vi "ACT Panel.vi"() -> ()   [LabVIEW 2013]
uses:
  Type Defs/Final Output for Dispaly 2.ctl
  Type Defs/Alt Control.ctl
  Type Defs/Alt Digit 100 New.ctl
  Type Defs/All Timers.ctl
  Type Defs/Timer Control.ctl
  Altitude/Altitude.xctl
  Type Defs/Action Time.ctl
  Mode Control/Mode.xctl
  Type Defs/Alt Display Large.ctl
  MSR/VertMode/VertMode.xctl
  Type Defs/Named Final Output name list with 02.ctl
  Type Defs/Named Final Output name list ordered.ctl
  MSR/MultiVal Buffer Xctl/Multivalue Buffer.xctl
  Type Defs/CO2 Settings.ctl
  Type Defs/Output Values.ctl
  Type Defs/Output Switches.ctl
  Type Defs/AD Settings.ctl
  <vilib>/Platform/TimedLoop/XDataNode/timing_clust.ctl
  <vilib>/Platform/TimedLoop/XDataNode/nitl_modes.ctl
  <vilib>/Platform/TimedLoop/XDataNode/wakeup.ctl
  <vilib>/Utility/miscctls.llb/LVPointTypeDef.ctl
  Type Defs/Data Reading.ctl
  File/File.lvclass
  Output Timer/Output Timer.lvclass
  <vilib>/Utility/config.llb/Read Key (I32).vi
  <vilib>/Utility/config.llb/Read Key (Double).vi
  <vilib>/Utility/config.llb/Read Key (Boolean).vi
  Output Timer/Set Delay.vi
  <vilib>/Utility/config.llb/Write Key (I32).vi
  <vilib>/Utility/config.llb/Write Key (Double).vi
  <vilib>/Utility/config.llb/Write Key (Boolean).vi
  <vilib>/Platform/TimedLoop/XDataNode/XDataNode.xnode
  <vilib>/Platform/TimedLoop/XDataNode/XDNodeRunTimeDep.lvlib
  <vilib>/ptbypt/NI_PtbyPt.lvlib
  <vilib>/Utility/config.llb/NI_LVConfig.lvlib
panel:
  out "sysStat":bool caption="System Status"
  in  "Main Tabs":T1(tab)=enum."Hypoxic CO2 Settings"
  in  "Close":bool
  in  "Other Outputs":cluster{"Alarm":bool, "Heater":bool}
  out "CO2 ppm":u32(slide)=493 scale=0.0..10000.0
  out "Alt Dif":dbl(slide)=1604.2180978990014 scale=-1000.0..1000.0 scale format="%.1f"
  out "Final Output":T2
  in  "hypCO2":T3={"Run C1"={"A-1,  1"=inf, "A-3,  2"=inf, "A-4, 3"=9600.0, "A-5, 4"=8800.0, "ABCD-7, 5"=9800.0, "A-8, 6"=9800.0, "B-1,  7"=3400.0, "B-3, 8"=3400.0, "B-4,  9"=9600.0, "B-5, 10"=8800.0, "B-8, 11"=9800.0, "C-1, 12"=1800.0, "C-3, 13"=1800.0, "C-4, 14"=9600.0, "C-5,  15"=8800.0, "C-8, 16"=9800.0, "D-1, 17"=inf, "D-3, 18"=inf, "D-4,  19"=3400.0, "D-5,  20"=1800.0, "D-8,  21"=9800.0}, "Run C2"={"A-1,  1"=inf, "A-3,  2"=inf, "A-4, 3"=9500.0, "A-5, 4"=8600.0, "ABCD-7, 5"=9700.0, "A-8, 6"=9700.0, "B-1,  7"=3000.0, "B-3, 8"=3000.0, "B-4,  9"=9500.0, "B-5, 10"=8600.0, "B-8, 11"=9700.0, "C-1, 12"=1400.0, "C-3, 13"=1400.0, "C-4, 14"=9500.0, "C-5,  15"=8600.0, "C-8, 16"=9700.0, "D-1, 17"=inf, "D-3, 18"=inf, "D-4,  19"=3000.0, "D-5,  20"=1400.0, "D-8,  21"=9700.0}, "Hold C3"={"A-1,  1"=1800.0, "A-3,  2"=1800.0, "A-4, 3"=9000.0, "A-5, 4"=8800.0, "ABCD-7, 5"=9800.0, "A-8, 6"=9800.0, "B-1,  7"=3400.0, "B-3, 8"=3400.0, "B-4,  9"=9000.0, "B-5, 10"=8800.0, "B-8, 11"=9800.0, "C-1, 12"=1800.0, "C-3, 13"=1800.0, "C-4, 14"=9000.0, "C-5,  15"=8800.0, "C-8, 16"=9800.0, "D-1, 17"=inf, "D-3, 18"=1800.0, "D-4,  19"=3400.0, "D-5,  20"=1800.0, "D-8,  21"=9800.0}, "Hold C4"={"A-1,  1"=1400.0, "A-3,  2"=1400.0, "A-4, 3"=8800.0, "A-5, 4"=8600.0, "ABCD-7, 5"=9700.0, "A-8, 6"=9700.0, "B-1,  7"=3000.0, "B-3, 8"=3000.0, "B-4,  9"=8800.0, "B-5, 10"=8600.0, "B-8, 11"=9700.0, "C-1, 12"=1400.0, "C-3, 13"=1400.0, "C-4, 14"=8800.0, "C-5,  15"=8600.0, "C-8, 16"=9700.0, "D-1, 17"=inf, "D-3, 18"=1400.0, "D-4,  19"=3000.0, "D-5,  20"=1400.0, "D-8,  21"=9700.0}, "High CO2 Forces"={"A-1, 1"=TRUE, "A-3, 2"=TRUE, "A-4, 3"=FALSE, "A-5, 4"=TRUE, "ABCD-7, 5"=FALSE, "A-8, 6"=TRUE, "B-1,  7"=TRUE, "B-3, 8"=TRUE, "B-4, 9"=FALSE, "B-5, 10"=TRUE, "B-8,  11"=TRUE, "C-1, 12"=TRUE, "C-3, 13"=TRUE, "C-4,  14"=FALSE, "C-5,  15"=TRUE, "C-8, 16"=TRUE, "D-1, 17"=TRUE, "D-3, 18"=TRUE, "D-4, 19"=TRUE, "D-5,  20"=TRUE, "D-8,  21"=TRUE}}
  in  "hypAD":T6={"Set Point Force"={"A-1,  1"=inf, "A-3,  2"=inf, "A-4, 3"=inf, "A-5, 4"=5790.0, "ABCD-7, 5"=inf, "A-8, 6"=inf, "B-1,  7"=5790.0, "B-3, 8"=5790.0, "B-4,  9"=inf, "B-5, 10"=5790.0, "B-8, 11"=inf, "C-1, 12"=inf, "C-3, 13"=inf, "C-4, 14"=inf, "C-5,  15"=5790.0, "C-8, 16"=inf, "D-1, 17"=inf, "D-3, 18"=inf, "D-4,  19"=5790.0, "D-5,  20"=5790.0, "D-8,  21"=inf}, "Run A1"={"A-1,  1"=inf, "A-3,  2"=inf, "A-4, 3"=3.0, "A-5, 4"=inf, "ABCD-7, 5"=67.0, "A-8, 6"=630.0, "B-1,  7"=-30.0, "B-3, 8"=-30.0, "B-4,  9"=3.0, "B-5, 10"=inf, "B-8, 11"=630.0, "C-1, 12"=-60.0, "C-3, 13"=-60.0, "C-4, 14"=3.0, "C-5,  15"=inf, "C-8, 16"=630.0, "D-1, 17"=inf, "D-3, 18"=inf, "D-4,  19"=-30.0, "D-5,  20"=-60.0, "D-8,  21"=630.0}, "Run A2"={"A-1,  1"=inf, "A-3,  2"=inf, "A-4, 3"=-3.0, "A-5, 4"=inf, "ABCD-7, 5"=60.0, "A-8, 6"=610.0, "B-1,  7"=-100.0, "B-3, 8"=-100.0, "B-4,  9"=-3.0, "B-5, 10"=inf, "B-8, 11"=610.0, "C-1, 12"=-120.0, "C-3, 13"=-120.0, "C-4, 14"=-3.0, "C-5,  15"=inf, "C-8, 16"=610.0, "D-1, 17"=inf, "D-3, 18"=inf, "D-4,  19"=-100.0, "D-5,  20"=-120.0, "D-8,  21"=610.0}, "Hold A3"={"A-1,  1"=0.0, "A-3,  2"=0.0, "A-4, 3"=3.0, "A-5, 4"=inf, "ABCD-7, 5"=67.0, "A-8, 6"=630.0, "B-1,  7"=-150.0, "B-3, 8"=-150.0, "B-4,  9"=3.0, "B-5, 10"=inf, "B-8, 11"=630.0, "C-1, 12"=-300.0, "C-3, 13"=-300.0, "C-4, 14"=3.0, "C-5,  15"=inf, "C-8, 16"=630.0, "D-1, 17"=inf, "D-3, 18"=0.0, "D-4,  19"=-150.0, "D-5,  20"=-300.0, "D-8,  21"=630.0}, "Hold A4"={"A-1,  1"=-150.0, "A-3,  2"=-150.0, "A-4, 3"=-3.0, "A-5, 4"=inf, "ABCD-7, 5"=60.0, "A-8, 6"=610.0, "B-1,  7"=-250.0, "B-3, 8"=-250.0, "B-4,  9"=-3.0, "B-5, 10"=inf, "B-8, 11"=610.0, "C-1, 12"=-500.0, "C-3, 13"=-500.0, "C-4, 14"=-3.0, "C-5,  15"=inf, "C-8, 16"=610.0, "D-1, 17"=inf, "D-3, 18"=-150.0, "D-4,  19"=-250.0, "D-5,  20"=-500.0, "D-8,  21"=610.0}, "High AD Diff "={"A-1, 1"=FALSE, "A-3, 2"=FALSE, "A-4, 3"=FALSE, "A-5, 4"=TRUE, "ABCD-7, 5"=FALSE, "A-8, 6"=TRUE, "B-1,  7"=FALSE, "B-3, 8"=FALSE, "B-4, 9"=FALSE, "B-5, 10"=TRUE, "B-8,  11"=TRUE, "C-1, 12"=FALSE, "C-3, 13"=FALSE, "C-4,  14"=FALSE, "C-5,  15"=TRUE, "C-8, 16"=TRUE, "D-1, 17"=FALSE, "D-3, 18"=FALSE, "D-4, 19"=FALSE, "D-5,  20"=FALSE, "D-8,  21"=TRUE}, "Delay S"={"A-1,  1"=30.0, "A-3,  2"=30.0, "A-4, 3"=1.0, "A-5, 4"=1.0, "ABCD-7, 5"=1.0, "A-8, 6"=1.0, "B-1,  7"=30.0, "B-3, 8"=30.0, "B-4,  9"=1.0, "B-5, 10"=1.0, "B-8, 11"=1.0, "C-1, 12"=30.0, "C-3, 13"=30.0, "C-4, 14"=1.0, "C-5,  15"=1.0, "C-8, 16"=1.0, "D-1, 17"=1.0, "D-3, 18"=30.0, "D-4,  19"=30.0, "D-5,  20"=30.0, "D-8,  21"=1.0}}
  in  "hyperCO2":T3={"Run C1"={"A-1,  1"=inf, "A-3,  2"=inf, "A-4, 3"=9600.0, "A-5, 4"=8800.0, "ABCD-7, 5"=9800.0, "A-8, 6"=9800.0, "B-1,  7"=3400.0, "B-3, 8"=3400.0, "B-4,  9"=9600.0, "B-5, 10"=8800.0, "B-8, 11"=9800.0, "C-1, 12"=1800.0, "C-3, 13"=1800.0, "C-4, 14"=9600.0, "C-5,  15"=8800.0, "C-8, 16"=9800.0, "D-1, 17"=inf, "D-3, 18"=inf, "D-4,  19"=3400.0, "D-5,  20"=1800.0, "D-8,  21"=9800.0}, "Run C2"={"A-1,  1"=inf, "A-3,  2"=inf, "A-4, 3"=9500.0, "A-5, 4"=8600.0, "ABCD-7, 5"=9700.0, "A-8, 6"=9700.0, "B-1,  7"=3000.0, "B-3, 8"=3000.0, "B-4,  9"=9500.0, "B-5, 10"=8600.0, "B-8, 11"=9700.0, "C-1, 12"=1400.0, "C-3, 13"=1400.0, "C-4, 14"=9500.0, "C-5,  15"=8600.0, "C-8, 16"=9700.0, "D-1, 17"=inf, "D-3, 18"=inf, "D-4,  19"=3000.0, "D-5,  20"=1400.0, "D-8,  21"=9700.0}, "Hold C3"={"A-1,  1"=1800.0, "A-3,  2"=1800.0, "A-4, 3"=9000.0, "A-5, 4"=8800.0, "ABCD-7, 5"=9800.0, "A-8, 6"=9800.0, "B-1,  7"=3400.0, "B-3, 8"=3400.0, "B-4,  9"=9000.0, "B-5, 10"=8800.0, "B-8, 11"=9800.0, "C-1, 12"=1800.0, "C-3, 13"=1800.0, "C-4, 14"=9000.0, "C-5,  15"=8800.0, "C-8, 16"=9800.0, "D-1, 17"=inf, "D-3, 18"=1800.0, "D-4,  19"=3400.0, "D-5,  20"=1800.0, "D-8,  21"=9800.0}, "Hold C4"={"A-1,  1"=1400.0, "A-3,  2"=1400.0, "A-4, 3"=8800.0, "A-5, 4"=8600.0, "ABCD-7, 5"=9700.0, "A-8, 6"=9700.0, "B-1,  7"=3000.0, "B-3, 8"=3000.0, "B-4,  9"=8800.0, "B-5, 10"=8600.0, "B-8, 11"=9700.0, "C-1, 12"=1400.0, "C-3, 13"=1400.0, "C-4, 14"=8800.0, "C-5,  15"=8600.0, "C-8, 16"=9700.0, "D-1, 17"=inf, "D-3, 18"=1400.0, "D-4,  19"=3000.0, "D-5,  20"=1400.0, "D-8,  21"=9700.0}, "High CO2 Forces"={"A-1, 1"=TRUE, "A-3, 2"=TRUE, "A-4, 3"=FALSE, "A-5, 4"=TRUE, "ABCD-7, 5"=FALSE, "A-8, 6"=TRUE, "B-1,  7"=TRUE, "B-3, 8"=TRUE, "B-4, 9"=FALSE, "B-5, 10"=TRUE, "B-8,  11"=TRUE, "C-1, 12"=TRUE, "C-3, 13"=TRUE, "C-4,  14"=FALSE, "C-5,  15"=TRUE, "C-8, 16"=TRUE, "D-1, 17"=TRUE, "D-3, 18"=TRUE, "D-4, 19"=TRUE, "D-5,  20"=TRUE, "D-8,  21"=TRUE}}
  in  "hyperAD":T6={"Set Point Force"={"A-1,  1"=inf, "A-3,  2"=inf, "A-4, 3"=inf, "A-5, 4"=5790.0, "ABCD-7, 5"=inf, "A-8, 6"=inf, "B-1,  7"=5790.0, "B-3, 8"=5790.0, "B-4,  9"=inf, "B-5, 10"=5790.0, "B-8, 11"=inf, "C-1, 12"=inf, "C-3, 13"=inf, "C-4, 14"=inf, "C-5,  15"=5790.0, "C-8, 16"=inf, "D-1, 17"=inf, "D-3, 18"=inf, "D-4,  19"=5790.0, "D-5,  20"=5790.0, "D-8,  21"=inf}, "Run A1"={"A-1,  1"=inf, "A-3,  2"=inf, "A-4, 3"=3.0, "A-5, 4"=inf, "ABCD-7, 5"=67.0, "A-8, 6"=630.0, "B-1,  7"=-30.0, "B-3, 8"=-30.0, "B-4,  9"=3.0, "B-5, 10"=inf, "B-8, 11"=630.0, "C-1, 12"=-60.0, "C-3, 13"=-60.0, "C-4, 14"=3.0, "C-5,  15"=inf, "C-8, 16"=630.0, "D-1, 17"=inf, "D-3, 18"=inf, "D-4,  19"=-30.0, "D-5,  20"=-60.0, "D-8,  21"=630.0}, "Run A2"={"A-1,  1"=inf, "A-3,  2"=inf, "A-4, 3"=-3.0, "A-5, 4"=inf, "ABCD-7, 5"=60.0, "A-8, 6"=610.0, "B-1,  7"=-100.0, "B-3, 8"=-100.0, "B-4,  9"=-3.0, "B-5, 10"=inf, "B-8, 11"=610.0, "C-1, 12"=-120.0, "C-3, 13"=-120.0, "C-4, 14"=-3.0, "C-5,  15"=inf, "C-8, 16"=610.0, "D-1, 17"=inf, "D-3, 18"=inf, "D-4,  19"=-100.0, "D-5,  20"=-120.0, "D-8,  21"=610.0}, "Hold A3"={"A-1,  1"=0.0, "A-3,  2"=0.0, "A-4, 3"=3.0, "A-5, 4"=inf, "ABCD-7, 5"=67.0, "A-8, 6"=630.0, "B-1,  7"=-150.0, "B-3, 8"=-150.0, "B-4,  9"=3.0, "B-5, 10"=inf, "B-8, 11"=630.0, "C-1, 12"=-300.0, "C-3, 13"=-300.0, "C-4, 14"=3.0, "C-5,  15"=inf, "C-8, 16"=630.0, "D-1, 17"=inf, "D-3, 18"=0.0, "D-4,  19"=-150.0, "D-5,  20"=-300.0, "D-8,  21"=630.0}, "Hold A4"={"A-1,  1"=-150.0, "A-3,  2"=-150.0, "A-4, 3"=-3.0, "A-5, 4"=inf, "ABCD-7, 5"=60.0, "A-8, 6"=610.0, "B-1,  7"=-250.0, "B-3, 8"=-250.0, "B-4,  9"=-3.0, "B-5, 10"=inf, "B-8, 11"=610.0, "C-1, 12"=-500.0, "C-3, 13"=-500.0, "C-4, 14"=-3.0, "C-5,  15"=inf, "C-8, 16"=610.0, "D-1, 17"=inf, "D-3, 18"=-150.0, "D-4,  19"=-250.0, "D-5,  20"=-500.0, "D-8,  21"=610.0}, "High AD Diff "={"A-1, 1"=FALSE, "A-3, 2"=FALSE, "A-4, 3"=FALSE, "A-5, 4"=TRUE, "ABCD-7, 5"=FALSE, "A-8, 6"=TRUE, "B-1,  7"=FALSE, "B-3, 8"=FALSE, "B-4, 9"=FALSE, "B-5, 10"=TRUE, "B-8,  11"=TRUE, "C-1, 12"=FALSE, "C-3, 13"=FALSE, "C-4,  14"=FALSE, "C-5,  15"=TRUE, "C-8, 16"=TRUE, "D-1, 17"=FALSE, "D-3, 18"=FALSE, "D-4, 19"=FALSE, "D-5,  20"=FALSE, "D-8,  21"=TRUE}, "Delay S"={"A-1,  1"=30.0, "A-3,  2"=30.0, "A-4, 3"=1.0, "A-5, 4"=1.0, "ABCD-7, 5"=1.0, "A-8, 6"=1.0, "B-1,  7"=30.0, "B-3, 8"=30.0, "B-4,  9"=1.0, "B-5, 10"=1.0, "B-8, 11"=1.0, "C-1, 12"=30.0, "C-3, 13"=30.0, "C-4, 14"=1.0, "C-5,  15"=1.0, "C-8, 16"=1.0, "D-1, 17"=1.0, "D-3, 18"=30.0, "D-4,  19"=30.0, "D-5,  20"=30.0, "D-8,  21"=1.0}}
  in  "Main States":T7(tab)
  out "altDisp1":dbl format="%#.0f"
  out "altDisp1 2":dbl format="%#.0f"
  out "Heading 3":string="Current Effective Altitude in  Feet"
  in  "Mode 1":enum8{"Off", "Stby", "Hold", "Run"}(xcontrol)=enum."Stby"
  in  "Confirm Now 2":bool
  out "CO2_1":sgl caption="Carbon Dioxide  %" format="%.3f"
  in  "ALT SET 2":T8 {"Alt Digit 100" min=0 max=9 step=1; "Alt Digit 100" min=0 max=9 step=1; "Alt Digit 100" min=0 max=9 step=1; "Alt Digit 100" min=0 max=9 step=1; "Alt Digit 100" min=0 max=9 step=1}
  out "altDisp2":T10 caption="ALT DISPLAY 2" format="%#.0f"
  out "Heading 2":string="Current Effective Altitude in  Feet"
  in  "dimmer":i8(slide) scale=0.0..100.0
  out "CO2Buffer":cluster{"Time":timestamp, "Val":dbl[]}(xcontrol)
  out "pAltitude":cluster{"Time":timestamp, "Val":dbl[]}(xcontrol)
  out "Temp C":sgl=26.28
  out "Press mB":sgl=833.25
  out "CO2_0":sgl=0.0493 caption="CO2%\n %" format="%.3g"
  in  "Confirm Now":bool
  in  "ALT SET":T8 {"Alt Digit 100" min=0 max=9 step=1; "Alt Digit 100" min=0 max=9 step=1; "Alt Digit 100" min=0 max=9 step=1; "Alt Digit 100" min=0 max=9 step=1; "Alt Digit 100" min=0 max=9 step=1}
  out "Altitude":sgl format="%#.0f"
  out "O2%":sgl=20.9793 format="%.1f"
  out "Units":string="F\ne\ne\nt"
  in  "Mode":enum8{"Off", "Stby", "Hold", "Run"}(xcontrol)=enum."Stby"
  out "Final  Output Names":T11={"A-1,  1"="Main", "A-3,  2"="Main", "A-4, 3"="Recircirculation", "A-5, 4"="Scrubber", "A-7, 5"="Oxygen", "A-8, 6"="Vent", "B-1,  7"="Boost A", "B-3, 8"="Boost A", "B-4,  9"="Recircirculation", "B-5, 10"="Scrubber", "B-8, 11"="Vent", "C-1, 12"="Boost B", "C-3, 13"="Boost B", "C-4, 14"="Recircirculation", "C-5,  15"="Scrubber", "C-8, 16"="Vent", "D-1, 17"="Main", "D-3, 18"="Boost A", "D-4,  19"="Boost B", "D-5,  20"="Vent", "D-8,  21"="Vent 2", "B-7"="Oxygen", "C-7"="Oxygen", "D-7"="Oxygen", "A-1"=FALSE, "A-3"=FALSE, "A-4"=FALSE, "A-5"=FALSE, "A-7"=FALSE, "A-8"=FALSE, "B-1"=FALSE, "B-3"=FALSE, "B-4"=FALSE, "B-5"=FALSE, "B-7"=FALSE, "B-8"=FALSE, "C-1"=FALSE, "C-3"=FALSE, "C-4"=FALSE, "C-5"=FALSE, "C-7"=FALSE, "C-8"=FALSE, "D-1"=FALSE, "D-3"=FALSE, "D-4"=FALSE, "D-5"=FALSE, "D-7"=FALSE, "D-8"=FALSE}
  out "Time":timestamp caption="Controller\nTime" format="%<%H:%M:%S\n%m/%d/%y>T"
  in  "Timers":T12 {"Timer 4"."Action Time" format="%<%H:%M>t"; "Timer 3"."Action Time" format="%<%H:%M>t"; "Timer 2"."Action Time" format="%<%H:%M>t"; "Timer"."Action Time" format="%<%H:%M>t"}
  in  "Shutdown":bool
  out "maxO2":dbl caption="Max O2" format="%.1f"
  out "minAlt":dbl caption="Minimum Altitude"
  out "onBatt":bool caption="Plugged in?"
  out "estBattLeft":u8(slide) caption="Estimated Battery Life" scale=0.0..100.0
  in  "eCode":bool
  in  "silence":bool
  out "senseConn":bool caption="Sensor Connection"
  out "High O2 Level":bool
  out "Altitude":bool
  out "Low O2 Level":bool
  out "CO2 Level":bool
  in  "writetofile":bool
  out "Sensor Error":bool
  out "Calibrate":bool
  out "meanDiff":dbl caption="Mean O2 Difference"
  out "Calibrating":bool
  in  "Enter or Exit Setup":bool
  in  "reset":bool
  in  "Set Point Alt":i32 min=0 max=10000 step=1
  in  "Level 0":T15 {"Time Offset (h)" min=-12.0 max=12.0 step=1.0}
  in  "Level 1":T16
  in  "Level 2":T17
  in  "Level 3":T19={"Final  Output Names "={"A-1, 1"="Main", "A-3, 2"="Main", "A-4, 3"="Recircirculation", "A-5, 4"="Scrubber", "A-7, 5"="Oxygen", "A-8, 6"="Vent", "B-1,  7"="Boost A", "B-3, 8"="Boost A", "B-4, 9"="Recircirculation", "B-5, 10"="Scrubber", "B-8, 11"="Vent", "C-1, 12"="Boost B", "C-3, 13"="Boost B", "C-4, 14"="Recircirculation", "C-5,  15"="Scrubber", "C-8, 16"="Vent", "D-1, 17"="Main", "D-3, 18"="Boost A", "D-4,  19"="Boost B", "D-5,  20"="Vent", "D-8,  21"="Vent 2"}, " Setup Tables Visible"=FALSE, "Load Names"=FALSE, "Save Names"=FALSE, "maxAltSP"=0.0, "Alarm Points"={"CalLimit"=500.0, "SenseLimit"=1000.0, "CO2Lim"=1.0, "AltLim"=100000.0, "O2 Low"=100.0, "O2 High"=100.0}, "Stop"=FALSE, "O2-1 (%)"=0.0, "O2-2 (%)"=0.0, "Buffer"=0.0} {"Buffer" min=0.0 max=1.0 format="%7.4f"; "O2-2 (%)" format="%7.4f"; "O2-1 (%)" format="%7.4f"}
  out "SN#":string
  out "Version":string
  out "locElev":dbl=1449.1019287109375 caption="Pressure Compensated \nLocal Elevation"
  out "altSp":dbl
  out "codelapse":bool
  # "Channel A"
  # "Channel B"
  # "Channel C"
  # "Channel D"
  # "Channel A"
  # "Channel B"
  # "Channel C"
  # "Channel D"
  # "1"
  # "1"
  # "1"
  # "1"
  # "CAT v153"
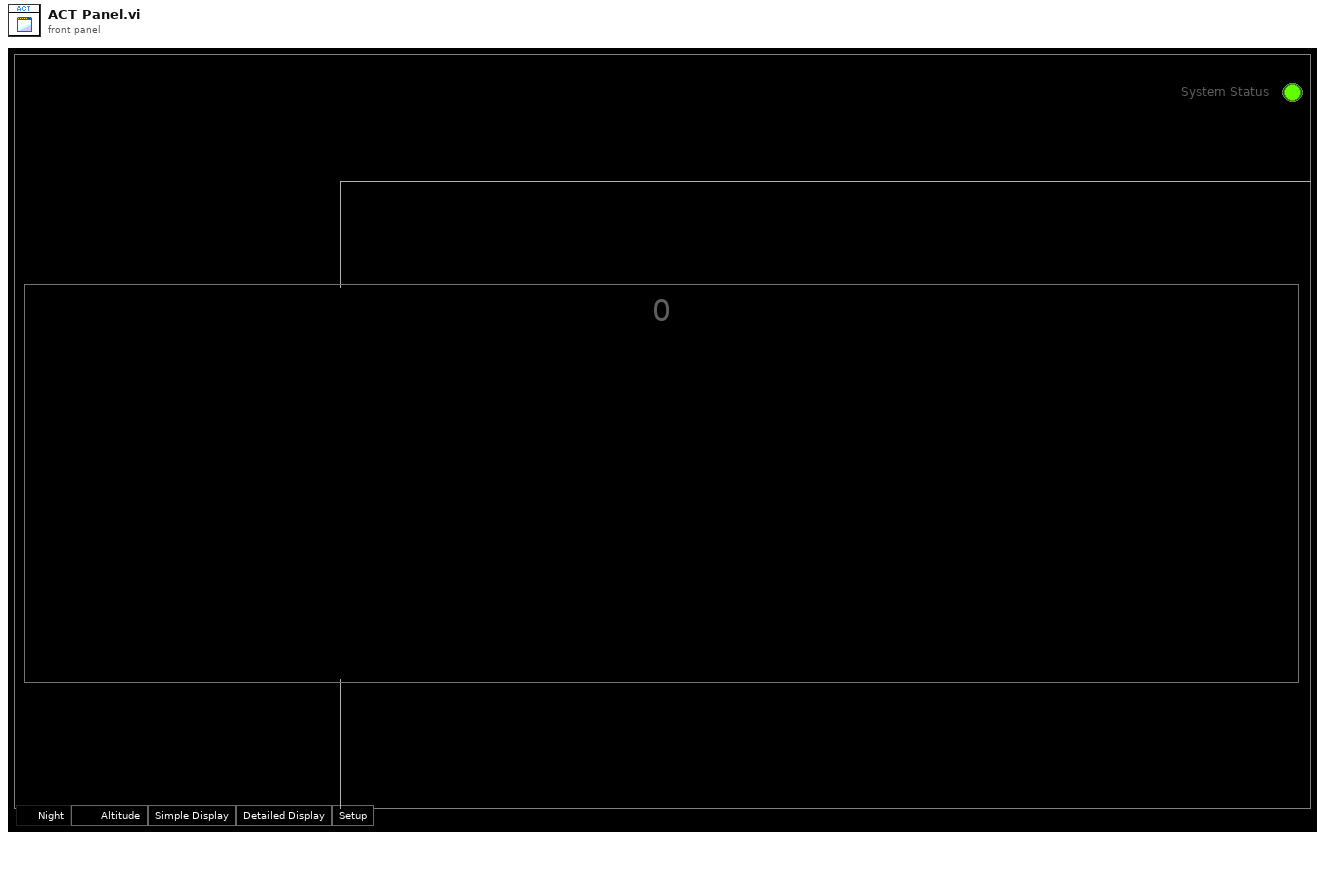
[diagram p1: front panel]
types:
  T1 = enum32{"Inputs and Controls", "CO2 and AD Outputs", "Hypoxic CO2 Settings", "Hypoxic AD Settings", "Hyperoxic CO2 Settings", "Hyperoxic AD Settings"}
  T2 = typedef "Final Output for Dispaly 2.ctl" = cluster{"A-1,  1":bool, "A-3,  2":bool, "A-4, 3":bool, "A-5, 4":bool, "ABCD-7, 5":bool, "A-8, 6":bool, "B-1,  7":bool, "B-3, 8":bool, "B-4,  9":bool, "B-5, 10":bool, "B-8, 11":bool, "C-1, 12":bool, "C-3, 13":bool, "C-4, 14":bool, "C-5,  15":bool, "C-8, 16":bool, "D-1, 17":bool, "D-3, 18":bool, "D-4,  19":bool, "D-5,  20":bool, "D-8,  21":bool}
  T3 = typedef "CO2 Settings.ctl" = cluster{"Run C1":T4, "Run C2":T4, "Hold C3":T4, "Hold C4":T4, "High CO2 Forces":T5}
  T4 = typedef "Output Values.ctl" = cluster{"A-1,  1":dbl, "A-3,  2":dbl, "A-4, 3":dbl, "A-5, 4":dbl, "ABCD-7, 5":dbl, "A-8, 6":dbl, "B-1,  7":dbl, "B-3, 8":dbl, "B-4,  9":dbl, "B-5, 10":dbl, "B-8, 11":dbl, "C-1, 12":dbl, "C-3, 13":dbl, "C-4, 14":dbl, "C-5,  15":dbl, "C-8, 16":dbl, "D-1, 17":dbl, "D-3, 18":dbl, "D-4,  19":dbl, "D-5,  20":dbl, "D-8,  21":dbl}
  T5 = typedef "Output Switches.ctl" = cluster{"A-1, 1":bool, "A-3, 2":bool, "A-4, 3":bool, "A-5, 4":bool, "ABCD-7, 5":bool, "A-8, 6":bool, "B-1,  7":bool, "B-3, 8":bool, "B-4, 9":bool, "B-5, 10":bool, "B-8,  11":bool, "C-1, 12":bool, "C-3, 13":bool, "C-4,  14":bool, "C-5,  15":bool, "C-8, 16":bool, "D-1, 17":bool, "D-3, 18":bool, "D-4, 19":bool, "D-5,  20":bool, "D-8,  21":bool}
  T6 = typedef "AD Settings.ctl" = cluster{"Set Point Force":T4, "Run A1":T4, "Run A2":T4, "Hold A3":T4, "Hold A4":T4, "High AD Diff ":T5, "Delay S":T4}
  T7 = enum32{"     Night", "       Altitude ", "Simple Display", "Detailed Display", "Timers", "Setup"}
  T8 = typedef "Alt Control.ctl" = cluster{"Alt Digit 100":T9, "Alt Digit 100":T9, "Alt Digit 100":T9, "Alt Digit 100":T9, "Alt Digit 100":T9}
  T9 = typedef "Alt Digit 100 New.ctl" = i8
  T10 = typedef "Alt Display Large.ctl" = sgl
  T11 = typedef "Named Final Output name list with 02.ctl" = cluster{"A-1,  1":string, "A-3,  2":string, "A-4, 3":string, "A-5, 4":string, "A-7, 5":string, "A-8, 6":string, "B-1,  7":string, "B-3, 8":string, "B-4,  9":string, "B-5, 10":string, "B-8, 11":string, "C-1, 12":string, "C-3, 13":string, "C-4, 14":string, "C-5,  15":string, "C-8, 16":string, "D-1, 17":string, "D-3, 18":string, "D-4,  19":string, "D-5,  20":string, "D-8,  21":string, "B-7":string, "C-7":string, "D-7":string, "A-1":bool, "A-3":bool, "A-4":bool, "A-5":bool, "A-7":bool, "A-8":bool, "B-1":bool, "B-3":bool, "B-4":bool, "B-5":bool, "B-7":bool, "B-8":bool, "C-1":bool, "C-3":bool, "C-4":bool, "C-5":bool, "C-7":bool, "C-8":bool, "D-1":bool, "D-3":bool, "D-4":bool, "D-5":bool, "D-7":bool, "D-8":bool}
  T12 = typedef "All Timers.ctl" = cluster{"Timer":T13, "Timer 2":T13, "Timer 3":T13, "Timer 4":T13}
  T13 = typedef "Timer Control.ctl" = cluster{"Sun":bool, "Timer":bool, "Altitude":sgl, "Action Time":T14, "Mon":bool, "Tues":bool, "Wed":bool, "Thur":bool, "Fri":bool, "Sat":bool, "Mode":enum8{"Off", "Stby", "Hold", "Run"}}
  T14 = typedef "Action Time.ctl" = dbl
  T15 = cluster{"Time Offset (h)":dbl, "Demo Mode?":bool}
  T16 = cluster{"ALT Window ON/OFF":bool, "Feet OFF/ Meters ON":bool}
  T17 = cluster{"West ON/Std OFF":bool, "Enter Calibration":bool, "Max Altitude":dbl, "Alt Points":u32, "CO2 Points":u32}
  T18 = typedef "Named Final Output name list ordered.ctl" = cluster{"A-1, 1":string, "A-3, 2":string, "A-4, 3":string, "A-5, 4":string, "A-7, 5":string, "A-8, 6":string, "B-1,  7":string, "B-3, 8":string, "B-4, 9":string, "B-5, 10":string, "B-8, 11":string, "C-1, 12":string, "C-3, 13":string, "C-4, 14":string, "C-5,  15":string, "C-8, 16":string, "D-1, 17":string, "D-3, 18":string, "D-4,  19":string, "D-5,  20":string, "D-8,  21":string}
  T19 = cluster{"Final  Output Names ":T18, " Setup Tables Visible":bool, "Load Names":bool, "Save Names":bool, "maxAltSP":sgl, "Alarm Points":cluster{"CalLimit":sgl, "SenseLimit":sgl, "CO2Lim":sgl, "AltLim":sgl, "O2 Low":sgl, "O2 High":sgl}, "Stop":bool, "O2-1 (%)":dbl, "O2-2 (%)":dbl, "Buffer":dbl}
  T20 = typedef "LVPointTypeDef.ctl" = cluster{"Horizontal":i16, "Vertical":i16}
  T21 = cluster{"Heading":string, "Altitude":dbl, "Visible?":bool}
  T22 = typedef "XDNodeRunTimeDep.lvlib/timing_clust.ctl" = cluster{"Expected End [f-1]":u64, "Actual End [f-1]":u64, "Finished Late? [f-1]":bool, "Expected End [i-1]":u64, "Actual End [i-1]":u64, "Finished Late? [i-1]":bool, "Expected Start [i]":u64, "Actual Start [i]":u64, "Expected Start [f]":u64, "Actual Start [f]":u64, "Source Name":string, "Structure Name":string, "Period":i64, "Deadline":i64, "Offset":i64, "Start":i64, "Priority":i32, "Timeout":i32, "Mode":T23, "Wakeup Reason":T24, "Error":errorcluster, "Source Type":string, "Secondary Source Type":string, "Global End Time":u64, "Global Start Time":u64, "Frame Duration":u64, "Iteration Duration":u64, "Assigned CPU":i32, "I/O Scan Engine Mode":u32}
  T23 = typedef "XDNodeRunTimeDep.lvlib/nitl_modes.ctl" = enum32{"No Change", "Process missed periods, maintain original phase", "Discard missed periods, maintain original phase", "Process missed periods, ignore original phase", "Discard missed periods, ignore original phase"}
  T24 = typedef "XDNodeRunTimeDep.lvlib/wakeup.ctl" = enum32{"Normal", "Aborted", "Asynchronous wakeup", "Timing source error", "Timed loop error", "Timeout"}
  T25 = enum32{"Invalid", "Standard", "Closed", "Hidden", "Minimized", "Maximized"}
  T26 = typedef "Data Reading.ctl" = cluster{"Date":string, "Time":string, "CO2- ppm":u32, "Last Ctrl Word":u32, "O2-1 ppm":u32, "O2-2 ppm":u32, "Temp MB":sgl, "Temp Sensor Module":sgl, "Press mB":sgl}
  T27 = typedef "NI_LVConfig.lvlib/Config Data RefNum.ctl" = refnum<k1>
  T28 = enum8{"Enabled", "Disabled", "Disabled and Grayed Out"}
  T29 = cluster{"[0]":i8, "[1]":i8, "[2]":i8, "[3]":i8, "[4]":i8}
  T30 = cluster{"Level 1 Password":string, "Level 2 Password":string, "Level 3 Password":string}
  T31 = cluster{"CalLimit":dbl, "SenseLimit":dbl, "CO2Lim":dbl, "AltLim":dbl, "O2 Low":dbl, "O2 High":dbl}
  T32 = cluster{"Pointers":i32[], "Dates":dbl[], "Keys":string[], "Key Valid?":bool[], "Date Exceeded":bool[]}
  T33 = typedef "LVRectTypeDef.ctl" = cluster{"Left":i16, "Top":i16, "Right":i16, "Bottom":i16}
  T34 = cluster{"Mode":refnum<vi>, "ALT SET":refnum<vi>, "Confirm Now":refnum<vi>}
  T35 = cluster{"Main 1":bool, "Main 2":bool, "Recirc  3":bool, "Boost A 7":bool, "Recirc  9":bool, "Scrub 4":bool, "Scrub 10":bool, "O2 5":bool, "Vent 6":bool, "Boost A 8":bool, "Vent 11":bool, "Boost B 12":bool, "Boost B 13":bool, "Recirc 14":bool, "Scrub 15":bool, "Vent 16":bool, "Main 17":bool, "Boost A 18":bool, "Boost B 19":bool, "Boost F 20":bool, "Vent 2 21":bool}
  T36 = cluster{"A-1,  1":bool, "A-3,  2":bool, "A-4, 3":bool, "A-5, 4":bool, "ABCD-7, 5":bool, "A-8, 6":bool, "B-1,  7":bool, "B-3, 8":bool, "B-4,  9":bool, "B-5, 10":bool, "B-8, 11":bool, "C-1, 12":bool, "C-3, 13":bool, "C-4, 14":bool, "C-5,  15":bool, "C-8, 16":bool, "D-1, 17":bool, "D-3, 18":bool, "D-4,  19":bool, "D-5,  20":bool, "D-8,  21":bool}
  T37 = cluster{bool, bool, bool, bool, bool, bool, bool, bool, bool, bool, bool, bool, bool, bool, bool, bool, bool, bool, bool, bool, bool}
  T38 = cluster{"[0]":bool, "[1]":bool, "[2]":bool, "[3]":bool, "[4]":bool, "[5]":bool, "[6]":bool, "[7]":bool, "[8]":bool, "[9]":bool, "[10]":bool, "[11]":bool, "[12]":bool, "[13]":bool, "[14]":bool, "[15]":bool, "[16]":bool, "[17]":bool, "[18]":bool, "[19]":bool, "[20]":bool}
  T39 = cluster{"Date":string, "Time":string, "CO2- ppm":u32, "Last Ctrl Word":u32, "O2-1 ppm":u32, "O2-2 ppm":u32, "Temp MB":sgl, "Temp Sensor Module":sgl, "Press mB":sgl}
  T40 = cluster{"Set Point Force":T4, "Run A1":T4, "Run A2":T4, "Hold A3":T4, "Hold A4":T4}
  T41 = cluster{"Set Point Force":T4, "Run A1":T4, "Run A2":T4, "Hold A3":T4, "Hold A4":T4, "AltLim":sgl, "Set Point Alt":i32, "Value":sgl, "Value":dbl}
  T42 = cluster{"Set Point Force":T4, "Run A1":T4, "Run A2":T4, "Hold A3":T4, "Hold A4":T4, "AltLim":dbl, "Set Point Alt":dbl, "Value":dbl, "Value":dbl}
  T43 = cluster{"CalLimit":sgl, "SenseLimit":sgl, "CO2Lim":sgl, "AltLim":sgl, "O2 Low":sgl, "O2 High":sgl}
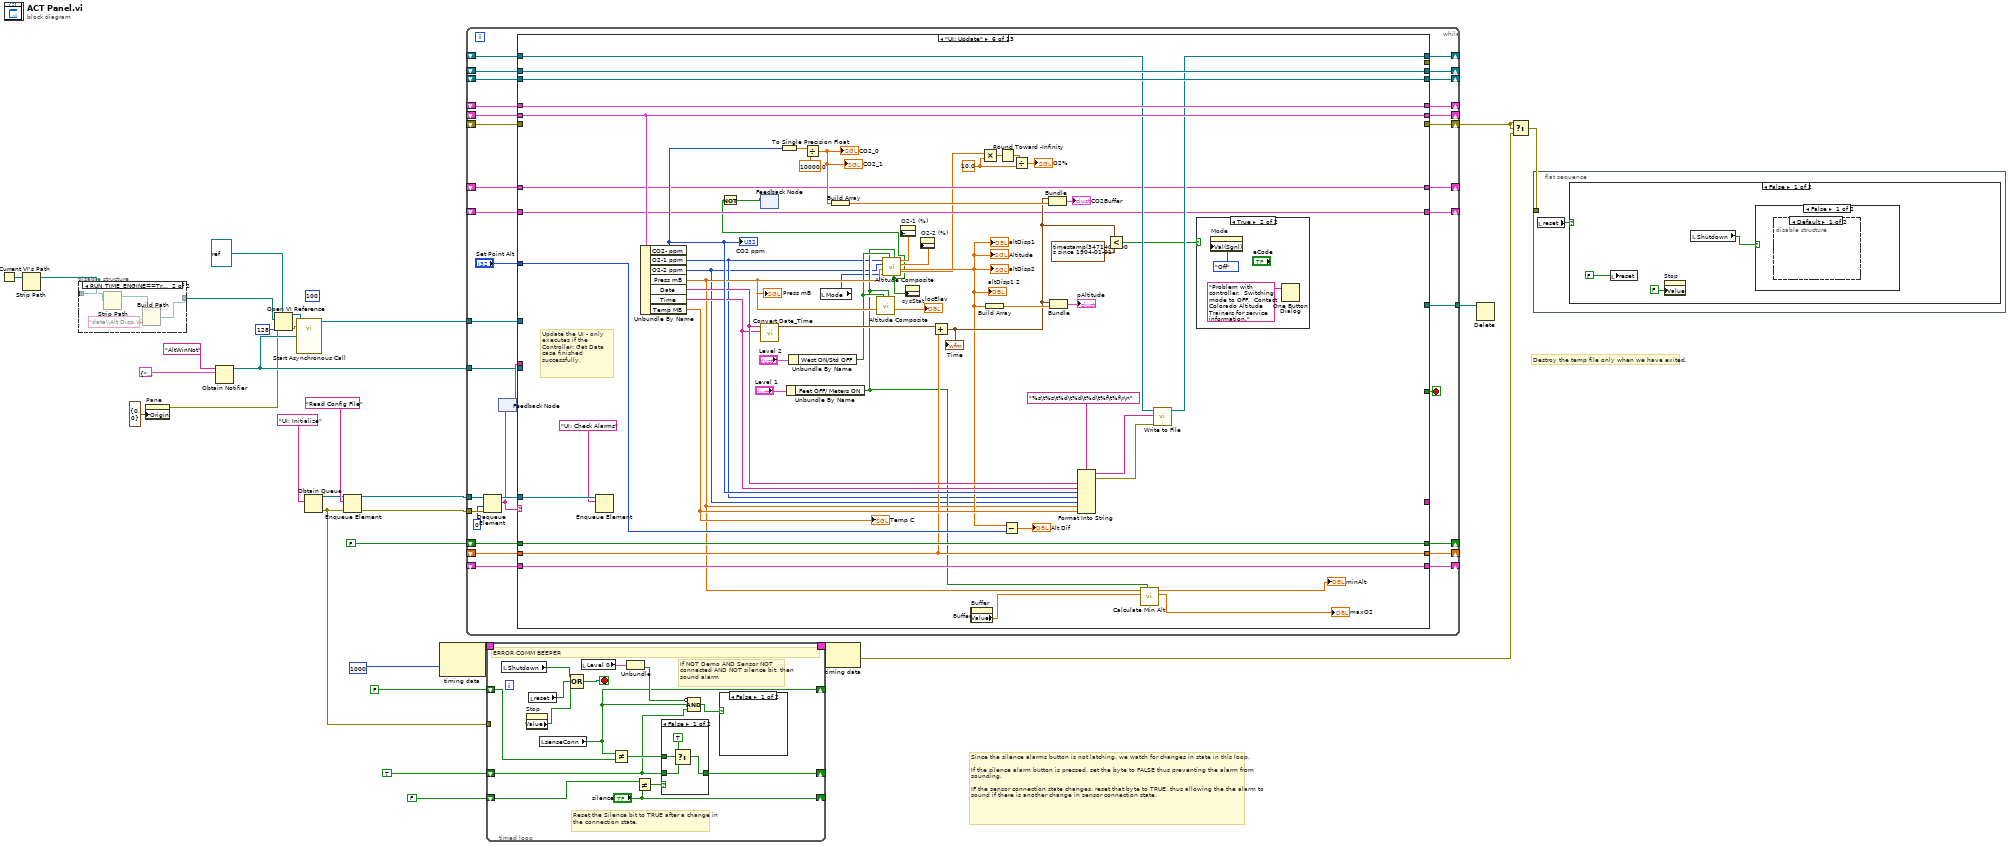
[diagram p0: block diagram]
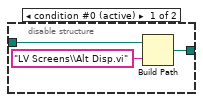
[diagram p2: hidden frame]
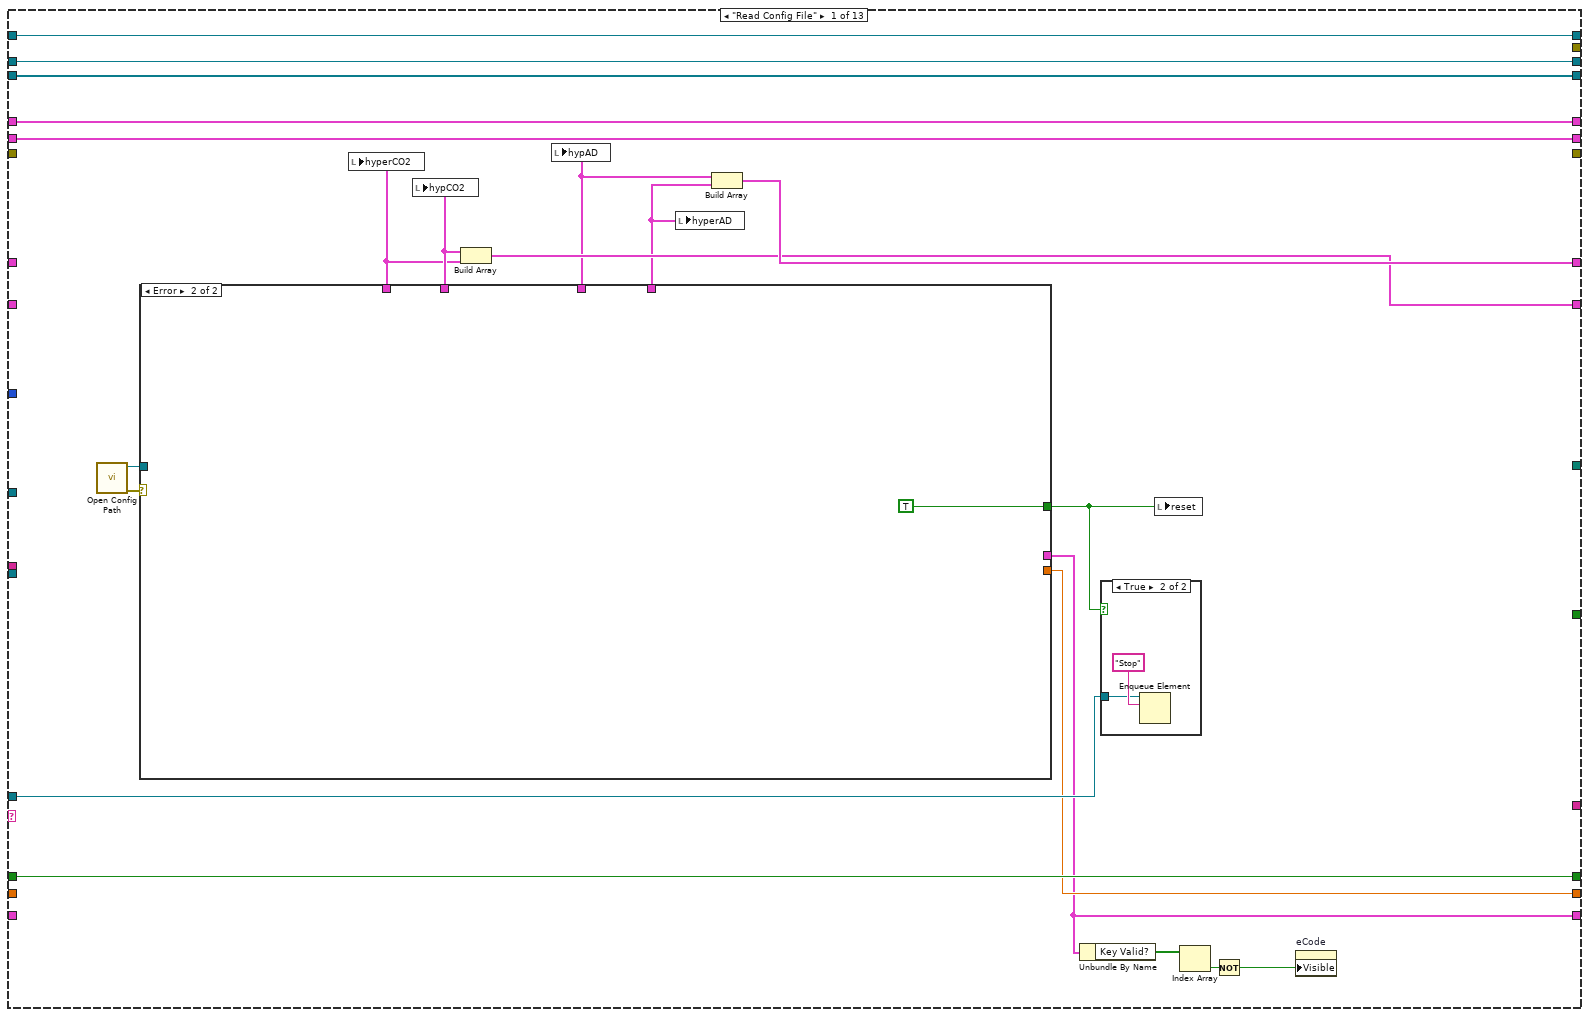
[diagram p3: hidden frame]
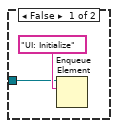
[diagram p4: hidden frame]
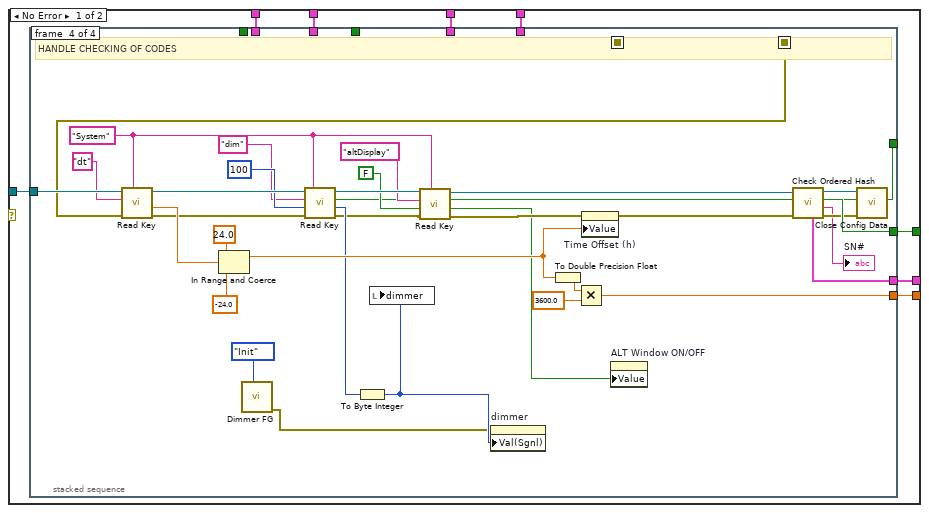
[diagram p5: hidden frame]
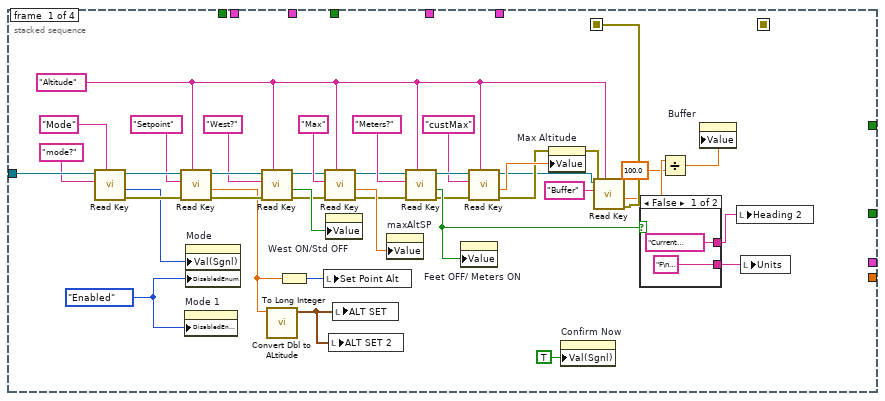
[diagram p6: hidden frame]
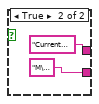
[diagram p7: hidden frame]
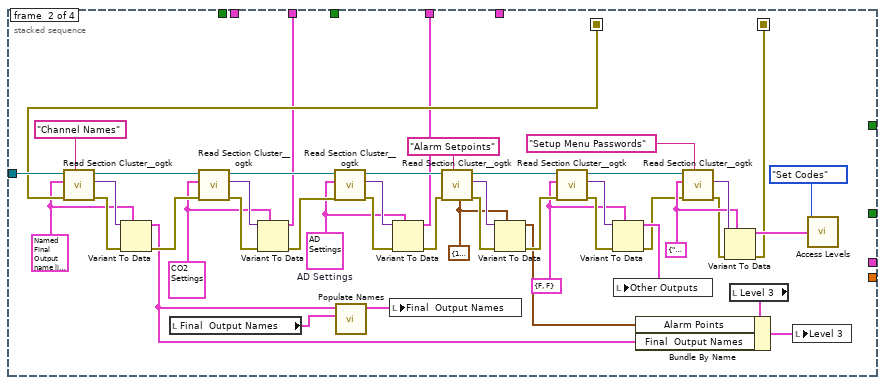
[diagram p8: hidden frame]
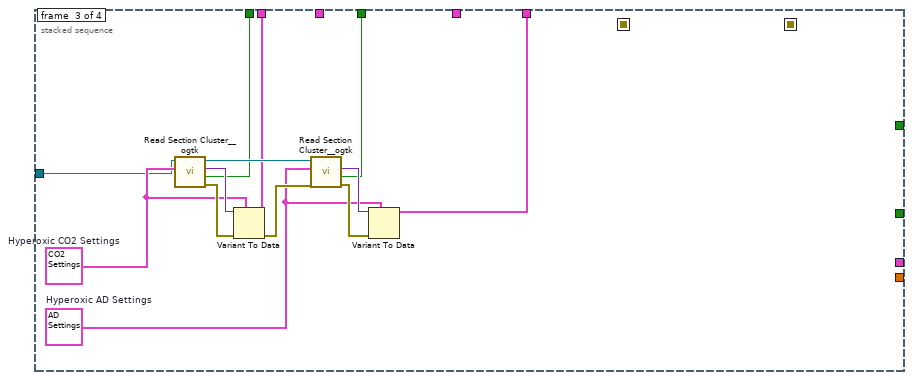
[diagram p9: hidden frame]
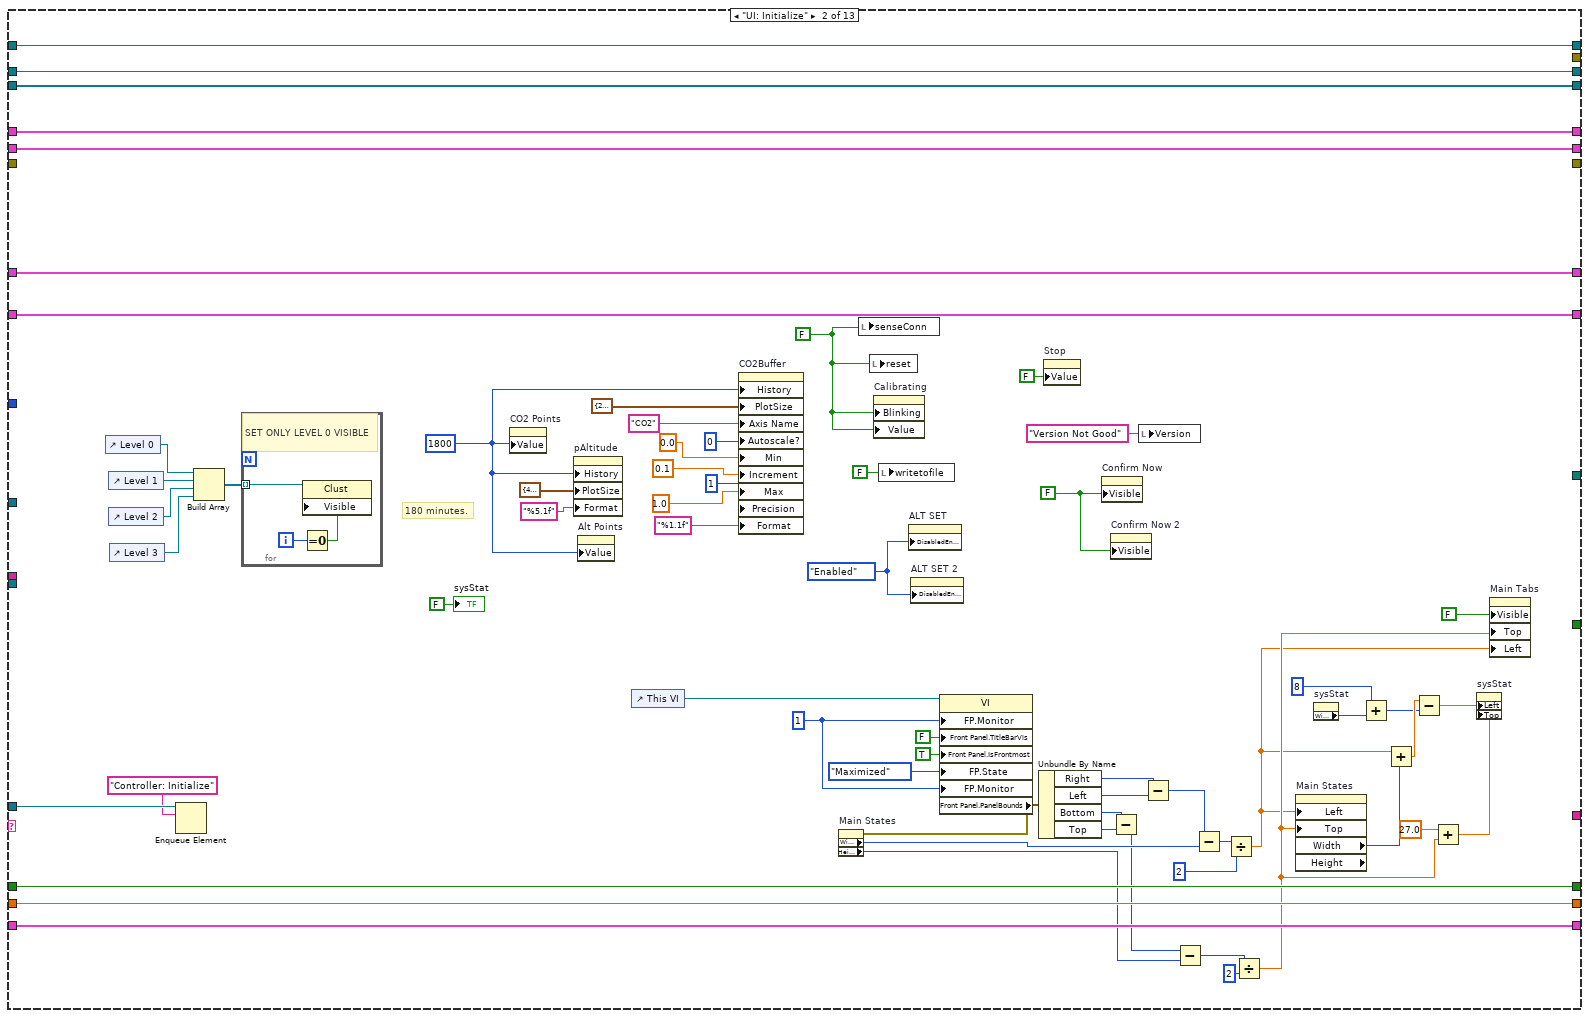
[diagram p10: hidden frame]
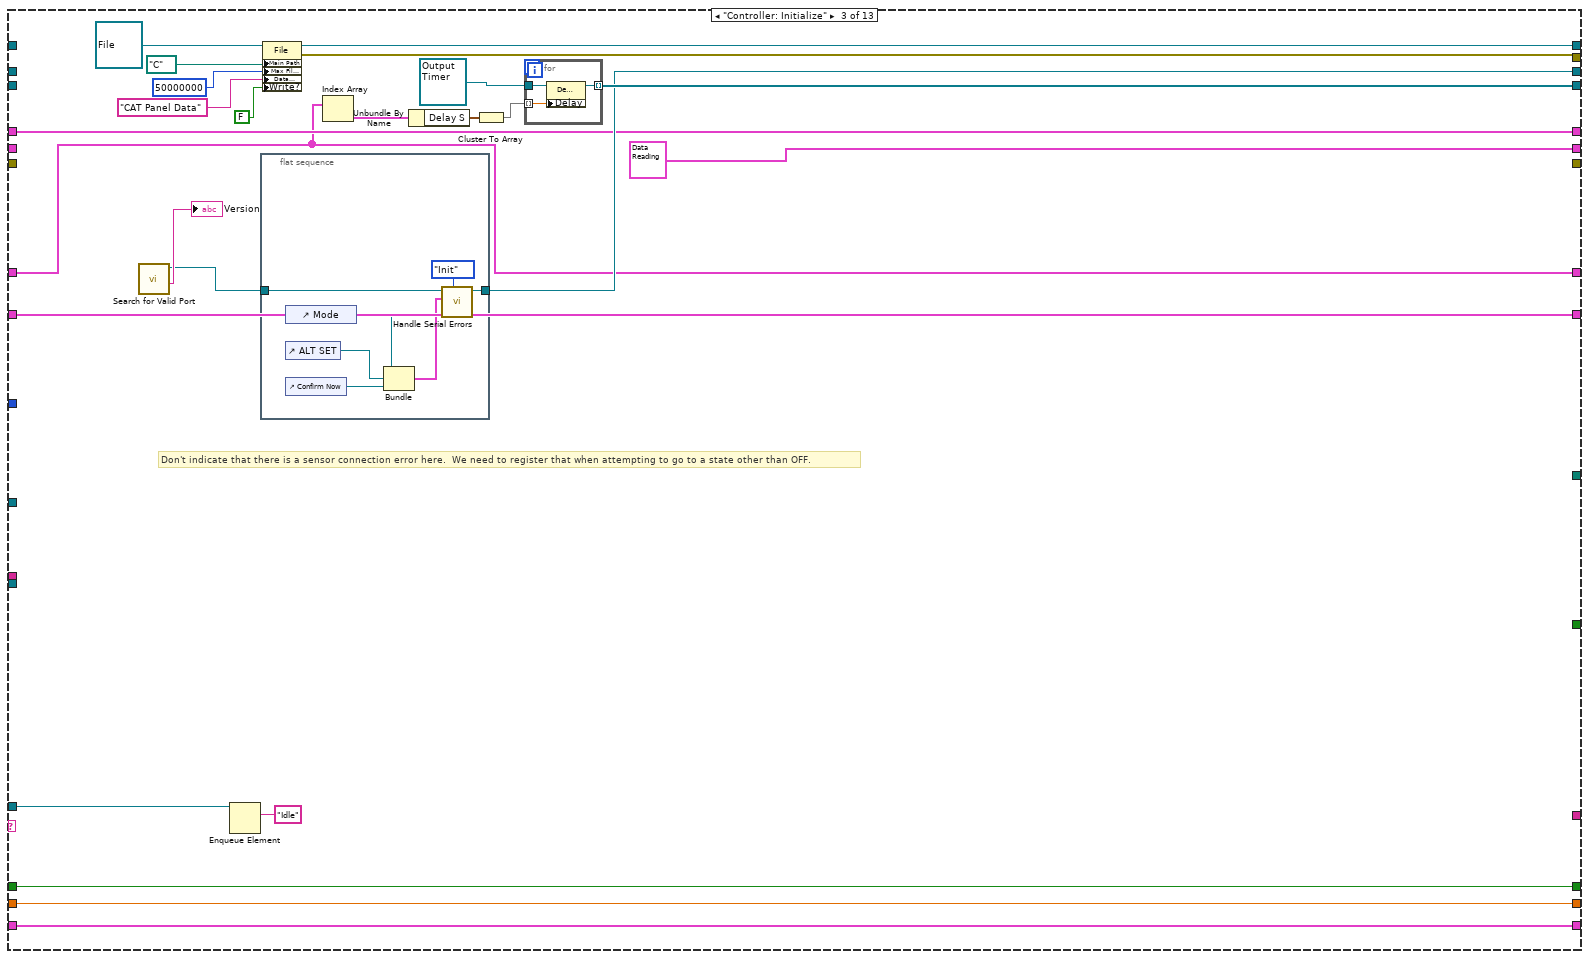
[diagram p11: hidden frame]
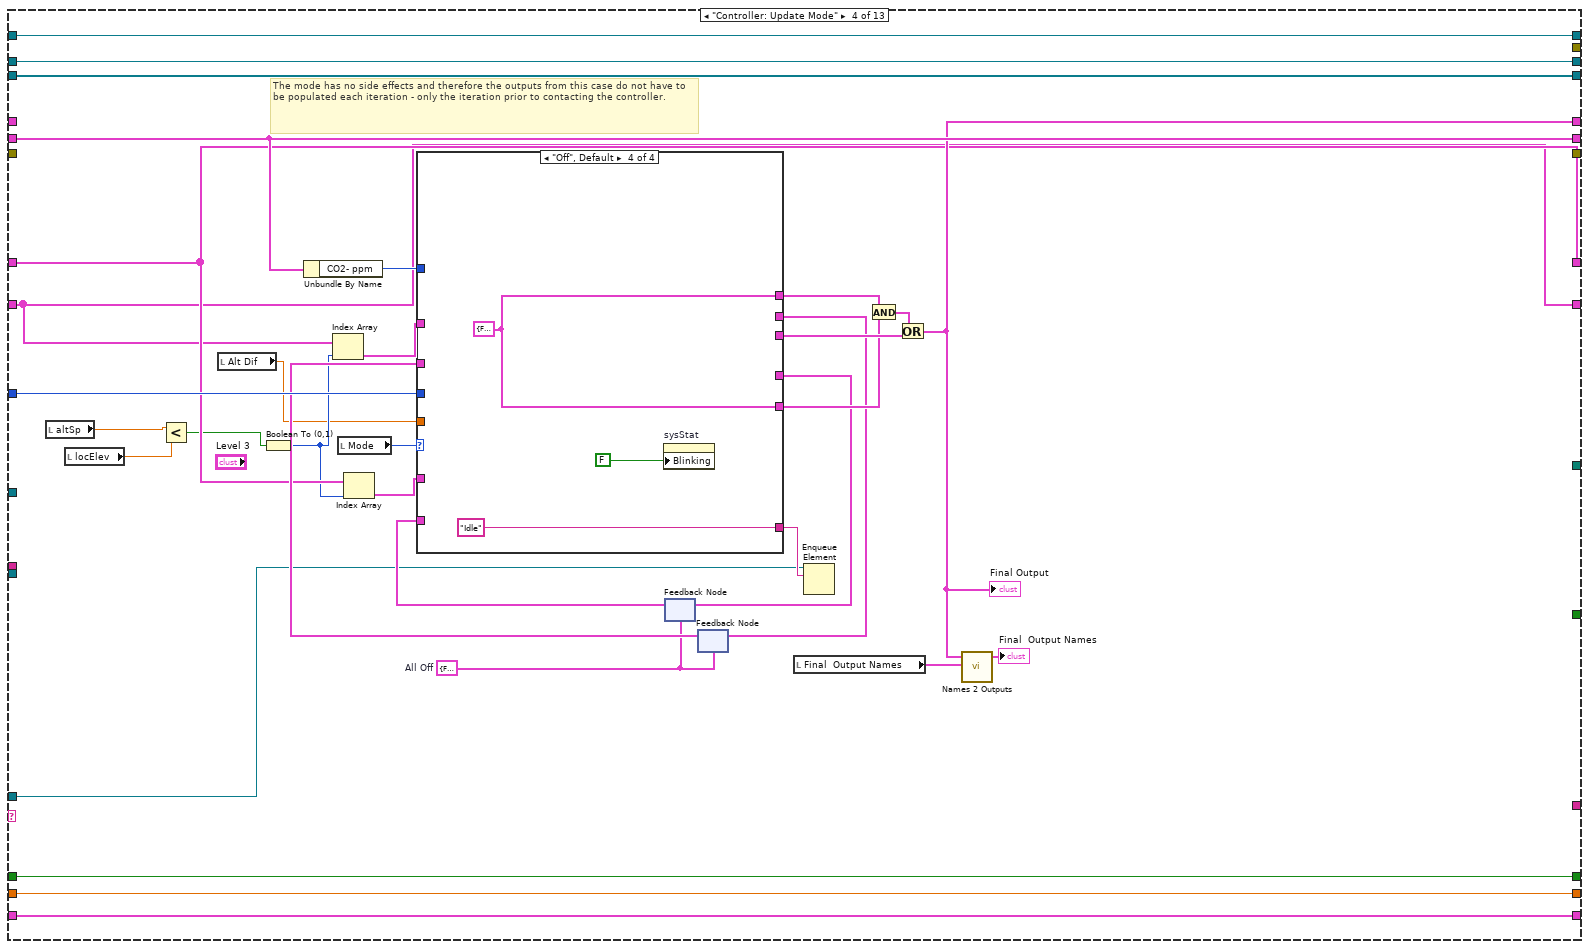
[diagram p12: hidden frame]
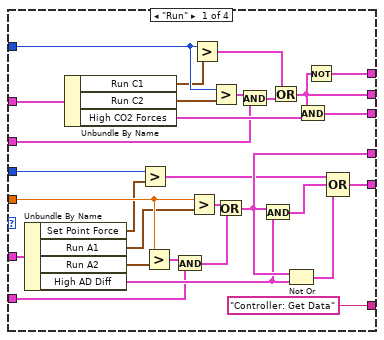
[diagram p13: hidden frame]
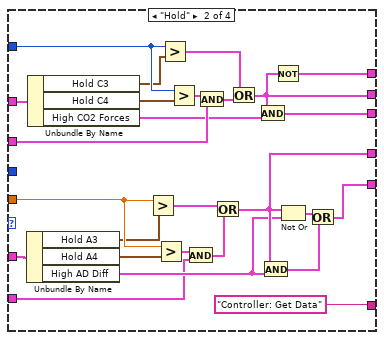
[diagram p14: hidden frame]
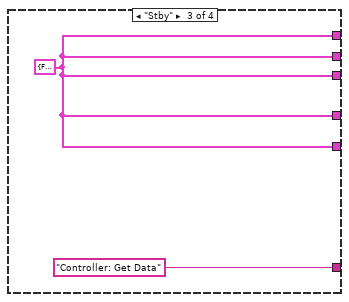
[diagram p15: hidden frame]
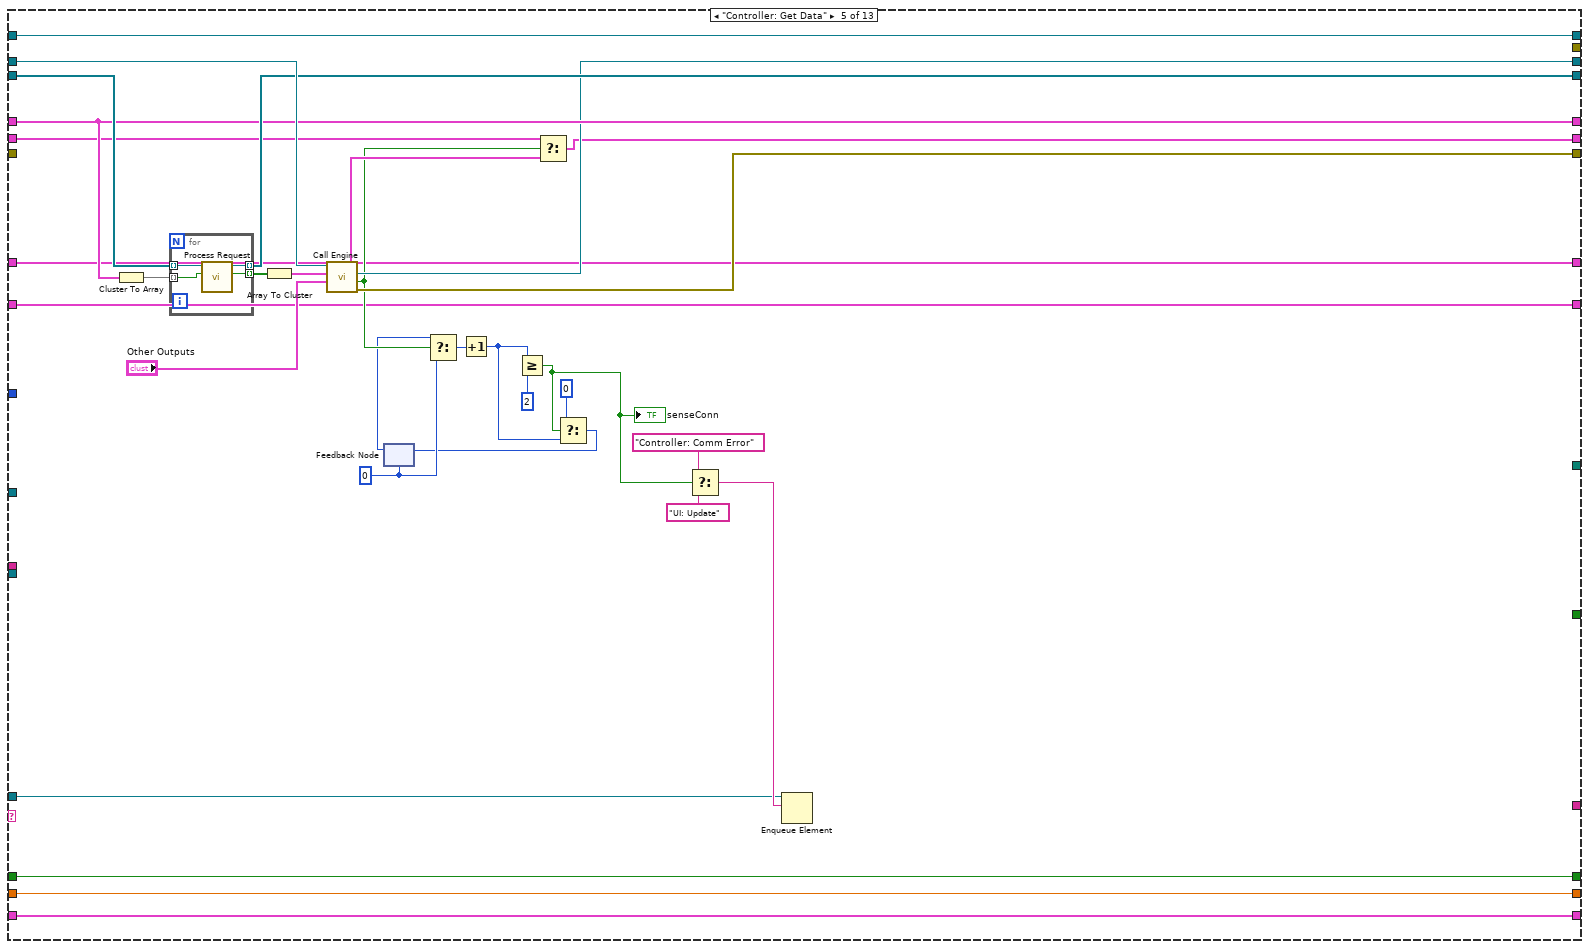
[diagram p16: hidden frame]
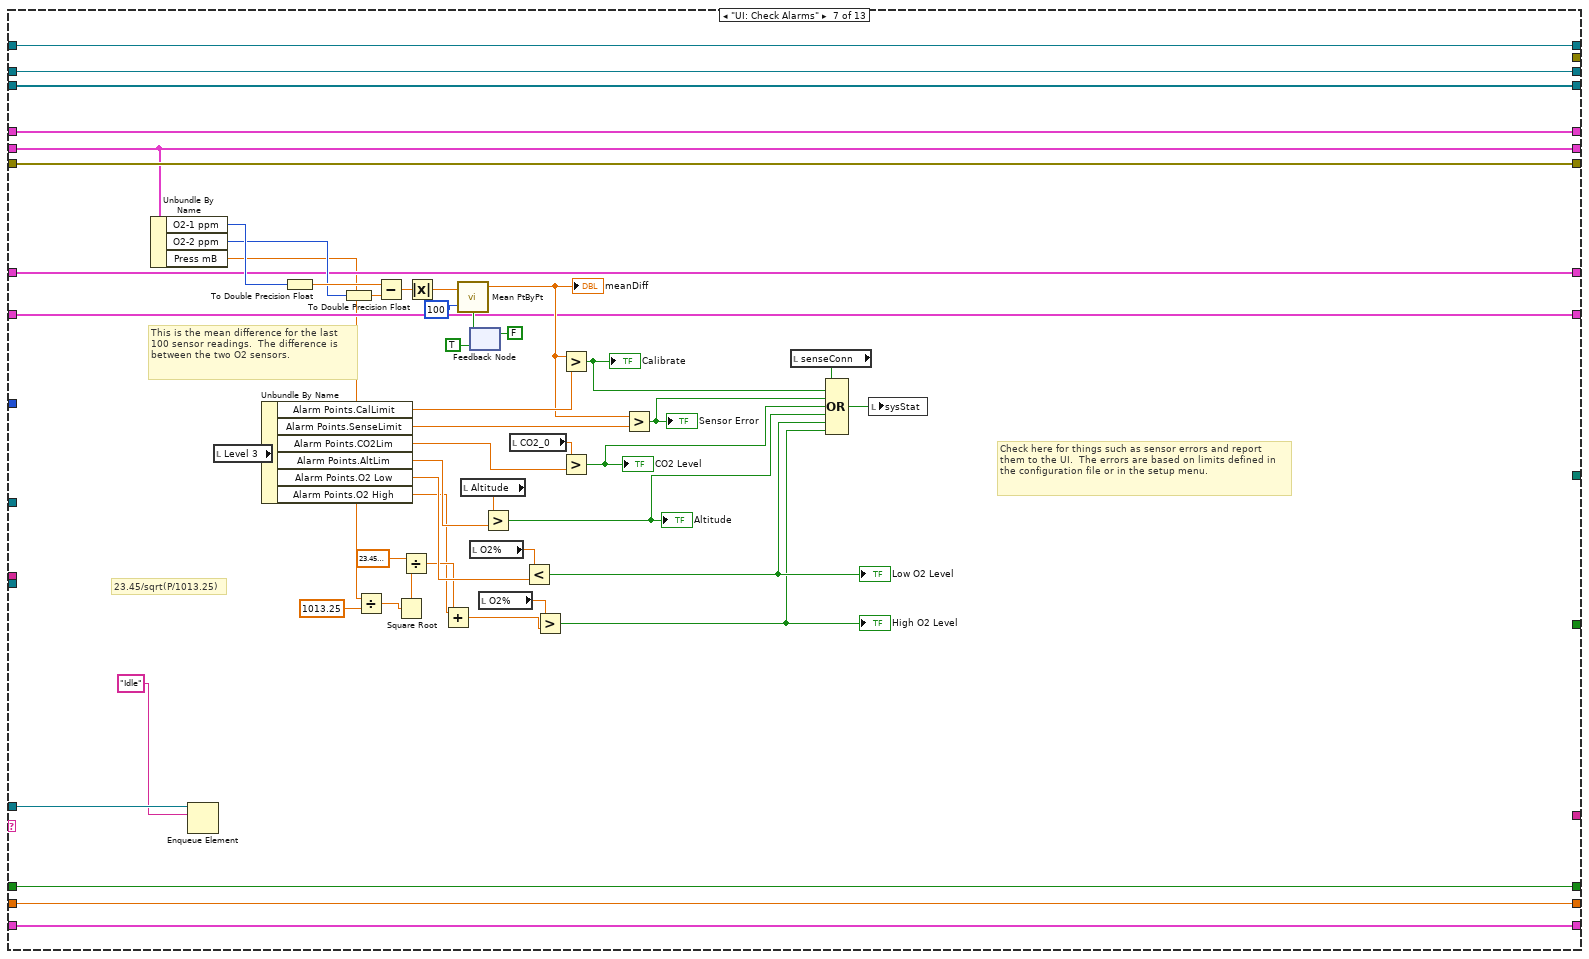
[diagram p18: hidden frame]
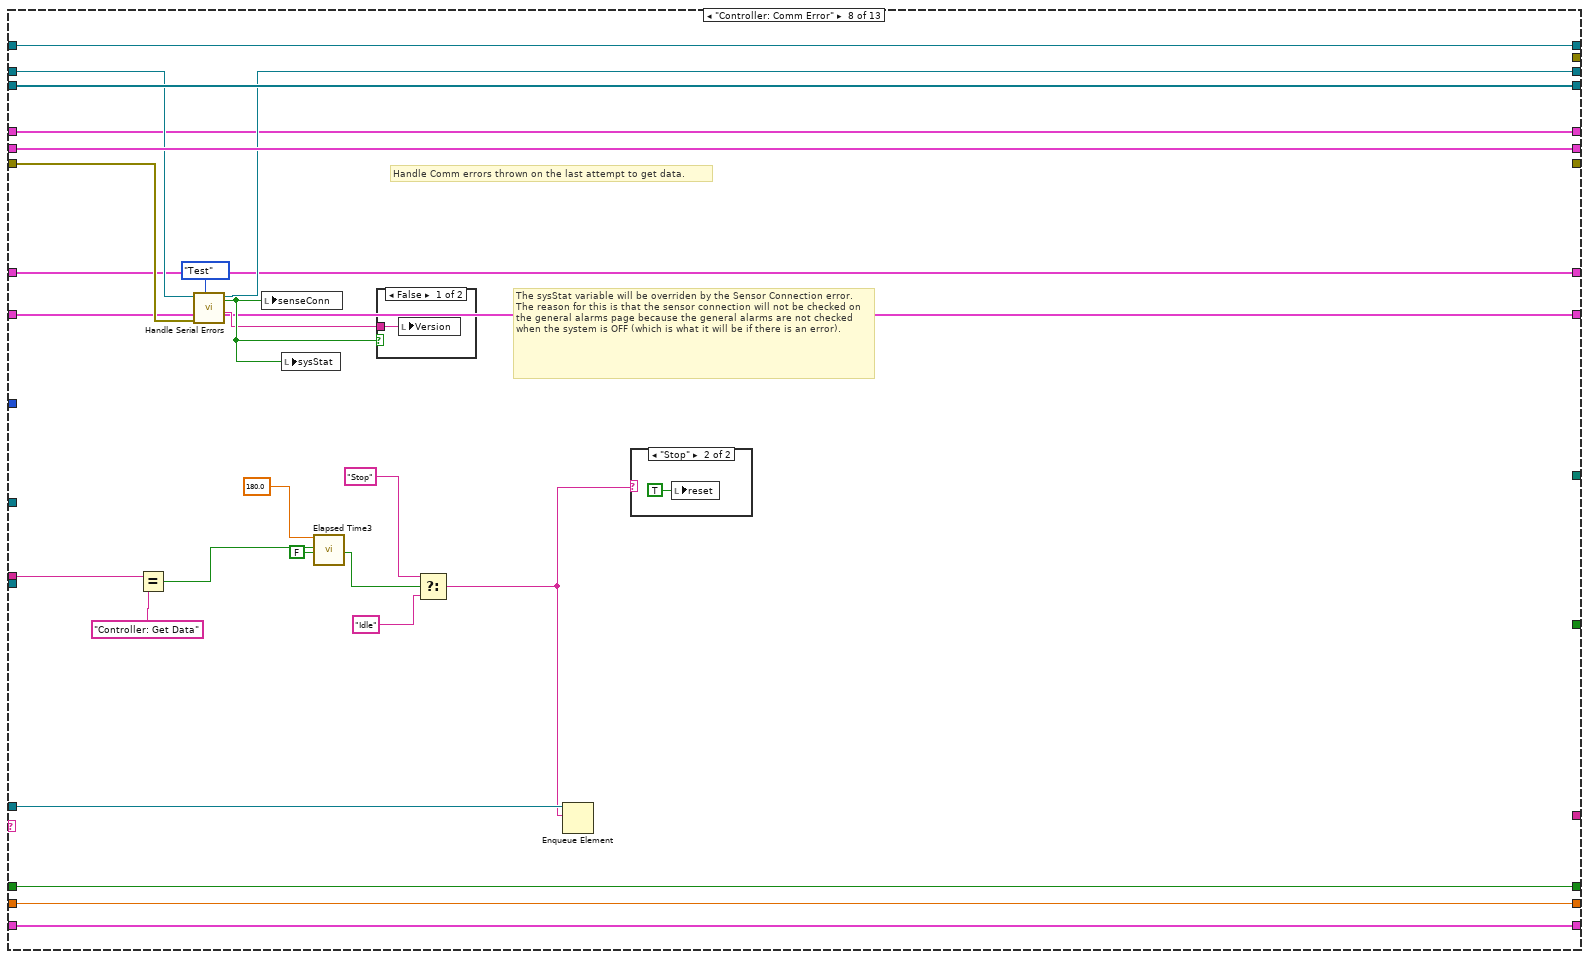
[diagram p19: hidden frame]
diagram:
  (unwired) i64 100 ("Period")
  # "Destroy the temp file only when we have exited."
  # "Since the silence alarms button is not latching, we watch for changes in state in this loop.\n\nIf the silence alarm button is pressed, set the byte to FALSE thus preventing the alarm from sounding.\n\nIF the sensor connection state changes, reset that byte to TRUE, thus allowing the the alarm to sound if there is another change in sensor connection state."
  n1 = Current VI's Path() -> (path=w6:path)
  n2 = Strip Path(path=w6) -> (stripped path=w5:path)  [unwired: 1 out]
  n3 = disable-structure shown="RUN_TIME_ENGINE==True" {
    disable-tunnel: w5 -> [w33 w35]
    disable-tunnel: [w31 w37] -> w4
    frame condition #0 (active) {
      n4 = Build Path(base path=w33, name or relative path="LV Screens\\Alt Disp.vi") -> (appended path=w31:path)
    }
    frame condition #1 {
      n5 = Strip Path(path=w35) -> (stripped path=w34:path)  [unwired: 1 out]
      n6 = Build Path(base path=w34, name or relative path="data\\Alt Disp.vi") -> (appended path=w37:path)
    }
  }
  n7 = property on="Pane" class="Pane"("Origin"=T20 {"Horizontal"=0, "Vertical"=0}) -> (error out=w1:errorcluster)  [unwired: 2 in, 1 out]
  n8 = Obtain Notifier(name (unnamed)="AltWinNot", notification data type=T21 {"Heading"="Current Effective Altitude in  Feet", "Altitude"=0.0, "Visible?"=TRUE}) -> (notifier out=w8:refnum<notifier>)  [unwired: 2 in, 2 out]
  n9 = Open VI Reference(type specifier VI Refnum (for type only)=refnum<vi> refnum, vi path=w4, options=128, error in (no error)=w1) -> (vi reference=w13:refnum<vi>, error out=w12:errorcluster)  [unwired: 2 in]
  n10 = call-by-ref "Start Asynchronous Call"(reference=w13, error in=w12, "Notifer In"=w8) -> (reference out=w7:refnum<vi>)  [unwired: 3 in, 1 out]
  n11 = Obtain Queue(element data type="UI: Initialize") -> (queue out=w19:refnum<queue>, error out=w18:errorcluster)  [unwired: 4 in, 1 out]
  n12 = Enqueue Element(queue=w19, element="Read Config File" ("f"), error in (no error)=w18) -> (queue out=w23:refnum<queue>, error out=w22:errorcluster)  [unwired: 1 in, 1 out]
  n13 = node-c288(i64 1000 ("Period")) -> (w29:T22)  [unwired: 1 in]
  n14 = while {
    shift-right: [w67] -> _
    shift-left: _ -> [w66]
    shift-right: [w68] -> _
    shift-left: _ -> [w69]
    shift-right: [w64] -> _
    shift-left: _ -> [w70]
    shift-right: [w61] -> _
    shift-left: _ -> [w60]
    shift-right: [w63] -> w26
    shift-left: _ -> [w59]
    tunnel: w23 -> [w58]
    tunnel: w22 -> [w57]
    shift-right: [w53] -> _
    shift-left: FALSE -> [w54]
    shift-right: [w52] -> _
    shift-left: _ -> [w51]
    shift-right: [w50] -> _
    shift-left: _ -> [w49]
    shift-right: [w48] -> _
    shift-left: _ -> [w47]
    shift-right: [w44] -> _
    shift-left: _ -> [w43]
    shift-right: [w42] -> _
    shift-left: _ -> [w41]
    tunnel: w8 -> [w40]
    tunnel: w7 -> [w39]
    tunnel: [w38] -> w3
    stop <- w65 stop-if-true
    n15 = Dequeue Element(queue=w58, timeout in ms (-1)=0, error in (no error)=w57) -> (queue out=w55:refnum<queue>, element=w46:string)  [unwired: 2 out]
    n16 = feedback-in #1(w46) -> ()
    n17 = feedback #1() -> (w45:string)  [unwired: 1 in]
    n18 = case shown="\"UI: Update\"" w46 {
      tunnel: w70 -> [w85 w298 _ w367 w465 w516 w572 w599 w615 w663 w1163 w1239 w1342]
      tunnel: w69 -> [w86 w297 _ w371 w464 w517 w573 w601 w617 w662 w1162 w1244 w1341]
      tunnel: [w86 w297 w328 w371 w463 w517 w573 w601 w617 w662 w1162 w1244 w1341] -> w68
      tunnel: [w87 w296 T26 {"Date"="", "Time"="", "CO2- ppm"=380, "Last Ctrl Word"=0, "O2-1 ppm"=209400, "O2-2 ppm"=209400, "Temp MB"=20.0, "Temp Sensor Module"=20.0, "Press mB"=1013.0} ("Data Read") w372 w455 w518 w570 w600 w616 w661 w1161 w1243 w1340] -> w67
      tunnel: w66 -> [w87 w296 _ w372 w456 w518 w570 w600 w616 w661 w1161 w1243 w1340]
      tunnel: [_ _ _ _ _ _ _ _ _ _ _ FALSE w1250] -> w65
      tunnel: [w85 w298 w325 w367 w458 w516 w572 w598 w614 w663 w1163 w1239 w1342] -> w64
      tunnel: [_ _ _ _ w452 _ w571 _ w609 _ _ w1238 w1339] -> w63
      tunnel: "Set Point Alt" -> [_ _ _ w373 _ w520 _ _ _ _ _ _ _]
      tunnel: [w91 w293 w322 w370 w462 w519 w576 w593 w612 w653 w1155 w1236 w1345] -> w61
      tunnel: w60 -> [w91 w293 w322 _ w462 w519 w576 w593 w612 w653 w1155 w1236 w1345]
      tunnel: w59 -> [_ _ _ _ _ _ w571 w597 _ _ _ _ w1339]
      tunnel: w55 -> [w84 w287 w313 w350 w450 w515 w550 w595 _ w655 w1157 w1232 w1298]
      tunnel: w54 -> [w90 w294 w323 w369 w449 w513 w575 w594 w613 w652 w1156 w1237 w1344]
      tunnel: [w90 w294 w323 w369 w449 w513 w575 w594 w611 w651 w1156 w1237 w1344] -> w53
      tunnel: [w89 w289 w318 w368 w448 w511 w574 w592 w608 w649 w1153 w1234 w1343] -> w52
      tunnel: w51 -> [w89 w289 _ w368 w448 w512 w574 w592 w608 w650 w1153 w1235 w1343]
      tunnel: [_ _ w315 _ _ _ _ _ _ _ _ _ _] -> _
      tunnel: [w81 w273 w311 w353 w437 w495 w538 w589 w607 w646 w1150 w1230 w1289] -> w50
      tunnel: w49 -> [_ w273 w311 w353 w437 w495 w538 w589 w607 w647 w1150 w1230 w1289]
      tunnel: [w80 w272 w310 w352 w436 w493 w537 w588 w606 w644 w1145 w1229 w1284] -> w48
      tunnel: w47 -> [_ w272 w310 w352 w436 w493 w537 w588 w606 w645 w1146 w1229 w1284]
      tunnel: w45 -> [_ _ _ _ _ _ _ w587 _ _ _ _ _]
      tunnel: [w76 w271 w309 w349 w435 w485 w536 w578 w605 w642 w1141 w1228 w1281] -> w44
      tunnel: w43 -> [_ w271 w309 w349 w435 w485 w536 w578 w605 w643 w1141 w1228 w1281]
      tunnel: [w75 w270 w307 w346 w434 w484 w535 w577 w604 w639 w1140 w1227 w1270] -> w42
      tunnel: w41 -> [_ w270 w307 w346 w434 w484 w535 w577 w604 w640 w1140 w1227 w1270]
      tunnel: w40 -> [_ _ _ _ _ _ _ _ _ w641 _ w1226 w1249]
      tunnel: w39 -> [_ _ _ _ _ _ _ _ _ _ _ w1224 _]
      tunnel: [_ _ _ _ _ _ _ _ _ _ w1137 _ _] -> _
      tunnel: [_ _ _ _ _ _ _ _ _ _ _ _ w1247] -> w38
      frame "Read Config File" {
        n19 = call "Open Config Path.vi"() -> ("error out"=w83:errorcluster, "cfg_ref out"=w88:T27)  [unwired: 10 in]
        n20 = case shown="Error" w83 {
          tunnel: w88 -> [w102 _]
          tunnel: [w103 TRUE ("Canceled?")] -> w82
          tunnel: [w101 _] -> w81
          tunnel: [w100 _] -> w80
          tunnel: [w99 _] -> w72
          tunnel: [w98 _] -> w71
          tunnel: [w97 _] -> w74
          tunnel: [w96 _] -> w73
          frame No Error {
            n21 = stacked-sequence {
              seq-local: [w110 _ _ _] -> [_ w172 _ _]
              seq-local: [_ w151 _ _] -> [_ _ _ w223]
              tunnel: w102 -> [w142 w180 w196 w233]
              tunnel: [_ _ _ w236] -> w103
              tunnel: [_ _ _ w230] -> w101
              tunnel: [_ _ _ w229] -> w100
              tunnel: [_ w148 _ _] -> w99
              tunnel: [_ _ w194 _] -> _
              tunnel: [_ _ w195 _] -> _
              tunnel: [_ _ w193 _] -> w98
              tunnel: [_ _ w192 _] -> w96
              tunnel: [_ w147 _ _] -> w97
              tunnel: [_ _ _ w207] -> _
              frame #0 {
                w129 = T28."Enabled" ("Disabled")
                w109 = "Altitude" ("section")
                n22 = call-poly <vilib>:"Read Key.vi"("section"="Mode", "key"="mode?", "refnum"=w142) -> ("error out"=w133:errorcluster, "value"=w128:i32, "refnum out"=w141:T27)  [unwired: 5 in, 1 out]
                n23 = call-poly <vilib>:"Read Key.vi"("section"=w109, "error in (no error)"=w133, "key"="Setpoint", "refnum"=w141) -> ("error out"=w132:errorcluster, "value"=w125:dbl, "refnum out"=w140:T27)  [unwired: 4 in, 1 out]
                n24 = property on="Mode 1" class="VertMode (strict)"("DisabledEnum"=w129) -> ()  [unwired: 2 in, 2 out]
                n25 = property on="Mode" class="VertMode (strict)"("Val(Sgnl)"=w128, "DisabledEnum"=w129) -> ()  [unwired: 2 in, 2 out]
                n26 = call-poly <vilib>:"Read Key.vi"("section"=w109, "error in (no error)"=w132, "key"="West?", "refnum"=w140) -> ("error out"=w113:errorcluster, "value"=w130:bool, "refnum out"=w121:T27)  [unwired: 4 in, 1 out]
                n27 = call "Convert Dbl to ALtitude.vi"("Setpoint"=w125) -> ("Altitude Out"=w126:T29)  [unwired: 10 in]
                n28 = To Long Integer(number=w125) -> (32bit integer=w127:i32)
                n29 = local write "Set Point Alt"(w127) -> ()
                n30 = call-poly <vilib>:"Read Key.vi"("section"=w109, "error in (no error)"=w113, "key"="Max", "refnum"=w121) -> ("error out"=w119:errorcluster, "value"=w131:dbl, "refnum out"=w120:T27)  [unwired: 4 in, 1 out]
                n31 = property on="West ON/Std OFF" class="Bool (strict)"("Value"=w130) -> ()  [unwired: 2 in, 2 out]
                n32 = local write "ALT SET 2"(w126) -> ()
                n33 = local write "ALT SET"(w126) -> ()
                n34 = property on="maxAltSP" class="DigNum (strict)"("Value"=w131) -> ()  [unwired: 2 in, 2 out]
                n35 = call-poly <vilib>:"Read Key.vi"("section"=w109, "error in (no error)"=w119, "key"="Meters?", "refnum"=w120) -> ("error out"=w117:errorcluster, "value"=w124:bool, "refnum out"=w118:T27)  [unwired: 4 in, 1 out]
                n36 = property on="Feet OFF/ Meters ON" class="Bool (strict)"("Value"=w124) -> ()  [unwired: 2 in, 2 out]
                n37 = call-poly <vilib>:"Read Key.vi"("section"=w109, "error in (no error)"=w117, "key"="custMax", "refnum"=w118) -> ("error out"=w114:errorcluster, "value"=w115:dbl, "refnum out"=w112:T27)  [unwired: 4 in, 1 out]
                n38 = property on="Max Altitude" class="DigNum (strict)"(error in=w114, "Value"=w115) -> (error out=w111:errorcluster)  [unwired: 1 in, 1 out]
                n39 = property on="Confirm Now" class="Bool (strict)"("Val(Sgnl)"=TRUE ("Value (Signaling)")) -> ()  [unwired: 2 in, 2 out]
                n40 = call-poly <vilib>:"Read Key.vi"("section"=w109, "error in (no error)"=w111, "key"="Buffer", "refnum"=w112) -> ("error out"=w110:errorcluster, "value"=w107:dbl)  [unwired: 4 in, 2 out]
                n41 = case shown="False" w124 {
                  tunnel: ["Current Effective Altitude in Feet" ("Heading") "Current Effective Altitude in Meters" ("Heading")] -> w123
                  tunnel: ["F\ne\ne\nt" ("Units") "M\ne\nt\ne\nr\ns" ("Units")] -> w122
                  frame False {
                  }
                  frame True {
                  }
                }
                n42 = Divide(x=w107, y=100.0) -> (x/y=w105:dbl)
                n43 = property on="Buffer" class="DigNum (strict)"("Value"=w105) -> ()  [unwired: 2 in, 2 out]
                n44 = local write "Heading 2"(w123) -> ()
                n45 = local write "Units"(w122) -> ()
              }
              frame #1 {
                w155 = T30 {"Level 1 Password"="123", "Level 2 Password"="228", "Level 3 Password"="3228679"} ("Setup Menu Passwords")
                w168 = cluster{"Alarm":bool, "Heater":bool} {"Alarm"=FALSE, "Heater"=FALSE} ("Other Outputs")
                w169 = T31 {"CalLimit"=10000.0, "SenseLimit"=10000.0, "CO2Lim"=10000.0, "AltLim"=10000.0, "O2 Low"=10000.0, "O2 High"=10000.0} ("Alarm Setpoints")
                w170 = T6 {"Set Point Force"={"A-1,  1"=inf, "A-3,  2"=inf, "A-4, 3"=inf, "A-5, 4"=5790.0, "ABCD-7, 5"=inf, "A-8, 6"=inf, "B-1,  7"=5790.0, "B-3, 8"=5790.0, "B-4,  9"=inf, "B-5, 10"=5790.0, "B-8, 11"=inf, "C-1, 12"=inf, "C-3, 13"=inf, "C-4, 14"=inf, "C-5,  15"=5790.0, "C-8, 16"=inf, "D-1, 17"=inf, "D-3, 18"=inf, "D-4,  19"=inf, "D-5,  20"=inf, "D-8,  21"=inf}, "Run A1"={"A-1,  1"=inf, "A-3,  2"=inf, "A-4, 3"=3.0, "A-5, 4"=inf, "ABCD-7, 5"=67.0, "A-8, 6"=630.0, "B-1,  7"=-30.0, "B-3, 8"=-30.0, "B-4,  9"=3.0, "B-5, 10"=inf, "B-8, 11"=630.0, "C-1, 12"=-60.0, "C-3, 13"=-60.0, "C-4, 14"=3.0, "C-5,  15"=inf, "C-8, 16"=630.0, "D-1, 17"=inf, "D-3, 18"=-30.0, "D-4,  19"=-60.0, "D-5,  20"=630.0, "D-8,  21"=930.0}, "Run A2"={"A-1,  1"=inf, "A-3,  2"=inf, "A-4, 3"=-3.0, "A-5, 4"=inf, "ABCD-7, 5"=60.0, "A-8, 6"=610.0, "B-1,  7"=-100.0, "B-3, 8"=-100.0, "B-4,  9"=-3.0, "B-5, 10"=inf, "B-8, 11"=610.0, "C-1, 12"=-120.0, "C-3, 13"=-120.0, "C-4, 14"=-3.0, "C-5,  15"=inf, "C-8, 16"=610.0, "D-1, 17"=inf, "D-3, 18"=-100.0, "D-4,  19"=-120.0, "D-5,  20"=610.0, "D-8,  21"=910.0}, "Hold A3"={"A-1,  1"=0.0, "A-3,  2"=0.0, "A-4, 3"=3.0, "A-5, 4"=inf, "ABCD-7, 5"=67.0, "A-8, 6"=630.0, "B-1,  7"=-150.0, "B-3, 8"=-150.0, "B-4,  9"=3.0, "B-5, 10"=inf, "B-8, 11"=630.0, "C-1, 12"=-300.0, "C-3, 13"=-300.0, "C-4, 14"=3.0, "C-5,  15"=inf, "C-8, 16"=630.0, "D-1, 17"=0.0, "D-3, 18"=-150.0, "D-4,  19"=-300.0, "D-5,  20"=630.0, "D-8,  21"=930.0}, "Hold A4"={"A-1,  1"=-150.0, "A-3,  2"=-150.0, "A-4, 3"=-3.0, "A-5, 4"=inf, "ABCD-7, 5"=60.0, "A-8, 6"=610.0, "B-1,  7"=-250.0, "B-3, 8"=-250.0, "B-4,  9"=-3.0, "B-5, 10"=inf, "B-8, 11"=610.0, "C-1, 12"=-500.0, "C-3, 13"=-500.0, "C-4, 14"=-3.0, "C-5,  15"=inf, "C-8, 16"=610.0, "D-1, 17"=-150.0, "D-3, 18"=-250.0, "D-4,  19"=-500.0, "D-5,  20"=610.0, "D-8,  21"=910.0}, "High AD Diff "={"A-1, 1"=FALSE, "A-3, 2"=FALSE, "A-4, 3"=FALSE, "A-5, 4"=TRUE, "ABCD-7, 5"=FALSE, "A-8, 6"=TRUE, "B-1,  7"=FALSE, "B-3, 8"=FALSE, "B-4, 9"=FALSE, "B-5, 10"=TRUE, "B-8,  11"=TRUE, "C-1, 12"=FALSE, "C-3, 13"=FALSE, "C-4,  14"=FALSE, "C-5,  15"=TRUE, "C-8, 16"=TRUE, "D-1, 17"=FALSE, "D-3, 18"=FALSE, "D-4, 19"=FALSE, "D-5,  20"=TRUE, "D-8,  21"=TRUE}, "Delay S"={"A-1,  1"=30.0, "A-3,  2"=30.0, "A-4, 3"=1.0, "A-5, 4"=1.0, "ABCD-7, 5"=1.0, "A-8, 6"=1.0, "B-1,  7"=30.0, "B-3, 8"=30.0, "B-4,  9"=1.0, "B-5, 10"=1.0, "B-8, 11"=1.0, "C-1, 12"=30.0, "C-3, 13"=30.0, "C-4, 14"=1.0, "C-5,  15"=1.0, "C-8, 16"=1.0, "D-1, 17"=30.0, "D-3, 18"=30.0, "D-4,  19"=30.0, "D-5,  20"=1.0, "D-8,  21"=1.0}}  # AD Settings
                w164 = T3 {"Run C1"={"A-1,  1"=inf, "A-3,  2"=inf, "A-4, 3"=9600.0, "A-5, 4"=8800.0, "ABCD-7, 5"=9800.0, "A-8, 6"=9800.0, "B-1,  7"=3400.0, "B-3, 8"=3400.0, "B-4,  9"=9600.0, "B-5, 10"=8800.0, "B-8, 11"=9800.0, "C-1, 12"=1800.0, "C-3, 13"=1800.0, "C-4, 14"=9600.0, "C-5,  15"=8800.0, "C-8, 16"=9800.0, "D-1, 17"=inf, "D-3, 18"=3400.0, "D-4,  19"=1800.0, "D-5,  20"=9800.0, "D-8,  21"=9800.0}, "Run C2"={"A-1,  1"=inf, "A-3,  2"=inf, "A-4, 3"=9500.0, "A-5, 4"=8600.0, "ABCD-7, 5"=9700.0, "A-8, 6"=9700.0, "B-1,  7"=3000.0, "B-3, 8"=3000.0, "B-4,  9"=9500.0, "B-5, 10"=8600.0, "B-8, 11"=9700.0, "C-1, 12"=1400.0, "C-3, 13"=1400.0, "C-4, 14"=9500.0, "C-5,  15"=8600.0, "C-8, 16"=9700.0, "D-1, 17"=inf, "D-3, 18"=3000.0, "D-4,  19"=1400.0, "D-5,  20"=9700.0, "D-8,  21"=9700.0}, "Hold C3"={"A-1,  1"=1800.0, "A-3,  2"=1800.0, "A-4, 3"=9000.0, "A-5, 4"=8800.0, "ABCD-7, 5"=9800.0, "A-8, 6"=9800.0, "B-1,  7"=3400.0, "B-3, 8"=3400.0, "B-4,  9"=9000.0, "B-5, 10"=8800.0, "B-8, 11"=9800.0, "C-1, 12"=1800.0, "C-3, 13"=1800.0, "C-4, 14"=9000.0, "C-5,  15"=8800.0, "C-8, 16"=9800.0, "D-1, 17"=1800.0, "D-3, 18"=3400.0, "D-4,  19"=1800.0, "D-5,  20"=9800.0, "D-8,  21"=9800.0}, "Hold C4"={"A-1,  1"=1400.0, "A-3,  2"=1400.0, "A-4, 3"=8800.0, "A-5, 4"=8600.0, "ABCD-7, 5"=9700.0, "A-8, 6"=9700.0, "B-1,  7"=3000.0, "B-3, 8"=3000.0, "B-4,  9"=8800.0, "B-5, 10"=8600.0, "B-8, 11"=9700.0, "C-1, 12"=1400.0, "C-3, 13"=1400.0, "C-4, 14"=8800.0, "C-5,  15"=8600.0, "C-8, 16"=9700.0, "D-1, 17"=1400.0, "D-3, 18"=3000.0, "D-4,  19"=1400.0, "D-5,  20"=9700.0, "D-8,  21"=9700.0}, "High CO2 Forces"={"A-1, 1"=TRUE, "A-3, 2"=TRUE, "A-4, 3"=FALSE, "A-5, 4"=TRUE, "ABCD-7, 5"=FALSE, "A-8, 6"=TRUE, "B-1,  7"=TRUE, "B-3, 8"=TRUE, "B-4, 9"=FALSE, "B-5, 10"=TRUE, "B-8,  11"=TRUE, "C-1, 12"=TRUE, "C-3, 13"=TRUE, "C-4,  14"=FALSE, "C-5,  15"=TRUE, "C-8, 16"=TRUE, "D-1, 17"=TRUE, "D-3, 18"=TRUE, "D-4, 19"=TRUE, "D-5,  20"=TRUE, "D-8,  21"=TRUE}} ("CO2 Settings")
                w171 = T18 {"A-1, 1"="Main", "A-3, 2"="Main", "A-4, 3"="Recirculation", "A-5, 4"="Scrubber", "A-7, 5"="Oxygen", "A-8, 6"="Vent", "B-1,  7"="Boost A", "B-3, 8"="Boost A", "B-4, 9"="Recirculation", "B-5, 10"="Scrubber", "B-8, 11"="Vent", "C-1, 12"="Boost B", "C-3, 13"="Boost B", "C-4, 14"="Recirculation", "C-5,  15"="Scrubber", "C-8, 16"="Vent", "D-1, 17"="+24V", "D-3, 18"="Main", "D-4,  19"="Boost A", "D-5,  20"="Boost B", "D-8,  21"="Vent"} ("Channel Names")
                n46 = call <userlib>:"Read Section Cluster__ogtk.vi"("section (optional)"="Channel Names", "error in (no error)"=w172, "Section Formatted Cluster Type"=w171, "refnum"=w180) -> ("error out"=w186:errorcluster, "Section Formatted Cluster"=w185:variant, "dup refnum"=w181:T27)  [unwired: 3 in, 2 out]
                n47 = Variant To Data(error in=w186, type=w171, Variant=w185) -> (data=w163:T18, error out=w187:errorcluster)
                n48 = local read "Final  Output Names"() -> (w161:T11)
                n49 = call <userlib>:"Read Section Cluster__ogtk.vi"("error in (no error)"=w187, "Section Formatted Cluster Type"=w164, "refnum"=w181) -> ("error out"=w179:errorcluster, "Section Formatted Cluster"=w188:variant, "dup refnum"=w182:T27)  [unwired: 4 in, 2 out]
                n50 = Variant To Data(error in=w179, type=w164, Variant=w188) -> (data=w147:T3, error out=w178:errorcluster)
                n51 = call <userlib>:"Read Section Cluster__ogtk.vi"("error in (no error)"=w178, "Section Formatted Cluster Type"=w170, "refnum"=w182) -> ("error out"=w177:errorcluster, "Section Formatted Cluster"=w189:variant, "dup refnum"=w183:T27)  [unwired: 4 in, 2 out]
                n52 = call "Populate Names.vi"("Final  Output In"=w161, "Final Names"=w163) -> ("Final  Output Out"=w162:T11)  [unwired: 9 in]
                n53 = local write "Final  Output Names"(w162) -> ()
                n54 = Variant To Data(error in=w177, type=w170, Variant=w189) -> (data=w148:T6, error out=w176:errorcluster)
                n55 = call <userlib>:"Read Section Cluster__ogtk.vi"("section (optional)"="Alarm Setpoints", "error in (no error)"=w176, "Section Formatted Cluster Type"=w169, "refnum"=w183) -> ("error out"=w175:errorcluster, "Section Formatted Cluster"=w190:variant, "dup refnum"=w184:T27)  [unwired: 3 in, 2 out]
                n56 = Variant To Data(error in=w175, type=w169, Variant=w190) -> (data=w159:T31, error out=w174:errorcluster)
                n57 = call <userlib>:"Read Section Cluster__ogtk.vi"("error in (no error)"=w174, "Section Formatted Cluster Type"=w168, "refnum"=w184) -> ("error out"=w173:errorcluster, "Section Formatted Cluster"=w191:variant, "dup refnum"=w157:T27)  [unwired: 4 in, 2 out]
                n58 = Variant To Data(error in=w173, type=w168, Variant=w191) -> (data=w167:cluster{"Alarm":bool, "Heater":bool}, error out=w150:errorcluster)
                n59 = local write "Other Outputs"(w167) -> ()
                n60 = call <userlib>:"Read Section Cluster__ogtk.vi"("section (optional)"="Setup Menu Passwords", "error in (no error)"=w150, "Section Formatted Cluster Type"=w155, "refnum"=w157) -> ("error out"=w149:errorcluster, "Section Formatted Cluster"=w156:variant)  [unwired: 3 in, 3 out]
                n61 = Variant To Data(error in=w149, type=w155, Variant=w156) -> (data=w152:T30, error out=w151:errorcluster)
                n62 = local read "Level 3"() -> (w166:T19)
                n63 = Bundle By Name(cluster=w166, "Alarm Points"=w159, "Final  Output Names"=w163) -> (w165:T19)
                n64 = local write "Level 3"(w165) -> ()
                n65 = call "Access Levels.vi"("Setup Menu Passwords"=w152, "Action"=enum8{"Set Codes", "Get Level"}."Set Codes") -> ()  [unwired: 3 in, 1 out]
              }
              frame #2 {
                w198 = T6 {"Set Point Force"={"A-1,  1"=inf, "A-3,  2"=inf, "A-4, 3"=inf, "A-5, 4"=5790.0, "ABCD-7, 5"=inf, "A-8, 6"=inf, "B-1,  7"=5790.0, "B-3, 8"=5790.0, "B-4,  9"=inf, "B-5, 10"=5790.0, "B-8, 11"=inf, "C-1, 12"=inf, "C-3, 13"=inf, "C-4, 14"=inf, "C-5,  15"=5790.0, "C-8, 16"=inf, "D-1, 17"=inf, "D-3, 18"=inf, "D-4,  19"=inf, "D-5,  20"=inf, "D-8,  21"=inf}, "Run A1"={"A-1,  1"=inf, "A-3,  2"=inf, "A-4, 3"=3.0, "A-5, 4"=inf, "ABCD-7, 5"=67.0, "A-8, 6"=630.0, "B-1,  7"=-30.0, "B-3, 8"=-30.0, "B-4,  9"=3.0, "B-5, 10"=inf, "B-8, 11"=630.0, "C-1, 12"=-60.0, "C-3, 13"=-60.0, "C-4, 14"=3.0, "C-5,  15"=inf, "C-8, 16"=630.0, "D-1, 17"=inf, "D-3, 18"=-30.0, "D-4,  19"=-60.0, "D-5,  20"=630.0, "D-8,  21"=930.0}, "Run A2"={"A-1,  1"=inf, "A-3,  2"=inf, "A-4, 3"=-3.0, "A-5, 4"=inf, "ABCD-7, 5"=60.0, "A-8, 6"=610.0, "B-1,  7"=-100.0, "B-3, 8"=-100.0, "B-4,  9"=-3.0, "B-5, 10"=inf, "B-8, 11"=610.0, "C-1, 12"=-120.0, "C-3, 13"=-120.0, "C-4, 14"=-3.0, "C-5,  15"=inf, "C-8, 16"=610.0, "D-1, 17"=inf, "D-3, 18"=-100.0, "D-4,  19"=-120.0, "D-5,  20"=610.0, "D-8,  21"=910.0}, "Hold A3"={"A-1,  1"=0.0, "A-3,  2"=0.0, "A-4, 3"=3.0, "A-5, 4"=inf, "ABCD-7, 5"=67.0, "A-8, 6"=630.0, "B-1,  7"=-150.0, "B-3, 8"=-150.0, "B-4,  9"=3.0, "B-5, 10"=inf, "B-8, 11"=630.0, "C-1, 12"=-300.0, "C-3, 13"=-300.0, "C-4, 14"=3.0, "C-5,  15"=inf, "C-8, 16"=630.0, "D-1, 17"=0.0, "D-3, 18"=-150.0, "D-4,  19"=-300.0, "D-5,  20"=630.0, "D-8,  21"=930.0}, "Hold A4"={"A-1,  1"=-150.0, "A-3,  2"=-150.0, "A-4, 3"=-3.0, "A-5, 4"=inf, "ABCD-7, 5"=60.0, "A-8, 6"=610.0, "B-1,  7"=-250.0, "B-3, 8"=-250.0, "B-4,  9"=-3.0, "B-5, 10"=inf, "B-8, 11"=610.0, "C-1, 12"=-500.0, "C-3, 13"=-500.0, "C-4, 14"=-3.0, "C-5,  15"=inf, "C-8, 16"=610.0, "D-1, 17"=-150.0, "D-3, 18"=-250.0, "D-4,  19"=-500.0, "D-5,  20"=610.0, "D-8,  21"=910.0}, "High AD Diff "={"A-1, 1"=FALSE, "A-3, 2"=FALSE, "A-4, 3"=FALSE, "A-5, 4"=TRUE, "ABCD-7, 5"=FALSE, "A-8, 6"=TRUE, "B-1,  7"=FALSE, "B-3, 8"=FALSE, "B-4, 9"=FALSE, "B-5, 10"=TRUE, "B-8,  11"=TRUE, "C-1, 12"=FALSE, "C-3, 13"=FALSE, "C-4,  14"=FALSE, "C-5,  15"=TRUE, "C-8, 16"=TRUE, "D-1, 17"=FALSE, "D-3, 18"=FALSE, "D-4, 19"=FALSE, "D-5,  20"=TRUE, "D-8,  21"=TRUE}, "Delay S"={"A-1,  1"=30.0, "A-3,  2"=30.0, "A-4, 3"=1.0, "A-5, 4"=1.0, "ABCD-7, 5"=1.0, "A-8, 6"=1.0, "B-1,  7"=30.0, "B-3, 8"=30.0, "B-4,  9"=1.0, "B-5, 10"=1.0, "B-8, 11"=1.0, "C-1, 12"=30.0, "C-3, 13"=30.0, "C-4, 14"=1.0, "C-5,  15"=1.0, "C-8, 16"=1.0, "D-1, 17"=30.0, "D-3, 18"=30.0, "D-4,  19"=30.0, "D-5,  20"=1.0, "D-8,  21"=1.0}}  # Hyperoxic AD Settings
                w197 = T3 {"Run C1"={"A-1,  1"=inf, "A-3,  2"=inf, "A-4, 3"=9600.0, "A-5, 4"=8800.0, "ABCD-7, 5"=9800.0, "A-8, 6"=9800.0, "B-1,  7"=3400.0, "B-3, 8"=3400.0, "B-4,  9"=9600.0, "B-5, 10"=8800.0, "B-8, 11"=9800.0, "C-1, 12"=1800.0, "C-3, 13"=1800.0, "C-4, 14"=9600.0, "C-5,  15"=8800.0, "C-8, 16"=9800.0, "D-1, 17"=inf, "D-3, 18"=3400.0, "D-4,  19"=1800.0, "D-5,  20"=9800.0, "D-8,  21"=9800.0}, "Run C2"={"A-1,  1"=inf, "A-3,  2"=inf, "A-4, 3"=9500.0, "A-5, 4"=8600.0, "ABCD-7, 5"=9700.0, "A-8, 6"=9700.0, "B-1,  7"=3000.0, "B-3, 8"=3000.0, "B-4,  9"=9500.0, "B-5, 10"=8600.0, "B-8, 11"=9700.0, "C-1, 12"=1400.0, "C-3, 13"=1400.0, "C-4, 14"=9500.0, "C-5,  15"=8600.0, "C-8, 16"=9700.0, "D-1, 17"=inf, "D-3, 18"=3000.0, "D-4,  19"=1400.0, "D-5,  20"=9700.0, "D-8,  21"=9700.0}, "Hold C3"={"A-1,  1"=1800.0, "A-3,  2"=1800.0, "A-4, 3"=9000.0, "A-5, 4"=8800.0, "ABCD-7, 5"=9800.0, "A-8, 6"=9800.0, "B-1,  7"=3400.0, "B-3, 8"=3400.0, "B-4,  9"=9000.0, "B-5, 10"=8800.0, "B-8, 11"=9800.0, "C-1, 12"=1800.0, "C-3, 13"=1800.0, "C-4, 14"=9000.0, "C-5,  15"=8800.0, "C-8, 16"=9800.0, "D-1, 17"=1800.0, "D-3, 18"=3400.0, "D-4,  19"=1800.0, "D-5,  20"=9800.0, "D-8,  21"=9800.0}, "Hold C4"={"A-1,  1"=1400.0, "A-3,  2"=1400.0, "A-4, 3"=8800.0, "A-5, 4"=8600.0, "ABCD-7, 5"=9700.0, "A-8, 6"=9700.0, "B-1,  7"=3000.0, "B-3, 8"=3000.0, "B-4,  9"=8800.0, "B-5, 10"=8600.0, "B-8, 11"=9700.0, "C-1, 12"=1400.0, "C-3, 13"=1400.0, "C-4, 14"=8800.0, "C-5,  15"=8600.0, "C-8, 16"=9700.0, "D-1, 17"=1400.0, "D-3, 18"=3000.0, "D-4,  19"=1400.0, "D-5,  20"=9700.0, "D-8,  21"=9700.0}, "High CO2 Forces"={"A-1, 1"=TRUE, "A-3, 2"=TRUE, "A-4, 3"=FALSE, "A-5, 4"=TRUE, "ABCD-7, 5"=FALSE, "A-8, 6"=TRUE, "B-1,  7"=TRUE, "B-3, 8"=TRUE, "B-4, 9"=FALSE, "B-5, 10"=TRUE, "B-8,  11"=TRUE, "C-1, 12"=TRUE, "C-3, 13"=TRUE, "C-4,  14"=FALSE, "C-5,  15"=TRUE, "C-8, 16"=TRUE, "D-1, 17"=TRUE, "D-3, 18"=TRUE, "D-4, 19"=TRUE, "D-5,  20"=TRUE, "D-8,  21"=TRUE}}  # Hyperoxic CO2 Settings
                n66 = call <userlib>:"Read Section Cluster__ogtk.vi"("Section Formatted Cluster Type"=w197, "refnum"=w196) -> ("error out"=w201:errorcluster, "all found?"=w194:bool, "Section Formatted Cluster"=w203:variant, "dup refnum"=w202:T27)  [unwired: 5 in, 1 out]
                n67 = Variant To Data(error in=w201, type=w197, Variant=w203) -> (data=w192:T3, error out=w200:errorcluster)
                n68 = call <userlib>:"Read Section Cluster__ogtk.vi"("error in (no error)"=w200, "Section Formatted Cluster Type"=w198, "refnum"=w202) -> ("error out"=w199:errorcluster, "all found?"=w195:bool, "Section Formatted Cluster"=w204:variant)  [unwired: 4 in, 2 out]
                n69 = Variant To Data(error in=w199, type=w198, Variant=w204) -> (data=w193:T6)  [unwired: 1 out]
              }
              frame #3 {
                w215 = "System" ("section")
                # "HANDLE CHECKING OF CODES"
                n70 = call-poly <vilib>:"Read Key.vi"("section"=w215, "error in (no error)"=w223, "key"="dt", "refnum"=w233) -> ("error out"=w218:errorcluster, "value"=w228:dbl, "refnum out"=w221:T27)  [unwired: 4 in, 1 out]
                n71 = In Range and Coerce(upper limit=24.0, x=w228, lower limit=-24.0) -> (coerced(x)=w225:dbl)  [unwired: 1 out]
                n72 = call "Dimmer FG.vi"("Operation"=enum16{"Init", "Run", "Close Ref"}."Init") -> ("error out"=w205:errorcluster)  [unwired: 10 in]
                n73 = call-poly <vilib>:"Read Key.vi"("section"=w215, "error in (no error)"=w218, "default value"=100, "key"="dim", "refnum"=w221) -> ("error out"=w212:errorcluster, "value"=w217:i32, "found?"=w207:bool, "refnum out"=w214:T27)  [unwired: 3 in]
                n74 = To Byte Integer(number=w217) -> (8bit integer=w206:i8)
                n75 = local write "dimmer"(w206) -> ()
                n76 = call-poly <vilib>:"Read Key.vi"("section"=w215, "error in (no error)"=w212, "default value"=FALSE, "key"="altDisplay", "refnum"=w214) -> ("error out"=w211:errorcluster, "value"=w208:bool, "refnum out"=w213:T27)  [unwired: 3 in, 1 out]
                n77 = property on="dimmer" class="Slide (strict)"(error in=w205, "Val(Sgnl)"=w206) -> ()  [unwired: 1 in, 2 out]
                n78 = To Double Precision Float(number=w225) -> (double precision float=w224:dbl)
                n79 = Multiply(x=w224, y=3600.0) -> (x*y=w230:dbl)
                n80 = property on="Time Offset (h)" class="DigNum (strict)"(error in=w211, "Value"=w225) -> (error out=w222:errorcluster)  [unwired: 1 in, 1 out]
                n81 = property on="ALT Window ON/OFF" class="Bool (strict)"("Value"=w208) -> ()  [unwired: 2 in, 2 out]
                n82 = call "Check Ordered Hash.vi"("error in"=w222, "refnum"=w213) -> ("error out"=w235:errorcluster, "Key"=→"SN#":string, "Canceled?"=w236:bool, "refnum out"=w237:T27, "Sorted Data"=w229:T32)  [unwired: 5 in]
                n83 = call <vilib>:"Close Config Data.vi"("error in (no error)"=w235, "refnum"=w237) -> ()  [unwired: 8 in, 2 out]
              }
            }
          }
          frame Error {
          }
        }
        n84 = local write "hyperCO2"(w73) -> ()
        n85 = local write "hypCO2"(w74) -> ()
        n86 = Build Array(w74, w73) -> (w75:T3[])
        n87 = local write "hypAD"(w72) -> ()
        n88 = local write "hyperAD"(w71) -> ()
        n89 = Build Array(w72, w71) -> (w76:T6[])
        n90 = Unbundle By Name(w80) -> ("Key Valid?"=w79:bool[])
        n91 = case shown="True" w82 {
          tunnel: w84 -> [w92 w94]
          frame False {
            n92 = Enqueue Element(queue=w92, element="UI: Initialize" ("f")) -> ()  [unwired: 2 in, 3 out]
          }
          frame True {
            n93 = Enqueue Element(queue=w94, element="Stop" ("f")) -> ()  [unwired: 2 in, 3 out]
          }
        }
        n94 = local write "reset"(w82) -> ()
        n95 = Index Array(array=w79) -> (element=w78:bool)  [unwired: 1 in]
        n96 = Not(x=w78) -> (.not. x?=w77:bool)
        n97 = property on="eCode" class="Bool"("Visible"=w77) -> ()  [unwired: 2 in, 2 out]
      }
      frame "UI: Initialize" {
        w267 = u16 1 ("Front Panel Window:Monitor")
        w277 = 1800 ("History")
        w291 = FALSE ("Visible")
        w290 = T28."Enabled" ("Disabled")
        w292 = FALSE ("Stop Button")
        # "180 minutes."
        n98 = control-ref of="Level 0"() -> (w302:refnum<vi>)
        n99 = control-ref of="Level 1"() -> (w301:refnum<vi>)
        n100 = control-ref of="Level 2"() -> (w300:refnum<vi>)
        n101 = control-ref of="Level 3"() -> (w299:refnum<vi>)
        n102 = Enqueue Element(queue=w287, element="Controller: Initialize") -> ()  [unwired: 2 in, 3 out]
        n103 = Build Array(w302, w301, w300, w299) -> (w303:refnum<vi>[])
        n104 = for {
          tunnel: w303 -> [w306] mode=indexing
          i -> [w305]
          # "SET ONLY LEVEL 0 VISIBLE"
          n105 = Equal To 0?(x=w305) -> (x = 0?=w304:bool)
          n106 = property class="Clust"(reference=w306, "Visible"=w304) -> ()  [unwired: 1 in, 2 out]
        }
        n107 = property on="CO2 Points" class="DigNum (strict)"("Value"=w277) -> ()  [unwired: 2 in, 2 out]
        n108 = property on="pAltitude" class="Multivalue Buffer (strict)"("History"=w277, "PlotSize"=cluster{"Height":i32, "Width":i32} {"Height"=475, "Width"=200}, "Format"="%5.1f") -> ()  [unwired: 2 in, 2 out]
        n109 = property on="Alt Points" class="DigNum (strict)"("Value"=w277) -> ()  [unwired: 2 in, 2 out]
        n110 = control-ref of="This VI"() -> (w269:refnum<vi>)
        n111 = property on="CO2Buffer" class="Multivalue Buffer (strict)"("History"=w277, "PlotSize"=cluster{"Height":i32, "Width":i32} {"Height"=250, "Width"=180}, "Axis Name"="CO2", "Autoscale?"=u8 0, "Min"=0.0 ("Increment"), "Increment"=0.1 ("Min"), "Max"=1.0, "Precision"=u8 1, "Format"="%1.1f") -> ()  [unwired: 2 in, 2 out]
        n112 = local write "senseConn"(w292) -> ()
        n113 = local write "reset"(w292) -> ()
        n114 = property on="Calibrating" class="Bool (strict)"("Blinking"=w292, "Value"=w292) -> ()  [unwired: 2 in, 2 out]
        n115 = local write "writetofile"(FALSE ("WritetoFile")) -> ()
        n116 = property on="ALT SET" class="Clust (strict)"("DisabledEnum"=w290) -> ()  [unwired: 2 in, 2 out]
        n117 = property on="ALT SET 2" class="Clust (strict)"("DisabledEnum"=w290) -> ()  [unwired: 2 in, 2 out]
        n118 = property class="VI"(reference=w269, "FP.Monitor"=w267, "Front Panel.TitleBarVis"=FALSE ("Front Panel Window:Title Bar Visible"), "Front Panel.IsFrontmost"=TRUE ("Front Panel Window:Is Frontmost"), "FP.State"=T25."Maximized" ("Front Panel Window:State"), "FP.Monitor"=w267) -> (error out=w240:errorcluster, "Front Panel.PanelBounds"=w266:T33)  [unwired: 1 in, 1 out]
        n119 = property on="Main States" class="TabCtl (strict)"(error in=w240) -> ("Width"=w263:u32, "Height"=w255:u32)  [unwired: 1 in, 2 out]
        n120 = Unbundle By Name(w266) -> ("Right"=w265:i16, "Left"=w257:i16, "Bottom"=w258:i16, "Top"=w243:i16)
        n121 = property on="Stop" class="Bool (strict)"("Value"=FALSE) -> ()  [unwired: 2 in, 2 out]
        n122 = property on="Confirm Now" class="Bool (strict)"("Visible"=w291) -> ()  [unwired: 2 in, 2 out]
        n123 = property on="Confirm Now 2" class="Bool (strict)"("Visible"=w291) -> ()  [unwired: 2 in, 2 out]
        n124 = Subtract(x=w258, y=w243) -> (x-y=w256:i16)
        n125 = local write "Version"("Version Not Good" ("Version")) -> ()
        n126 = Subtract(x=w265, y=w257) -> (x-y=w264:i16)
        n127 = Subtract(x=w256, y=w255) -> (x-y=w253:u32)
        n128 = Subtract(x=w264, y=w263) -> (x-y=w262:u32)
        n129 = Divide(x=w262, y=u32 2) -> (x/y=w241:dbl)
        n130 = Divide(x=w253, y=u32 2) -> (x/y=w242:dbl)
        n131 = property on="Main States" class="TabCtl (strict)" props=["Left", "Top", "Width", "Height"]("Left"=w241, "Top"=w242) -> ("Width"=w252:u32)  [unwired: 2 in, 3 out]
        n132 = property on="sysStat" class="Bool (strict)"() -> ("Width"=w250:u32)  [unwired: 2 in, 2 out]
        n133 = Add(x=u32 8 ("y"), y=w250) -> (x+y=w248:u32)
        n134 = Add(x=w241, y=w252) -> (x+y=w251:dbl)
        n135 = Subtract(x=w251, y=w248) -> (x-y=w247:dbl)
        n136 = Add(x=27.0, y=w242) -> (x+y=w245:dbl)
        n137 = property on="sysStat" class="Bool (strict)"("Left"=w247, "Top"=w245) -> ()  [unwired: 2 in, 2 out]
        n138 = property on="Main Tabs" class="TabCtl (strict)"("Visible"=FALSE, "Top"=w242, "Left"=w241) -> ()  [unwired: 2 in, 2 out]
        "sysStat" <- FALSE ("sysStat")
      }
      frame "Controller: Initialize" {
        # "Don't indicate that there is a sensor connection error here.  We need to register that when attempting to go to a state other than OFF."
        n139 = call "Search for Valid Port.vi"() -> ("Version"=→"Version":string, "Port Out"=w324:refnum<visa-resource-name>)  [unwired: 9 in, 1 out]
        n140 = Enqueue Element(queue=w313, element="Idle") -> ()  [unwired: 2 in, 3 out]
        n141 = flat-sequence {
          tunnel: w324 -> [w336]
          tunnel: [w334] -> w325
          frame #0 {
            n142 = control-ref of="Mode"() -> (w337:refnum<vi>)
            n143 = control-ref of="ALT SET"() -> (w338:refnum<vi>)
            n144 = control-ref of="Confirm Now"() -> (w340:refnum<vi>)
            n145 = Bundle("Mode"=w337, "ALT SET"=w338, "Confirm Now"=w340) -> (w335:T34)  [unwired: 1 in]
            n146 = call "Handle Serial Errors.vi"("GV State"=enum16{"Init", "Test"}."Init", "Ctl Refs"=w335, "Port"=w336) -> ("Port 2"=w334:refnum<visa-resource-name>)  [unwired: 5 in, 3 out]
          }
        }
        n147 = property class="File"(reference=refnum<class "File.lvclass"> refnum ("File"), "Main Path"=path "C:/", "Max File Size (bytes)"=i64 50000000, "Data Folder"="CAT Panel Data", "Write?"=FALSE) -> (reference out=w318:refnum<class "File.lvclass">, error out=w315:errorcluster)  [unwired: 1 in]
        n148 = Index Array(array=w309) -> (element=w308:T6)  [unwired: 1 in]
        n149 = Unbundle By Name(w308) -> ("Delay S"=w329:T4)
        n150 = Cluster To Array(cluster=w329) -> (array=w330:dbl[])
        n151 = for {
          tunnel: w330 -> [w331] mode=indexing
          tunnel: refnum<class "Output Timer.lvclass"> refnum ("Delay Timer") -> [w333]
          tunnel: [w332] -> w328 mode=indexing
          n152 = property class="Delay Timer"(reference=w333, "Delay"=w331) -> (reference out=w332:refnum<class "Output Timer.lvclass">)  [unwired: 1 in, 1 out]
        }
      }
      frame "Controller: Update Mode" {
        w356 = T35 {"Main 1"=FALSE, "Main 2"=FALSE, "Recirc  3"=FALSE, "Boost A 7"=FALSE, "Recirc  9"=FALSE, "Scrub 4"=FALSE, "Scrub 10"=FALSE, "O2 5"=FALSE, "Vent 6"=FALSE, "Boost A 8"=FALSE, "Vent 11"=FALSE, "Boost B 12"=FALSE, "Boost B 13"=FALSE, "Recirc 14"=FALSE, "Scrub 15"=FALSE, "Vent 16"=FALSE, "Main 17"=FALSE, "Boost A 18"=FALSE, "Boost B 19"=FALSE, "Boost F 20"=FALSE, "Vent 2 21"=FALSE}  # All Off
        # "The mode has no side effects and therefore the outputs from this case do not have to be populated each iteration - only the iteration prior to contacting the controller."
        n153 = local read "altSp"() -> (w344:dbl)
        n154 = local read "locElev"() -> (w343:dbl)
        n155 = Less?(x=w344, y=w343) -> (x < y?=w341:bool)
        n156 = local read "Alt Dif"() -> (w342:dbl)
        n157 = Boolean To (0,1)(Boolean=w341) -> (0, 1=w345:i16)
        n158 = Unbundle By Name(w372) -> ("CO2- ppm"=w355:u32)
        n159 = Index Array(array=w346, index=w345) -> (element=w347:T3)
        n160 = local read "Mode"() -> (w366:enum8{"Off", "Stby", "Hold", "Run"})
        n161 = Index Array(array=w349, index=w345) -> (element=w348:T6)
        n162 = feedback #2(w356) -> (w357:T35)
        n163 = feedback #3(w356) -> (w359:T35)
        n164 = case shown="\"Off\", Default" w366 {
          tunnel: w355 -> [w402 w426 _ _]
          tunnel: [w391 w417 w430 _] -> w360
          tunnel: w359 -> [w381 w415 _ _]
          tunnel: [w396 w422 w430 _] -> w365
          tunnel: w342 -> [w397 w423 _ _]
          tunnel: [w395 w421 w430 _] -> w358
          tunnel: w357 -> [w379 w405 _ _]
          tunnel: [w392 w418 w430 w433] -> w364
          tunnel: w373 -> [w376 _ _ _]
          tunnel: [w390 w416 w430 w433] -> w363
          tunnel: w347 -> [w389 w413 _ _]
          tunnel: w348 -> [w385 w409 _ _]
          tunnel: ["Controller: Get Data" ("t") "Controller: Get Data" ("t") "Controller: Get Data" ("t") "Idle"] -> w351
          frame "Run" {
            n165 = Unbundle By Name(w385) -> ("Set Point Force"=w375:T4, "Run A1"=w384:T4, "Run A2"=w383:T4, "High AD Diff"=w382:T5)
            n166 = Unbundle By Name(w389) -> ("Run C1"=w388:T4, "Run C2"=w387:T4, "High CO2 Forces"=w386:T5)
            n167 = Greater?(x=w376, y=w375) -> (0:w377:T36)
            n168 = Greater?(x=w397, y=w383) -> (0:w378:T36)
            n169 = And(x=w378, y=w379) -> (x .and. y?=w398:T37)
            n170 = Greater?(x=w397, y=w384) -> (0:w399:T36)
            n171 = Greater?(x=w402, y=w388) -> (0:w401:T36)
            n172 = Greater?(x=w402, y=w387) -> (0:w380:T36)
            n173 = Or(x=w399, y=w398) -> (x .or. y?=w395:T37)
            n174 = And(x=w380, y=w381) -> (x .and. y?=w400:T37)
            n175 = And(x=w395, y=w382) -> (x .and. y?=w394:T5)
            n176 = Or(x=w401, y=w400) -> (x .or. y?=w391:T37)
            n177 = Not Or(1:w382, 2:w395) -> (0:w393:T5)
            n178 = And(x=w391, y=w386) -> (x .and. y?=w396:T5)
            n179 = Not(x=w391) -> (.not. x?=w390:T37)
            n180 = Compound Arithmetic op=OR(w377, w394, w393) -> (w392:T5)
          }
          frame "Hold" {
            n181 = Unbundle By Name(w409) -> ("Hold A3"=w408:T4, "Hold A4"=w407:T4, "High AD Diff"=w406:T5)
            n182 = Unbundle By Name(w413) -> ("Hold C3"=w412:T4, "Hold C4"=w411:T4, "High CO2 Forces"=w410:T5)
            n183 = Greater?(x=w423, y=w408) -> (0:w425:T36)
            n184 = Greater?(x=w423, y=w407) -> (0:w404:T36)
            n185 = Greater?(x=w426, y=w412) -> (0:w428:T36)
            n186 = Greater?(x=w426, y=w411) -> (0:w414:T36)
            n187 = And(x=w404, y=w405) -> (x .and. y?=w424:T37)
            n188 = And(x=w414, y=w415) -> (x .and. y?=w427:T37)
            n189 = Or(x=w425, y=w424) -> (x .or. y?=w421:T37)
            n190 = Or(x=w428, y=w427) -> (x .or. y?=w417:T37)
            n191 = And(x=w417, y=w410) -> (x .and. y?=w422:T5)
            n192 = And(x=w421, y=w406) -> (x .and. y?=w419:T5)
            n193 = Not(x=w417) -> (.not. x?=w416:T37)
            n194 = Not Or(1:w406, 2:w421) -> (0:w420:T5)
            n195 = Or(x=w420, y=w419) -> (x .or. y?=w418:T5)
          }
          frame "Stby" {
            w430 = T35 {"Main 1"=FALSE, "Main 2"=FALSE, "Recirc  3"=FALSE, "Boost A 7"=FALSE, "Recirc  9"=FALSE, "Scrub 4"=FALSE, "Scrub 10"=FALSE, "O2 5"=FALSE, "Vent 6"=FALSE, "Boost A 8"=FALSE, "Vent 11"=FALSE, "Boost B 12"=FALSE, "Boost B 13"=FALSE, "Recirc 14"=FALSE, "Scrub 15"=FALSE, "Vent 16"=FALSE, "Main 17"=FALSE, "Boost A 18"=FALSE, "Boost B 19"=FALSE, "Boost F 20"=FALSE, "Vent 2 21"=FALSE}
          }
          frame "Off", Default {
            w433 = T35 {"Main 1"=FALSE, "Main 2"=FALSE, "Recirc  3"=FALSE, "Boost A 7"=FALSE, "Recirc  9"=FALSE, "Scrub 4"=FALSE, "Scrub 10"=FALSE, "O2 5"=FALSE, "Vent 6"=FALSE, "Boost A 8"=FALSE, "Vent 11"=FALSE, "Boost B 12"=FALSE, "Boost B 13"=FALSE, "Recirc 14"=FALSE, "Scrub 15"=FALSE, "Vent 16"=FALSE, "Main 17"=FALSE, "Boost A 18"=FALSE, "Boost B 19"=FALSE, "Boost F 20"=FALSE, "Vent 2 21"=FALSE}
            n196 = property on="sysStat" class="Bool (strict)"("Blinking"=FALSE ("sysStat")) -> ()  [unwired: 2 in, 2 out]
          }
        }
        n197 = feedback-in #2(w358) -> ()
        n198 = feedback-in #3(w360) -> ()
        n199 = local read "Final  Output Names"() -> (w354:T11)
        n200 = Enqueue Element(queue=w350, element=w351) -> ()  [unwired: 2 in, 3 out]
        n201 = And(x=w363, y=w364) -> (x .and. y?=w362:T5)
        n202 = Or(x=w362, y=w365) -> (x .or. y?=w370:T5)
        "Final Output" <- w370
        n203 = call "Names 2 Outputs.vi"("Final  Output In"=w354, "Final  Output"=w370) -> ("Final  Output Out"=→"Final  Output Names":T11)  [unwired: 3 in]
      }
      frame "Controller: Get Data" {
        w444 = 0
        n204 = Cluster To Array(cluster=w462) -> (array=w447:bool[])
        n205 = for {
          tunnel: w464 -> [w469] mode=indexing
          tunnel: w447 -> [w468] mode=indexing
          tunnel: [w467] -> w463 mode=indexing
          tunnel: [w466] -> w460 mode=indexing
          n206 = call "Process Request.vi"("Requested"=w468, "Delay Timer in"=w469) -> ("Returned"=w466:bool, "Delay Timer out"=w467:refnum<class "Output Timer.lvclass">)  [unwired: 7 in, 1 out]
        }
        n207 = Array To Cluster(array=w460) -> (cluster=w459:T38)
        n208 = call "Call Engine.vi"("Other Outputs"="Other Outputs", "Final Output Controls"=w459, "Port"=w465) -> ("error out"=w452:errorcluster, "Data Not Good"=w446:bool, "VISA resource name out"=w458:refnum<visa-resource-name>, "Data Read"=w457:T39)  [unwired: 2 in]
        n209 = feedback #4(w444) -> (w445:i32)
        n210 = Select(t=w445, s=w446, f=w444) -> (s? t:f=w443:i32)
        n211 = Increment(x=w443) -> (x+1=w441:i32)
        n212 = Greater Or Equal?(x=w441, y=2) -> (x >= y?=w438:bool)
        "senseConn" <- w438
        n213 = Select(t=w456, s=w446, f=w457) -> (s? t:f=w455:T26)
        n214 = Select(t=0, s=w438, f=w441) -> (s? t:f=w439:i32)
        n215 = feedback-in #4(w439) -> ()
        n216 = Select(t="Controller: Comm Error" ("f"), s=w438, f="UI: Update") -> (s? t:f=w451:string)
        n217 = Enqueue Element(queue=w450, element=w451) -> ()  [unwired: 2 in, 3 out]
      }
      frame "UI: Update" {
        w496 = sgl 10.0 ("y")
        # "Update the UI - only executes if the Controller: Get Data case finished successfully."
        n218 = Enqueue Element(queue=w515, element="UI: Check Alarms" ("f")) -> ()  [unwired: 2 in, 3 out]
        n219 = Unbundle By Name(w518) -> ("CO2- ppm"=w510:u32, "O2-1 ppm"=w474:u32, "O2-2 ppm"=w473:u32, "Press mB"=w478:sgl, "Date"=w503:string, "Time"=w502:string, "Temp MB"=w506:sgl)
        "CO2 ppm" <- w510
        "Press mB" <- w478
        "Temp C" <- w506
        n220 = feedback #5() -> ()  [unwired: 2 in]
        n221 = call "Convert Date_Time.vi"("Time"=w502, "Date"=w503) -> ("time stamp"=w494:timestamp)  [unwired: 8 in, 1 out]
        n222 = To Single Precision Float(number=w510) -> (single precision float=w523:sgl)
        n223 = Unbundle By Name("Level 1") -> ("Feet OFF/ Meters ON"=w476:bool)
        n224 = Unbundle By Name("Level 2") -> ("West ON/Std OFF"=w477:bool)
        n225 = Divide(x=w523, y=sgl 10000.0) -> (x/y=w500:sgl)
        "CO2_0" <- w500
        "CO2_1" <- w500
        n226 = local read "Mode"() -> (w470:enum8{"Off", "Stby", "Hold", "Run"})
        n227 = Build Array(w500) -> (w499:sgl[])
        n228 = call "Altitude Composite.vi"("Feet OFF/ Meters ON"=w476, "West ON/Std OFF"=w477, "Pressure mBar"=w478) -> ("Alt Eff correct"=→"locElev":dbl)  [unwired: 3 in, 5 out]
        n229 = call "Altitude Composite.vi"("Feet OFF/ Meters ON"=w476, "West ON/Std OFF"=w477, "Mode"=w470, "Pressure mBar"=w478, "O2ppm-2"=w473, "O2ppm-1"=w474) -> ("Alt Eff correct"=w481:dbl, "O2%-2"=w483:dbl, "O2%-1"=w482:dbl, "System Status Out"=w472:bool, "Mean O2%"=w479:dbl)  [unwired: 1 out]
        "altDisp1" <- w481
        "Altitude" <- w481
        "altDisp2" <- w481
        "altDisp1 2" <- w481
        n230 = Not(x=w472) -> (.not. x?=w471:bool)
        n231 = feedback-in #5(w471) -> ()
        n232 = property on="O2-1 (%)" class="DigNum (strict)"("Value"=w482) -> ()  [unwired: 2 in, 2 out]
        n233 = property on="sysStat" class="Bool (strict)"("Blinking"=w472) -> ()  [unwired: 2 in, 2 out]
        n234 = property on="O2-2 (%)" class="DigNum (strict)"("Value"=w483) -> ()  [unwired: 2 in, 2 out]
        n235 = Add(x=w494, y=w495) -> (x+y=w492:timestamp)
        "Time" <- w492
        n236 = property on="Buffer" class="DigNum (strict)" props=["Value"]() -> ()  [unwired: 2 in, 3 out]
        n237 = property on="Buffer" class="DigNum (strict)"() -> ("Value"=w488:dbl)  [unwired: 2 in, 2 out]
        n238 = Multiply(x=w479, y=w496) -> (x*y=w498:dbl)
        n239 = Build Array(w481) -> (w505:dbl[])
        n240 = Round Toward -Infinity(1:w498) -> (0:w497:dbl)
        n241 = Subtract(x=w481, y=w520) -> (x-y=→"Alt Dif":dbl)
        n242 = Divide(x=w497, y=w496) -> (x/y=→"O2%":dbl)
        n243 = Bundle(w492, w499) -> (→"CO2Buffer":cluster{timestamp, sgl[]})  [unwired: 1 in]
        n244 = Bundle(w492, w505) -> (→"pAltitude":cluster{timestamp, dbl[]})  [unwired: 1 in]
        n245 = Format Into String(format string="%s\t%s\t%d\t%d\t%d\t%f\t%f\r\n", w503, w502, w510, w474, w473, w478, w506) -> (resulting string=w508:string, error out=w507:errorcluster)  [unwired: 2 in]
        n246 = Less?(x=w492, y=timestamp(3471404400 s since 1904-01-01)) -> (x < y?=w490:bool)
        n247 = call "Calculate Min Alt.vi"("Meters?"=w476, "Buffer (0-1)"=w488, "P (mb)"=w478) -> ("Max O2"=→"maxO2":dbl, "Altitude"=→"minAlt":dbl)  [unwired: 7 in]
        n248 = call-dynamic "Write to File.vi"("error in"=w507, "DataIn"=w508, "File in"=w512) -> ("File out"=w511:refnum<class "File.lvclass">)  [unwired: 7 in, 1 out]
        n249 = case shown="True" w490 {
          frame False {
          }
          frame True {
            n250 = property on="Mode" class="VertMode (strict)"("Val(Sgnl)"=enum8{"Off", "Stby", "Hold", "Run"}."Off" ("Value (Signaling)")) -> ()  [unwired: 2 in, 2 out]
            n251 = One Button Dialog(message="Problem with controller.  Switching mode to OFF.  Contact Colorado Altitude Trainers for service information.") -> ()  [unwired: 1 in, 1 out]
          }
        }
      }
      frame "UI: Check Alarms" {
        # "23.45/sqrt(P/1013.25)"
        # "This is the mean difference for the last 100 sensor readings.  The difference is between the two O2 sensors."
        # "Check here for things such as sensor errors and report them to the UI.  The errors are based on limits defined in the configuration file or in the setup menu."
        n252 = Unbundle By Name(w570) -> ("O2-1 ppm"=w558:u32, "O2-2 ppm"=w557:u32, "Press mB"=w534:sgl)
        n253 = Enqueue Element(queue=w550, element="Idle") -> ()  [unwired: 2 in, 3 out]
        n254 = local read "Level 3"() -> (w566:T19)
        n255 = Unbundle By Name(w566) -> ("Alarm Points.CalLimit"=w564:sgl, "Alarm Points.SenseLimit"=w562:sgl, "Alarm Points.CO2Lim"=w556:sgl, "Alarm Points.AltLim"=w555:sgl, "Alarm Points.O2 Low"=w552:sgl, "Alarm Points.O2 High"=w528:sgl)
        n256 = To Double Precision Float(number=w558) -> (double precision float=w560:dbl)
        n257 = To Double Precision Float(number=w557) -> (double precision float=w561:dbl)
        n258 = Divide(x=w534, y=sgl 1013.25) -> (x/y=w532:sgl)
        n259 = Subtract(x=w560, y=w561) -> (x-y=w559:dbl)
        n260 = Square Root(x=w532) -> (sqrt(x)=w531:sgl)
        n261 = Divide(x=sgl 23.45, y=w531) -> (x/y=w529:sgl)
        n262 = Absolute Value(x=w559) -> (abs(x)=w565:dbl)
        n263 = Add(x=w528, y=w529) -> (x+y=w527:sgl)
        n264 = local read "Altitude"() -> (w554:sgl)
        n265 = feedback #6(TRUE) -> (w567:bool)
        n266 = call <vilib>:"Mean PtByPt.vi"("x"=w565, "sample length"=100, "initialize"=w567) -> ("mean"=w563:dbl)  [unwired: 1 in, 1 out]
        "meanDiff" <- w563
        n267 = feedback-in #6(FALSE) -> ()
        n268 = local read "O2%"() -> (w551:sgl)
        n269 = local read "O2%"() -> (w547:sgl)
        n270 = Greater?(x=w554, y=w555) -> (0:w543:bool)
        "Altitude" <- w543
        n271 = local read "CO2_0"() -> (w553:sgl)
        n272 = Less?(x=w551, y=w552) -> (x < y?=w542:bool)
        "Low O2 Level" <- w542
        n273 = Greater?(x=w547, y=w527) -> (0:w540:bool)
        "High O2 Level" <- w540
        n274 = Greater?(x=w563, y=w564) -> (0:w546:bool)
        "Calibrate" <- w546
        n275 = Greater?(x=w553, y=w556) -> (0:w544:bool)
        "CO2 Level" <- w544
        n276 = Greater?(x=w563, y=w562) -> (0:w545:bool)
        "Sensor Error" <- w545
        n277 = local read "senseConn"() -> (w539:bool)
        n278 = Compound Arithmetic op=OR(w539, w546, w545, w544, w543, w542, w540) -> (w541:bool)
        n279 = local write "sysStat"(w541) -> ()
      }
      frame "Controller: Comm Error" {
        # "The sysStat variable will be overriden by the Sensor Connection error.  The reason for this is that the sensor connection will not be checked on the general alarms page because the general alarms are not checked when the system is OFF (which is what it will be if there is an error)."
        # "Handle Comm errors thrown on the last attempt to get data."
        n280 = Equal?(x=w587, y="Controller: Get Data") -> (x = y?=w585:bool)
        n281 = call "Handle Serial Errors.vi"("GV State"=enum16{"Init", "Test"}."Test", "error in"=w597, "Port"=w599) -> ("Version"=w590:string, "Reconnect?"=w591:bool, "Port 2"=w598:refnum<visa-resource-name>)  [unwired: 5 in, 1 out]
        n282 = local write "senseConn"(w591) -> ()
        n283 = local write "sysStat"(w591) -> ()
        n284 = call "Elapsed Time3"("Time Target (s)"=180.0, "Reset"=w585, "Auto Reset"=FALSE) -> ("Time has Elapsed"=w582:bool)  [unwired: 9 in, 7 out]
        n285 = case shown="False" w591 {
          tunnel: w590 -> [w603 _]
          frame False {
            n286 = local write "Version"(w603) -> ()
          }
          frame True {
          }
        }
        n287 = Select(t="Stop", s=w582, f="Idle") -> (s? t:f=w579:string)
        n288 = Enqueue Element(queue=w595, element=w579) -> ()  [unwired: 2 in, 3 out]
        n289 = case shown="\"Stop\"" w579 {
          frame "False", Default {
          }
          frame "Stop" {
            n290 = local write "reset"(TRUE ("reset")) -> ()
          }
        }
      }
      frame "Controller: Calibrate" {
        # "NEED A WAY TO HANDLE CALS HERE - SHOULD NOT DO THE STANDARD CHECKING BUT NEED TO READ BASED ON THE FACT THAT THE CONTROLLER IS IN CALIBRATION MODE..."
        n291 = case shown="True" w613 {
          tunnel: [w626 w630] -> w610
          tunnel: w615 -> [w626 w632]
          tunnel: [TRUE w631] -> w611
          frame False {
          }
          frame True {
            # "READ FROM PORT IF COMMAND ISSUED"
            n292 = property class="Instr"(reference=w632) -> (reference out=w636:refnum<visa-resource-name>, error out=w627:errorcluster, "Bytes at Port"=w633:u32)  [unwired: 1 in]
            n293 = VISA Read(VISA resource name=w636, byte count=w633, error in (no error)=w627) -> (VISA resource name out=w630:refnum<visa-resource-name>, read buffer=w628:string, error out=w634:errorcluster)  [unwired: 1 out]
            n294 = call <vilib>:"Trim Whitespace.vi"("string"=w628) -> ("trimmed string"=w629:string)  [unwired: 1 in]
            n295 = call "Parse Cal String.vi"("error in (no error)"=w634, "read buffer in"=w629) -> ("CAL Complete"=w635:bool)  [unwired: 1 in, 2 out]
            n296 = Not(x=w635) -> (.not. x?=w631:bool)
          }
        }
        "Calibrating" <- w611
        n297 = case shown="False" w611 {
          tunnel: w610 -> [w620 w623]
          tunnel: [w620 w622] -> w614
          tunnel: [_ w621] -> w609
          frame False {
            w618 = T28."Enabled" ("Disabled")
            n298 = property on="Calibrating" class="Bool (strict)"("Blinking"=FALSE) -> ()  [unwired: 2 in, 2 out]
            n299 = property on="ALT SET" class="Clust (strict)"("DisabledEnum"=w618) -> ()  [unwired: 2 in, 2 out]
            n300 = property on="Mode" class="VertMode (strict)"("DisabledEnum"=w618) -> ()  [unwired: 2 in, 2 out]
            n301 = property on="ALT SET 2" class="Clust (strict)"("DisabledEnum"=w618) -> ()  [unwired: 2 in, 2 out]
            n302 = property on="Mode 1" class="VertMode (strict)"("DisabledEnum"=w618) -> ()  [unwired: 2 in, 2 out]
          }
          frame True {
            # "Don't issue read command if we are done"
            n303 = VISA Write(VISA resource name=w623, write buffer="R") -> (VISA resource name out=w622:refnum<visa-resource-name>, error out=w621:errorcluster)  [unwired: 1 in, 1 out]
          }
        }
      }
      frame "Idle", Default {
        w658 = FALSE ("Time has Elapsed")
        n304 = Enqueue Element(queue=w655, element="Check Timer" ("f")) -> (queue out=w638:refnum<queue>)  [unwired: 2 in, 2 out]
        n305 = local read "Set Point Alt"() -> (w648:i32)
        n306 = local read "ALT SET"() -> (w656:T8)
        n307 = To Long Integer(number=w648) -> (32bit integer=w657:i32)
        n308 = feedback #7(w657) -> (w659:i32)
        n309 = feedback #8(w656) -> (w664:T8)
        n310 = feedback #9(w658) -> (w667:bool)
        n311 = feedback #10(w658) -> (w666:bool)
        n312 = event shown="[19] \"reset\": Value Change" {
          selector: _ -> [_ _ _ _ _ _ _ _ _ _ _ _ _ _ _ _ _ _ _ _ _ _ _ _ _ _]
          dyn-events: _ -> [_ _ _ _ _ _ _ _ _ _ _ _ _ _ _ _ _ _ _ _ _ _ _ _ _ _]
          timeout: 10 -> [_ _ _ _ _ _ _ _ _ _ _ _ _ _ _ _ _ _ _ _ _ _ _ _ _ _]
          tunnel: w663 -> [_ _ _ _ _ _ _ _ w901 _ _ _ _ w970 _ _ _ _ _ _ _ _ _ _ _ _]
          tunnel: [w704 w728 w742 w770 w785 w812 w870 w892 w905 w922 w937 w948 w959 w977 w987 w999 w1012 w1018 TRUE ("Time has Elapsed") w1055 w1062 w1081 w1089 w1101 w1115 w1128] -> w669
          tunnel: w666 -> [w703 w728 w742 w770 w785 w812 w870 w892 w905 w922 w937 w948 w959 w977 w987 w999 w1012 _ _ w1055 w1062 w1081 w1089 w1101 w1115 w1128]
          tunnel: [w701 w729 w743 w768 w786 w811 w871 w893 w903 w923 w938 w949 w960 w976 w988 w1000 w1009 w1027 "ALT SET" w1056 w1061 w1082 w1090 w1102 w1116 w1129] -> w665
          tunnel: w664 -> [w702 w729 w743 w768 w786 w811 w871 w893 w903 w923 w938 w949 w960 w976 w988 w1000 w1009 w1027 _ w1056 w1061 w1082 w1090 w1102 w1116 w1129]
          tunnel: w667 -> [w693 w727 w741 w769 w784 w810 w869 w891 w904 w921 w936 w947 w958 w978 w986 w998 w1011 _ _ w1054 w1063 w1080 w1088 w1100 w1114 w1127]
          tunnel: [w700 w727 w741 w769 w784 w810 w869 w891 w904 w921 w936 w947 w958 w978 w986 w998 w1011 w1018 w1035 w1054 w1063 w1080 w1088 w1100 w1114 w1127] -> w668
          tunnel: [w697 w726 w740 w767 w783 w797 w872 w890 w902 w920 w933 w944 w955 w975 w985 w997 w1010 w1028 w1039 w1053 w1060 w1079 w1091 w1103 w1117 w1130] -> w660
          tunnel: w659 -> [w697 w726 w740 w767 w783 _ w872 w890 w902 w920 w934 w944 w955 w975 w985 w997 w1010 w1028 _ w1053 w1060 w1079 w1091 w1103 w1117 w1130]
          tunnel: w638 -> [_ _ _ _ _ _ _ _ _ _ _ _ _ _ _ _ _ _ _ w1052 w1059 w1078 _ _ _ _]
          tunnel: [w696 w724 w738 w761 w787 w809 w868 w888 FALSE w918 w932 w946 w957 w974 w983 w995 w1013 w1026 w1038 w1051 w1064 w1077 w1087 w1099 w1113 w1126] -> w651
          tunnel: w652 -> [w696 w724 w738 w761 w787 w809 w868 w888 _ w918 w932 w946 w957 w974 w983 w995 w1013 w1026 w1038 w1051 w1064 w1077 w1087 w1099 w1113 w1126]
          tunnel: w650 -> [w695 w725 w739 w760 w782 w807 w873 w889 w898 w919 w930 w945 w956 w973 w984 w996 w1008 w1020 w1037 w1050 w1067 w1076 w1092 w1104 w1118 w1131]
          tunnel: [w695 w725 w739 w760 w781 w807 w873 w889 w898 w919 w930 w945 w956 w973 w984 w996 w1008 w1020 w1037 w1050 w1067 w1076 w1092 w1104 w1118 w1131] -> w649
          tunnel: w647 -> [w694 w722 w737 w758 w779 w806 w867 w883 w897 w914 w927 w942 w953 w965 w982 _ w1005 w1019 w1036 w1049 w1065 w1073 w1086 w1098 w1112 w1125]
          tunnel: [w694 w722 w737 w758 w779 w806 w867 w883 w897 w914 w927 w942 w953 w965 w982 w992 w1005 w1019 w1036 w1049 w1065 w1073 w1086 w1098 w1112 w1125] -> w646
          tunnel: w645 -> [w692 w721 w736 w757 w778 w796 w866 w882 w896 w913 w926 w941 w952 w964 w981 w991 w1004 w1017 w1034 w1048 w1066 w1072 w1085 w1097 w1111 w1124]
          tunnel: [w692 w721 w732 w757 w778 w796 w866 w882 w896 w913 w926 w941 w952 w964 w981 w991 w1004 w1017 w1034 w1048 w1066 w1072 w1085 w1097 w1111 w1124] -> w644
          tunnel: w643 -> [w691 w720 w731 w756 w777 w795 w864 w881 w895 w912 w925 w940 w951 w963 w980 w990 w1003 w1015 w1033 w1047 w1069 w1071 w1094 w1105 w1110 w1136]
          tunnel: [w691 w720 w731 w756 w777 w790 w864 w881 w895 w912 w925 w940 w951 w963 w980 w990 w1003 w1015 w1033 w1047 w1069 w1071 w1093 w1105 w1110 w1133] -> w642
          tunnel: w641 -> [w675 _ _ _ _ _ _ _ _ _ _ _ _ _ _ _ _ _ _ _ _ _ _ _ _ _]
          tunnel: w640 -> [w673 w719 w730 w755 w776 w789 w863 w880 w894 w911 w924 w939 w950 w962 w979 w989 w1002 w1014 w1030 w1046 w1068 w1070 w1084 w1108 w1122 w1132]
          tunnel: [w673 w719 w730 w755 w776 w789 w863 w880 w894 w911 w924 w939 w950 w962 w979 w989 w1002 w1014 w1030 w1046 w1068 w1070 w1084 w1106 w1119 w1132] -> w639
          tunnel: [_ _ _ _ _ TRUE _ TRUE _ TRUE _ _ _ TRUE _ _ TRUE _ TRUE _ _ _ TRUE TRUE TRUE TRUE] -> w637
          event Timeout {
            n313 = event-data() -> ()  [unwired: 1 in, 1 out]
            n314 = case shown="False" w693 {
              selector: w693 -> [w708 _]
              tunnel: [w707 w710] -> w704
              tunnel: w703 -> [w707 w715]
              tunnel: w702 -> [w709 w713]
              tunnel: [w709 w712] -> w701
              tunnel: [w708 w711] -> w700
              frame False {
              }
              frame True {
                n315 = call "Elapsed Time"("Time Target (s)"=10.0, "Reset"=w715) -> ("Time has Elapsed"=w710:bool)  [unwired: 10 in, 7 out]
                n316 = Not(x=w710) -> (.not. x?=w711:bool)
                n317 = case shown="True" w710 {
                  tunnel: w713 -> [w716 w718]
                  tunnel: [w716 w718] -> w712
                  frame False {
                  }
                  frame True {
                    w717 = FALSE ("Visible")
                    n318 = local write "ALT SET 2"(w718) -> ()
                    n319 = local write "ALT SET"(w718) -> ()
                    n320 = property on="Confirm Now 2" class="Bool (strict)"("Visible"=w717) -> ()  [unwired: 2 in, 2 out]
                    n321 = property on="Confirm Now" class="Bool (strict)"("Visible"=w717) -> ()  [unwired: 2 in, 2 out]
                  }
                }
              }
            }
            n322 = case "Set Color" shown="False" w693 {
              tunnel: [cluster{u32, u32}[] [{13816530, 13816530}, {13816530, 13816530}] ("Colors [4] 2") cluster{u32, u32}[] [{16711700, 16711700}, {13816530, 13816530}] ("Colors [4]")] -> w699
              frame False {
              }
              frame True {
              }
            }
            n323 = property on="Confirm Now 2" class="Bool (strict)"("Colors [4]"=w699) -> ()  [unwired: 2 in, 2 out]
            n324 = property on="Confirm Now" class="Bool (strict)"("Colors [4]"=w699) -> ()  [unwired: 2 in, 2 out]
            n325 = call "Retrieve WMI String.vi"("wmiProperty"="VideoOutputTechnology", "wmiClass"="WmiMonitorConnectionParams", "Scope"="root\\WMI") -> ("Values"=w687:string[])  [unwired: 6 in, 2 out]
            n326 = Array Size(array=w687) -> (size(s)=w686:i32)
            n327 = local read "Altitude"() -> (w676:sgl)
            n328 = Greater?(x=w686, y=1) -> (0:w678:bool)
            n329 = property on="Setup Tables Visible" class="Bool (strict)"() -> ("Value"=w698:bool)  [unwired: 2 in, 2 out]
            n330 = property on="Main Tabs" class="TabCtl (strict)"("Visible"=w698) -> ()  [unwired: 2 in, 2 out]
            n331 = property on="ALT Window ON/OFF" class="Bool (strict)"("Visible"=w678) -> ("Value"=w679:bool)  [unwired: 2 in, 2 out]
            n332 = And(x=w679, y=w678) -> (x .and. y?=w677:bool)
            n333 = property on="Feet OFF/ Meters ON" class="Bool (strict)"() -> ("Value"=w674:bool)  [unwired: 2 in, 2 out]
            n334 = Select(t="Current Effective Altitude in Meters" ("Heading"), s=w674, f="Current Effective Altitude in Feet" ("Heading")) -> (s? t:f=w681:string)
            n335 = Bundle(cluster=T21 {"Heading"="Current Effective Altitude in  Feet", "Altitude"=0.0, "Visible?"=TRUE}, "Heading"=w681, "Altitude"=w676, "Visible?"=w677) -> (w680:T21)
            n336 = Send Notification(notification=w680, notifier=w675) -> ()  [unwired: 1 in, 2 out]
          }
          event "Close": Value Change {
            n337 = event-data() -> ()  [unwired: 1 in, 1 out]
            n338 = property on="Setup Tables Visible" class="Bool (strict)"("Value"=FALSE) -> ()  [unwired: 2 in, 2 out]
          }
          event "eCode": Value Change {
            n339 = event-data() -> ()  [unwired: 1 in, 1 out]
            n340 = flat-sequence {
              tunnel: w736 -> [w749]
              tunnel: [w748] -> w732
              tunnel: [w745] -> _
              frame #0 {
                n341 = One Button Dialog(message="Enter valid code to continue operation.\nCall CAT for new code.") -> ()  [unwired: 1 in, 1 out]
              }
              frame #1 {
                n342 = Build Path(base path=path "C:/temp" ("path"), name or relative path="cat_panel.tmp") -> (appended path=w753:path)
                n343 = call <vilib>:"Open Config Data.vi"("configuration file path"=w753) -> ("error out"=w750:errorcluster, "refnum"=w751:T27)  [unwired: 8 in, 1 out]
                n344 = call "Get Key.vi"("error in"=w750, "Sorted Data in"=w749, "Refnum in"=w751) -> ("error out"=w747:errorcluster, "Cancel?"=w745:bool, "Sorted Data out"=w748:T32, "Refnum out"=w746:T27)  [unwired: 5 in]
                n345 = call <vilib>:"Close Config Data.vi"("error in (no error)"=w747, "refnum"=w746) -> ()  [unwired: 8 in, 2 out]
              }
            }
            n346 = Unbundle By Name(w732) -> ("Key Valid?"=w735:bool[])
            n347 = Index Array(array=w735) -> (element=w734:bool)  [unwired: 1 in]
            n348 = Not(x=w734) -> (.not. x?=w733:bool)
            n349 = property on="eCode" class="Bool"("Visible"=w733) -> ()  [unwired: 2 in, 2 out]
          }
          event "Enter or Exit Setup": Value Change {
            n350 = event-data() -> ()  [unwired: 1 in, 1 out]
            n351 = control-ref of="Level 0"() -> (w763:refnum<vi>)
            n352 = control-ref of="Level 1"() -> (w764:refnum<vi>)
            n353 = control-ref of="Level 2"() -> (w765:refnum<vi>)
            n354 = control-ref of="Level 3"() -> (w766:refnum<vi>)
            n355 = Build Array(w763, w764, w765, w766) -> (w762:refnum<vi>[])
            n356 = call "Access Levels.vi"("Action"=enum8{"Set Codes", "Get Level"}."Get Level") -> ("Level"=w771:u8)  [unwired: 4 in]
            n357 = for {
              tunnel: w762 -> [w773] mode=indexing
              tunnel: w771 -> [w775]
              i -> [w774]
              n358 = Less Or Equal?(x=w774, y=w775) -> (x <= y?=w772:bool)
              n359 = property class="Clust"(reference=w773, "Visible"=w772) -> ()  [unwired: 1 in, 2 out]
            }
          }
          event "writetofile": Value Change {
            n360 = event-data() -> ("NewVal"=w780:bool)  [unwired: 1 in]
            n361 = call-dynamic "Write Write.vi"("Write?"=w780, "File in"=w782) -> ("File out"=w781:refnum<class "File.lvclass">)  [unwired: 8 in, 1 out]
          }
          event "Level 1.Feet OFF/ Meters ON": Value Change {
            n362 = event-data() -> ("NewVal"=w802:bool)  [unwired: 1 in]
            n363 = property on="Max Altitude" class="DigNum (strict)"() -> ("Value"=w800:dbl)  [unwired: 2 in, 2 out]
            n364 = local read "Level 3"() -> (w805:T19)
            n365 = local read "Set Point Alt"() -> (w804:i32)
            n366 = property on="maxAltSP" class="DigNum (strict)"() -> ("Value"=w803:sgl)  [unwired: 2 in, 2 out]
            n367 = Index Array(array=w795) -> (element #1=w793:T6, element #2=w794:T6)  [unwired: 2 in]
            n368 = in-place {
              in-place-border: w802 -> [w838]
              n369 = in-place-cluster #11(w793) -> ("Set Point Force"=w824:T4, "Run A1"=w823:T4, "Run A2"=w822:T4, "Hold A3"=w821:T4, "Hold A4"=w820:T4)
              n370 = in-place-cluster #12(w794) -> ("Set Point Force"=w848:T4, "Run A1"=w847:T4, "Run A2"=w846:T4, "Hold A3"=w845:T4, "Hold A4"=w844:T4)
              n371 = in-place-cluster #13(w805) -> ("Alarm Points.AltLim"=w843:sgl)
              n372 = in-place-match #14(w804) -> (w842:i32)
              n373 = in-place-match #15(w803) -> (w841:sgl)
              n374 = in-place-match #16(w800) -> (w837:dbl)
              n375 = Bundle("Set Point Force"=w824, "Run A1"=w823, "Run A2"=w822, "Hold A3"=w821, "Hold A4"=w820) -> (w819:T40)  [unwired: 1 in]
              n376 = Bundle("Set Point Force"=w848, "Run A1"=w847, "Run A2"=w846, "Hold A3"=w845, "Hold A4"=w844, "AltLim"=w843, "Set Point Alt"=w842, "Value"=w841, "Value"=w837) -> (w840:T41)  [unwired: 1 in]
              n377 = case shown="False" w838 {
                tunnel: w840 -> [w853 w860]
                tunnel: [w852 w859] -> w839
                tunnel: ["Current Effective Altitude in Feet" ("Heading") "Current Effective Altitude in Meters" ("Heading")] -> w826
                tunnel: ["F\ne\ne\nt" ("Units") "M\ne\nt\ne\nr\ns" ("Units")] -> w836
                tunnel: 0.3048 -> [w850 w857]
                tunnel: w819 -> [w851 w858]
                tunnel: [w849 w856] -> w818
                frame False {
                  n378 = Divide(x=w853, y=w850) -> (x/y=w852:T42)
                  n379 = Divide(x=w851, y=w850) -> (x/y=w849:T40)
                }
                frame True {
                  n380 = Multiply(x=w858, y=w857) -> (x*y=w856:T40)
                  n381 = Multiply(x=w860, y=w857) -> (x*y=w859:T42)
                }
              }
              "Units" <- w836
              "Heading 2" <- w826
              "Heading 3" <- w826
              n382 = Unbundle(w839) -> ("Set Point Force"=w834:T4, "Run A1"=w833:T4, "Run A2"=w832:T4, "Hold A3"=w831:T4, "Hold A4"=w830:T4, "AltLim"=w829:dbl, "Set Point Alt"=w835:dbl, "Value"=w828:dbl, "Value"=w827:dbl)
              n383 = Unbundle(w818) -> ("Set Point Force"=w817:T4, "Run A1"=w816:T4, "Run A2"=w815:T4, "Hold A3"=w814:T4, "Hold A4"=w813:T4)
              n384 = in-place-cluster #11("Set Point Force"=w817, "Run A1"=w816, "Run A2"=w815, "Hold A3"=w814, "Hold A4"=w813) -> (w792:T6)
              n385 = in-place-cluster #12("Set Point Force"=w834, "Run A1"=w833, "Run A2"=w832, "Hold A3"=w831, "Hold A4"=w830) -> (w791:T6)
              n386 = in-place-cluster #13("Alarm Points.AltLim"=w829) -> (w801:T19)
              n387 = in-place-match #14(w835) -> (w797:i32)
              n388 = in-place-match #15(w828) -> (w799:sgl)
              n389 = in-place-match #16(w827) -> (w798:dbl)
            }
            n390 = property on="Max Altitude" class="DigNum (strict)"("Value"=w798) -> ()  [unwired: 2 in, 2 out]
            n391 = property on="maxAltSP" class="DigNum (strict)"("Value"=w799) -> ()  [unwired: 2 in, 2 out]
            n392 = local write "Level 3"(w801) -> ()
            n393 = Build Array(w792, w791) -> (w790:T6[])
            n394 = call "Convert Dbl to ALtitude.vi"("Setpoint"=w797) -> ("Altitude Out"=w808:T29)  [unwired: 10 in]
            n395 = local write "ALT SET 2"(w808) -> ()
            n396 = local write "ALT SET"(w808) -> ()
          }
          event "Level 0.Demo Mode?": Value Change {
            n397 = event-data() -> ("NewVal"=w865:bool)  [unwired: 1 in]
            n398 = case shown="True" w865 {
              frame False {
                w874 = T28."Enabled" ("Disabled")
                n399 = property on="Mode" class="VertMode (strict)"("DisabledEnum"=w874) -> ()  [unwired: 2 in, 2 out]
                n400 = property on="Mode 1" class="VertMode (strict)"("DisabledEnum"=w874) -> ()  [unwired: 2 in, 2 out]
              }
              frame True {
                w875 = FALSE ("sysStat")
                w878 = enum8{"Off", "Stby", "Hold", "Run"}."Off" ("Value (Signaling)")
                w877 = T28."Disabled and Grayed Out" ("Disabled")
                n401 = local write "senseConn"(FALSE ("senseConn")) -> ()
                n402 = property on="sysStat" class="Bool (strict)"("Value"=w875, "Blinking"=w875) -> ()  [unwired: 2 in, 2 out]
                n403 = property on="Mode" class="VertMode (strict)"("Val(Sgnl)"=w878, "DisabledEnum"=w877) -> ()  [unwired: 2 in, 2 out]
                n404 = property on="Mode 1" class="VertMode (strict)"("Val(Sgnl)"=w878, "DisabledEnum"=w877) -> ()  [unwired: 2 in, 2 out]
              }
            }
          }
          event "Level 2.Max Altitude": Value Change {
            # "Make sure the user setpoint max does not exceed the CAT defined setpoint max"
            n405 = event-data() -> ("NewVal"=w887:dbl)  [unwired: 1 in]
            n406 = property on="maxAltSP" class="DigNum (strict)"() -> ("Value"=w886:sgl)  [unwired: 2 in, 2 out]
            n407 = In Range and Coerce(upper limit=w886, x=w887, lower limit=0.0) -> (coerced(x)=w884:dbl)  [unwired: 1 out]
            n408 = property on="Max Altitude" class="DigNum (strict)"("Value"=w884) -> ()  [unwired: 2 in, 2 out]
          }
          event "Level 2.Enter Calibration": Value Change {
            # "Reset the Calibration boolean - this will prevent a read on the first case"
            n409 = event-data() -> ()  [unwired: 1 in, 1 out]
            n410 = local read "Mode"() -> (w900:enum8{"Off", "Stby", "Hold", "Run"})
            n411 = case shown="\"Stby\", Default" w900 {
              tunnel: w901 -> [_ w909]
              frame "Off" {
              }
              frame "Stby", Default {
                w906 = TRUE ("Blinking")
                w907 = T28."Disabled and Grayed Out" ("Disabled")
                n412 = VISA Write(VISA resource name=w909, write buffer="C") -> ()  [unwired: 1 in, 3 out]
                n413 = property on="Calibrating" class="Bool (strict)"("Value"=w906, "Blinking"=w906) -> ()  [unwired: 2 in, 2 out]
                n414 = property on="Mode 1" class="VertMode (strict)"("DisabledEnum"=w907) -> ()  [unwired: 2 in, 2 out]
                n415 = property on="Mode" class="VertMode (strict)"("DisabledEnum"=w907) -> ()  [unwired: 2 in, 2 out]
                n416 = property on="ALT SET" class="Clust (strict)"("DisabledEnum"=w907) -> ()  [unwired: 2 in, 2 out]
                n417 = property on="ALT SET 2" class="Clust (strict)"("DisabledEnum"=w907) -> ()  [unwired: 2 in, 2 out]
              }
            }
          }
          event Value Change {
            n418 = event-data() -> ("NewVal"=w917:T18)  [unwired: 1 in]
            n419 = local read "Final  Output Names"() -> (w916:T11)
            n420 = call "Populate Names.vi"("Final  Output In"=w916, "Final Names"=w917) -> ("Final  Output Out"=w915:T11)  [unwired: 9 in]
            n421 = local write "Final  Output Names"(w915) -> ()
          }
          event "Level 3.maxAltSP": Value Change {
            n422 = event-data() -> ("NewVal"=w929:sgl)  [unwired: 1 in]
            n423 = In Range and Coerce(upper limit=w929, x=w934, lower limit=0.0) -> (coerced(x)=w928:dbl)  [unwired: 1 out]
            n424 = call "Convert Dbl to ALtitude.vi"("Setpoint"=w928) -> ("Altitude Out"=w931:T29)  [unwired: 10 in]
            n425 = local write "ALT SET 2"(w931) -> ()
            n426 = local write "ALT SET"(w931) -> ()
            n427 = To Long Integer(number=w928) -> (32bit integer=w933:i32)
          }
          event "Level 2.Alt Points": Value Change {
            n428 = event-data() -> ("NewVal"=w943:u32)  [unwired: 1 in]
            n429 = property on="pAltitude" class="Multivalue Buffer (strict)"("History"=w943) -> ()  [unwired: 2 in, 2 out]
          }
          event "Level 2.CO2 Points": Value Change {
            n430 = event-data() -> ("NewVal"=w954:u32)  [unwired: 1 in]
            n431 = property on="CO2Buffer" class="Multivalue Buffer (strict)"("History"=w954) -> ()  [unwired: 2 in, 2 out]
          }
          event "Mode 1", "Mode": Value Change {
            n432 = event-data() -> ("NewVal"=w972:enum8{"Off", "Stby", "Hold", "Run"})  [unwired: 1 in]
            n433 = local write "Mode"(w972) -> ()
            n434 = local write "Mode 1"(w972) -> ()
            n435 = Not Equal To 0?(x=w972) -> (x != 0?=w966:bool)
            n436 = call "Call Power On-Off.vi"("Warmup if ON"=FALSE, "VISA Ref In"=w970, "On/Off"=w966) -> ()  [unwired: 2 in, 2 out]
            n437 = feedback-in #17(w966) -> ()
            n438 = feedback #17(FALSE) -> (w968:bool)
            n439 = Not Equal?(x=w966, y=w968) -> (x != y?=w967:bool)
            n440 = And(x=w967, y=w966) -> ()  [unwired: 1 out]
          }
          event "Level 3.Alarm Points.CalLimit", "Level 3.Alarm Points.SenseLimit", "Level 3.Alarm Points.CO2Lim", "Level 3.Alarm Points.AltLim", "Level 3.Alarm Points.O2 Low": Value Change {
            n441 = event-data() -> ()  [unwired: 1 in, 1 out]
          }
          event "Level 0.Time Offset (h)": Value Change {
            n442 = event-data() -> ("NewVal"=w994:dbl)  [unwired: 1 in]
            n443 = Multiply(x=w994, y=3600.0) -> (x*y=w992:dbl)
          }
          event "dimmer": Value Change {
            n444 = event-data() -> ()  [unwired: 1 in, 1 out]
            n445 = call "Dimmer FG.vi"("Operation"=enum16{"Init", "Run", "Close Ref"}."Run", "dimmer"="dimmer") -> ()  [unwired: 9 in, 1 out]
          }
          event Value Change {
            w1018 = TRUE
            n446 = event-data() -> ("NewVal"=w1025:T8)  [unwired: 1 in]
            n447 = local read "minAlt"() -> (w1016:dbl)
            n448 = call "Alt 2 Num.vi"("Alt Ctl"=w1025) -> ("Alt"=w1024:i32)  [unwired: 2 in]
            n449 = property on="Max Altitude" class="DigNum (strict)"() -> ("Value"=w1023:dbl)  [unwired: 2 in, 2 out]
            n450 = In Range and Coerce(upper limit=w1023, x=w1024, lower limit=w1016) -> (coerced(x)=w1022:dbl)  [unwired: 1 out]
            n451 = call "Convert Dbl to ALtitude.vi"("Setpoint"=w1022) -> ("Altitude Out"=w1021:T29)  [unwired: 10 in]
            n452 = local write "ALT SET"(w1021) -> ()
            n453 = local write "ALT SET 2"(w1021) -> ()
            n454 = property on="Confirm Now" class="Bool (strict)"("Visible"=w1018) -> ()  [unwired: 2 in, 2 out]
            n455 = property on="Confirm Now 2" class="Bool (strict)"("Visible"=w1018) -> ()  [unwired: 2 in, 2 out]
          }
          event "Confirm Now", "Confirm Now 2": Value Change {
            w1035 = FALSE
            n456 = event-data() -> ()  [unwired: 1 in, 1 out]
            n457 = local read "minAlt"() -> (w1032:dbl)
            n458 = local write "ALT SET 2"("ALT SET") -> ()
            n459 = property on="Max Altitude" class="DigNum (strict)"() -> ("Value"=w1042:dbl)  [unwired: 2 in, 2 out]
            n460 = call "Alt 2 Num.vi"("Alt Ctl"="ALT SET") -> ("Alt"=w1041:i32)  [unwired: 2 in]
            n461 = In Range and Coerce(upper limit=w1042, x=w1041, lower limit=w1032) -> (coerced(x)=w1031:dbl)  [unwired: 1 out]
            "altSp" <- w1031
            n462 = To Long Integer(number=w1031) -> (32bit integer=w1039:i32)
            n463 = property on="Confirm Now 2" class="Bool (strict)"("Value"=w1035, "Visible"=w1035) -> ()  [unwired: 2 in, 2 out]
            n464 = property on="Confirm Now" class="Bool (strict)"("Value"=w1035, "Visible"=w1035) -> ()  [unwired: 2 in, 2 out]
          }
          event "reset": Value Change {
            n465 = event-data() -> ()  [unwired: 1 in, 1 out]
            n466 = Flush Queue(queue=w1052) -> (queue out=w1044:refnum<queue>)  [unwired: 1 in, 2 out]
            n467 = Enqueue Element(queue=w1044, element="Stop") -> ()  [unwired: 2 in, 3 out]
          }
          event "Shutdown": Value Change {
            n468 = event-data() -> ()  [unwired: 1 in, 1 out]
            n469 = Flush Queue(queue=w1059) -> (queue out=w1057:refnum<queue>)  [unwired: 1 in, 2 out]
            n470 = Enqueue Element(queue=w1057, element="Stop") -> ()  [unwired: 2 in, 3 out]
          }
          event "Level 3.Stop": Value Change {
            n471 = event-data() -> ()  [unwired: 1 in, 1 out]
            n472 = Flush Queue(queue=w1078) -> (queue out=w1074:refnum<queue>)  [unwired: 1 in, 2 out]
            n473 = Enqueue Element(queue=w1074, element="Stop") -> ()  [unwired: 2 in, 3 out]
          }
          event Value Change {
            n474 = event-data() -> ("NewVal"=w1095:T6)  [unwired: 1 in]
            n475 = Replace Array Subset(array=w1094, new element=w1095) -> (w1093:T6[])  [unwired: 1 in]
          }
          event Value Change {
            n476 = event-data() -> ("NewVal"=w1107:T3)  [unwired: 1 in]
            n477 = Replace Array Subset(array=w1108, new element=w1107) -> (w1106:T3[])  [unwired: 1 in]
          }
          event Value Change {
            n478 = event-data() -> ("NewVal"=w1120:T3)  [unwired: 1 in]
            n479 = Replace Array Subset(array=w1122, new element=w1120, index=1) -> (w1119:T3[])
          }
          event Value Change {
            n480 = event-data() -> ("NewVal"=w1135:T6)  [unwired: 1 in]
            n481 = Replace Array Subset(array=w1136, new element=w1135, index=1) -> (w1133:T6[])
          }
        }
        n482 = feedback-in #7(w660) -> ()
        n483 = feedback-in #8(w665) -> ()
        n484 = feedback-in #9(w668) -> ()
        n485 = feedback-in #10(w669) -> ()
        n486 = local write "Set Point Alt"(w660) -> ()
        n487 = case shown="True" w637 {
          tunnel: w638 -> [_ w672]
          frame False {
          }
          frame True {
            n488 = Enqueue Element(queue=w672, element="Write to Config FIle") -> ()  [unwired: 2 in, 3 out]
          }
        }
      }
      frame "Check Timer" {
        # "Attempt to contact the controller every 6 s +/- 10 ms"
        n489 = feedback #18(0.0 ("Set Start Time (s)")) -> (w1154:dbl)
        n490 = feedback #19(TRUE ("Time has Elapsed")) -> (w1166:bool)
        n491 = call "Elapsed Time2"("Time Target (s)"=6.0, "Reset"=w1166, "Auto Reset"=FALSE, "Set Start Time (s)"=w1154) -> ("Present (s)"=w1170:dbl, "Time has Elapsed"=w1149:bool)  [unwired: 8 in, 6 out]
        n492 = feedback-in #19(w1149) -> ()
        n493 = Select(t=w1170, s=w1149, f=w1154) -> (s? t:f=w1169:dbl)
        n494 = feedback-in #18(w1169) -> ()
        n495 = local read "Calibrating"() -> (w1160:bool)
        n496 = Select(t="Controller: Calibrate", s=w1160, f="Controller: Update Mode") -> (s? t:f=w1152:string)
        n497 = local read "senseConn"() -> (w1142:bool)
        n498 = Select(t="Controller: Comm Error", s=w1142, f=w1152) -> (s? t:f=w1148:string)
        n499 = feedback #20() -> (w1143:enum8{"Off", "Stby", "Hold", "Run"})  [unwired: 1 in]
        n500 = case shown="False" w1149 {
          tunnel: ["Idle" ("f") w1211] -> w1147
          tunnel: w1148 -> [_ w1211]
          tunnel: w1146 -> [w1173 w1210]
          tunnel: [w1172 w1202] -> w1145
          tunnel: [w1171 w1209] -> w1144
          tunnel: w1143 -> [w1171 w1208]
          tunnel: w1142 -> [_ w1204]
          frame False {
            n501 = local read "codelapse"() -> (w1174:bool)
            n502 = case shown="True" w1174 {
              tunnel: w1173 -> [w1176 w1181]
              tunnel: [w1176 w1180] -> w1172
              tunnel: w1171 -> [_ w1178]
              frame False {
              }
              frame True {
                n503 = flat-sequence {
                  tunnel: w1181 -> [w1190]
                  tunnel: [w1189] -> w1180
                  tunnel: [w1186] -> w1179
                  frame #0 {
                    n504 = One Button Dialog(message="Enter valid code to continue operation.\nCall CAT for new code.") -> ()  [unwired: 1 in, 1 out]
                  }
                  frame #1 {
                    n505 = Build Path(base path=path "C:/temp" ("path"), name or relative path="cat_panel.tmp") -> (appended path=w1194:path)
                    n506 = call <vilib>:"Open Config Data.vi"("configuration file path"=w1194) -> ("error out"=w1191:errorcluster, "refnum"=w1192:T27)  [unwired: 8 in, 1 out]
                    n507 = call "Get Key.vi"("error in"=w1191, "Sorted Data in"=w1190, "Refnum in"=w1192) -> ("error out"=w1188:errorcluster, "Cancel?"=w1186:bool, "Sorted Data out"=w1189:T32, "Refnum out"=w1187:T27)  [unwired: 5 in]
                    n508 = call <vilib>:"Close Config Data.vi"("error in (no error)"=w1188, "refnum"=w1187) -> ()  [unwired: 8 in, 2 out]
                  }
                }
                n509 = local write "codelapse"(FALSE ("codelapse")) -> ()
                n510 = case shown="False" w1179 {
                  tunnel: w1178 -> [w1182 _]
                  frame False {
                    # "CODE GOOD - RESET STATE TO PREVIOUS MODE"
                    n511 = local write "codelapse"(FALSE ("codelapse")) -> ()
                    n512 = property on="Mode" class="VertMode (strict)"("Val(Sgnl)"=w1182) -> ()  [unwired: 2 in, 2 out]
                  }
                  frame True {
                    # "DO NOTHING IF CODE NOT GOOD - REMAIN OFF"
                    n513 = One Button Dialog(message="Controller not accessible - no valid code avaialble.  Please contact CAT to obtain a valid code. ") -> ()  [unwired: 1 in, 1 out]
                  }
                }
              }
            }
          }
          frame True {
            # "TIME ELAPSED"
            n514 = local read "Mode"() -> (w1207:enum8{"Off", "Stby", "Hold", "Run"})
            n515 = local read "Time"() -> (w1200:timestamp)
            n516 = Not Equal?(x=w1207, y=enum8{"Off", "Stby", "Hold", "Run"}."Off") -> (x != y?=w1205:bool)
            n517 = Not(x=w1204) -> (.not. x?=w1203:bool)
            n518 = And(x=w1205, y=w1203) -> (x .and. y?=w1201:bool)
            n519 = Not Equal To 0?(x=w1200) -> (x != 0?=w1199:bool)
            n520 = And(x=w1201, y=w1199) -> (x .and. y?=w1198:bool)
            n521 = case shown="True" w1198 {
              tunnel: w1210 -> [w1212 w1219]
              tunnel: [w1213 w1218] -> w1209
              tunnel: w1208 -> [w1213 w1216]
              tunnel: [w1212 w1214] -> w1202
              frame False {
                # "Sensor is unconnected or the mode is off."
              }
              frame True {
                n522 = local read "Time"() -> (w1215:timestamp)
                n523 = call "Check Keys.vi"("Time"=w1215, "Sorted Data in"=w1219) -> ("codelapse"=w1217:bool, "Sorted Data Out"=w1214:T32)  [unwired: 8 in]
                "codelapse" <- w1217
                n524 = case shown="True" w1217 {
                  tunnel: [w1220 w1221] -> w1218
                  tunnel: w1216 -> [w1220 _]
                  frame False {
                  }
                  frame True {
                    # "CODE LAPSE"
                    n525 = property on="Mode" class="VertMode (strict)"("Val(Sgnl)"=enum8{"Off", "Stby", "Hold", "Run"}."Off" ("Value (Signaling)")) -> ("Value"=w1221:enum8{"Off", "Stby", "Hold", "Run"})  [unwired: 2 in, 2 out]
                  }
                }
              }
            }
            n526 = call "WMI Get Battery Status.vi"() -> ("Discharging?"=→"onBatt":bool, "estCharge"=→"estBattLeft":u8)  [unwired: 8 in, 2 out]
          }
        }
        n527 = feedback-in #20(w1144) -> ()
        n528 = Enqueue Element(queue=w1157, element=w1147) -> (queue out=w1139:refnum<queue>, error out=w1138:errorcluster)  [unwired: 2 in, 1 out]
        n529 = Preview Queue Element(queue=w1139, error in (no error)=w1138) -> (element=w1137:string)  [unwired: 1 in, 3 out]
      }
      frame "Stop" {
        w1242 = FALSE ("Leave CAT On/Off at Program Exit")
        # "Turn the controller off before exiting."
        n530 = Release Notifier(notifier=w1226, force destroy? (F)=TRUE) -> (error out=w1223:errorcluster)  [unwired: 1 in, 2 out]
        n531 = Close Reference(reference=w1224, error in (no error)=w1223) -> ()  [unwired: 1 out]
        n532 = Enqueue Element(queue=w1232, element="Write to Config FIle") -> ()  [unwired: 2 in, 3 out]
        n533 = call "Dimmer FG.vi"("Operation"=enum16{"Init", "Run", "Close Ref"}."Close Ref") -> ()  [unwired: 10 in, 1 out]
        n534 = call "Call Power On-Off.vi"("Warmup if ON"=w1242, "VISA Ref In"=w1239, "On/Off"=w1242) -> ("error out"=w1241:errorcluster, "VISA Ref Out"=w1240:refnum<visa-resource-name>)  [unwired: 2 in]
        n535 = VISA Close(VISA resource name=w1240, error in (no error)=w1241) -> (error out=w1238:errorcluster)
        n536 = call-dynamic "Close File.vi"("File in"=w1235) -> ("File out"=w1234:refnum<class "File.lvclass">)  [unwired: 9 in, 1 out]
      }
      frame "Write to Config FIle" {
        w1255 = "System" ("section")
        w1294 = "Altitude" ("section")
        n537 = Get Notifier Status(notifier=w1249) -> (error out=w1248:errorcluster)  [unwired: 1 in, 4 out]
        n538 = local read "Set Point Alt"() -> (w1310:i32)
        n539 = property on="West ON/Std OFF" class="Bool (strict)"() -> ("Value"=w1314:bool)  [unwired: 2 in, 2 out]
        n540 = Build Path(base path=path "C:/temp" ("path"), name or relative path="cat_panel.tmp") -> (appended path=w1319:path)
        n541 = case shown="Error" w1248 {
          tunnel: w1298 -> [_ w1348]
          tunnel: [FALSE TRUE] -> w1250
          frame No Error {
          }
          frame Error {
            n542 = Release Queue(queue=w1348) -> ()  [unwired: 2 in, 3 out]
          }
        }
        n543 = local read "Mode"() -> (w1315:enum8{"Off", "Stby", "Hold", "Run"})
        n544 = call <vilib>:"Open Config Data.vi"("configuration file path"=w1319) -> ("error out"=w1317:errorcluster, "refnum"=w1318:T27)  [unwired: 8 in, 1 out]
        n545 = property on="Feet OFF/ Meters ON" class="Bool (strict)"() -> ("Value"=w1313:bool)  [unwired: 2 in, 2 out]
        n546 = To Double Precision Float(number=w1310) -> (double precision float=w1309:dbl)
        n547 = call-poly <vilib>:"Write Key.vi"("section"="Mode", "error in (no error)"=w1317, "value"=w1315, "key"="mode?", "refnum"=w1318) -> ("error out"=w1325:errorcluster, "refnum out"=w1333:T27)  [unwired: 4 in, 1 out]
        n548 = call-poly <vilib>:"Write Key.vi"("section"=w1294, "error in (no error)"=w1325, "value"=w1309, "key"="Setpoint", "refnum"=w1333) -> ("error out"=w1324:errorcluster, "refnum out"=w1332:T27)  [unwired: 4 in, 1 out]
        n549 = property on="maxAltSP" class="DigNum (strict)"() -> ("Value"=w1312:sgl)  [unwired: 2 in, 2 out]
        n550 = call-poly <vilib>:"Write Key.vi"("section"=w1294, "error in (no error)"=w1324, "value"=w1314, "key"="West?", "refnum"=w1332) -> ("error out"=w1311:errorcluster, "refnum out"=w1323:T27)  [unwired: 4 in, 1 out]
        n551 = call-poly <vilib>:"Write Key.vi"("section"=w1294, "error in (no error)"=w1311, "value"=w1312, "key"="Max", "refnum"=w1323) -> ("error out"=w1321:errorcluster, "refnum out"=w1322:T27)  [unwired: 4 in, 1 out]
        n552 = call-poly <vilib>:"Write Key.vi"("section"=w1294, "error in (no error)"=w1321, "value"=w1313, "key"="Meters?", "refnum"=w1322) -> ("error out"=w1283:errorcluster, "refnum out"=w1292:T27)  [unwired: 4 in, 1 out]
        n553 = property on="Max Altitude" class="DigNum (strict)"() -> ("Value"=w1290:dbl)  [unwired: 2 in, 2 out]
        n554 = local read "Level 3"() -> (w1304:T19)
        n555 = property on="Time Offset (h)" class="DigNum (strict)"() -> ("Value"=w1285:dbl)  [unwired: 2 in, 2 out]
        n556 = call-poly <vilib>:"Write Key.vi"("section"=w1294, "error in (no error)"=w1283, "value"=w1290, "key"="custMax", "refnum"=w1292) -> ("error out"=w1282:errorcluster, "refnum out"=w1291:T27)  [unwired: 4 in, 1 out]
        n557 = Unbundle By Name(w1304) -> ("Alarm Points"=w1296:T43)
        n558 = property on="Final  Output Names" class="Clust (strict)"() -> ("Value"=w1306:T18)  [unwired: 2 in, 2 out]
        n559 = call <userlib>:"Write Section Cluster__ogtk.vi"("section (optional)"="Channel Names", "error in (no error)"=w1282, "Section Formatted Cluster"=w1306, "refnum"=w1291) -> ("error out"=w1287:errorcluster, "dup refnum"=w1288:T27)  [unwired: 6 in]
        n560 = local read "dimmer"() -> (w1258:i8)
        n561 = property on="ALT Window ON/OFF" class="Bool (strict)"() -> ("Value"=w1252:bool)  [unwired: 2 in, 2 out]
        n562 = call-poly <vilib>:"Write Key.vi"("section"=w1255, "error in (no error)"=w1287, "value"=w1285, "key"="dt", "refnum"=w1288) -> ("error out"=w1259:errorcluster, "refnum out"=w1261:T27)  [unwired: 4 in, 1 out]
        n563 = Index Array(array=w1281) -> (element #1=w1279:T6, element #2=w1274:T6)  [unwired: 2 in]
        n564 = call-poly <vilib>:"Write Key.vi"("section"=w1255, "error in (no error)"=w1259, "value"=w1258, "key"="dim" ("section"), "refnum"=w1261) -> ("error out"=w1256:errorcluster, "refnum out"=w1257:T27)  [unwired: 4 in, 1 out]
        n565 = local read "Other Outputs"() -> (w1305:cluster{"Alarm":bool, "Heater":bool})
        n566 = Current VI's Path() -> (path=w1301:path)
        n567 = call-poly <vilib>:"Write Key.vi"("section"=w1255, "error in (no error)"=w1256, "value"=w1252, "key"="altDisplay", "refnum"=w1257) -> ("error out"=w1253:errorcluster, "refnum out"=w1254:T27)  [unwired: 4 in, 1 out]
        n568 = call <userlib>:"Write Section Cluster__ogtk.vi"("section (optional)"="AD Settings", "error in (no error)"=w1253, "Section Formatted Cluster"=w1279, "refnum"=w1254) -> ("error out"=w1277:errorcluster, "dup refnum"=w1278:T27)  [unwired: 6 in]
        n569 = Strip Path(path=w1301) -> (stripped path=w1302:path)  [unwired: 1 out]
        n570 = call <userlib>:"Write Section Cluster__ogtk.vi"("section (optional)"="Hyperoxic AD Settings", "error in (no error)"=w1277, "Section Formatted Cluster"=w1274, "refnum"=w1278) -> ("error out"=w1275:errorcluster, "dup refnum"=w1276:T27)  [unwired: 6 in]
        n571 = disable-structure shown="RUN_TIME_ENGINE==True" {
          disable-tunnel: w1302 -> [w1350 w1351]
          disable-tunnel: [w1349 w1351] -> w1303
          frame condition #0 {
            n572 = Strip Path(path=w1350) -> (stripped path=w1349:path)  [unwired: 1 out]
          }
          frame condition #1 (active) {
          }
        }
        n573 = call <userlib>:"Write Section Cluster__ogtk.vi"("section (optional)"="Alarm Setpoints", "error in (no error)"=w1275, "Section Formatted Cluster"=w1296, "refnum"=w1276) -> ("error out"=w1307:errorcluster, "dup refnum"=w1308:T27)  [unwired: 6 in]
        n574 = call <userlib>:"Write Section Cluster__ogtk.vi"("error in (no error)"=w1307, "Section Formatted Cluster"=w1305, "refnum"=w1308) -> ("error out"=w1271:errorcluster, "dup refnum"=w1272:T27)  [unwired: 7 in]
        n575 = Build Path(base path=w1303, name or relative path="cat panel.cfg") -> (appended path=w1299:path)
        n576 = Index Array(array=w1270) -> (element #1=w1269:T3, element #2=w1264:T3)  [unwired: 2 in]
        n577 = call <userlib>:"Write Section Cluster__ogtk.vi"("section (optional)"="CO2 Settings", "error in (no error)"=w1271, "Section Formatted Cluster"=w1269, "refnum"=w1272) -> ("error out"=w1267:errorcluster, "dup refnum"=w1268:T27)  [unwired: 6 in]
        n578 = call <userlib>:"Write Section Cluster__ogtk.vi"("section (optional)"="Hyperoxic CO2 Settings", "error in (no error)"=w1267, "Section Formatted Cluster"=w1264, "refnum"=w1268) -> ("error out"=w1265:errorcluster, "dup refnum"=w1266:T27)  [unwired: 6 in]
        n579 = call <vilib>:"Close Config Data.vi"("error in (no error)"=w1265, "refnum"=w1266) -> ("error out"=w1338:errorcluster, "file path"=w1247:path)  [unwired: 8 in]
        n580 = Read from Text File(file (use dialog)=w1247, error in=w1338) -> (text=w1336:string, error out=w1246:errorcluster)  [unwired: 2 in, 2 out]
        n581 = call <userlib>:"Hill Cipher Encryption.vi"("Operation"=enum16{"Encrypt", "Decrypt", "Decrypt from Hex"}."Encrypt", "Input String"=w1336) -> ("Output String"=w1335:string)  [unwired: 7 in, 2 out]
        n582 = Write to Text File(file (use dialog)=w1299, text=w1335, error in=w1246) -> (error out=w1334:errorcluster)  [unwired: 1 in, 2 out]
        n583 = call <vilib>:"Simple Error Handler.vi"("error in (no error)"=w1334) -> ()  [unwired: 4 in, 5 out]
      }
    }
  }
  n584 = timed-loop {
    timing: w29 -> [_]
    timing-out: [_] -> w28
    tunnel: w18 -> [_]
    shift-right: [w1361] -> _
    shift-left: TRUE -> [w1357]
    shift-right: [w1358] -> _
    shift-left: FALSE ("Sensor Connection") -> [w1366]
    shift-right: ["silence"] -> _
    shift-left: FALSE ("silence") -> [w1365]
    stop <- w1353 stop-if-true
    # "If NOT Demo AND Sensor NOT connected AND NOT silence bit, then sound alarm"
    # "Reset the Silence bit to TRUE after a change in the connection state."
    # "ERROR COMM BEEPER"
    n585 = local read "Shutdown"() -> (w1352:bool)
    n586 = property on="Stop" class="Bool (strict)"() -> ("Value"=w1354:bool)  [unwired: 2 in, 2 out]
    n587 = local read "reset"() -> (w1355:bool)
    n588 = local read "senseConn"() -> (w1358:bool)
    n589 = Compound Arithmetic op=OR(w1352, w1355, w1354) -> (w1353:bool)
    n590 = local read "Level 0"() -> (w1360:T15)
    n591 = Not Equal?(x=w1358, y=w1366) -> (x != y?=w1362:bool)
    n592 = Unbundle(w1360) -> ("Demo Mode?"=w1359:bool)  [unwired: 1 out]
    n593 = Not Equal?(x=w1365, y="silence") -> (x != y?=w1363:bool)
    n594 = case shown="False" w1363 {
      tunnel: [w1369 FALSE] -> w1361
      tunnel: w1362 -> [w1370 _]
      tunnel: w1357 -> [w1367 _]
      frame False {
        n595 = Select(t=TRUE, s=w1370, f=w1367) -> (s? t:f=w1369:bool)
      }
      frame True {
      }
    }
    n596 = Compound Arithmetic op=AND(invert w1359, w1358, w1357) -> (w1356:bool)
    n597 = case shown="False" w1356 {
      frame False {
      }
      frame True {
        n598 = call <vilib>:"Beep.vi"("use system alert? (T)"=FALSE, "duration (msec)"=u32 500, "frequency (Hz)"=u32 440) -> ()  [unwired: 9 in]
      }
    }
  }
  n599 = node-c288(w28) -> (w20:errorcluster)
  n600 = Delete(path (use dialog)=w3) -> ()  [unwired: 4 in, 3 out]
  n601 = Select(t=w26, s=w26, f=w20) -> (s? t:f=w30:errorcluster)
  n602 = flat-sequence {
    tunnel: w30 -> [_]
    frame #0 {
      n603 = local read "reset"() -> (w1377:bool)
      n604 = case shown="False" w1377 {
        frame False {
          n605 = local write "reset"(FALSE ("Stop Button")) -> ()
          n606 = property on="Stop" class="Bool (strict)"("Value"=FALSE) -> ()  [unwired: 2 in, 2 out]
          n607 = local read "Shutdown"() -> (w1378:bool)
          n608 = case shown="False" w1378 {
            frame False {
              n609 = disable-structure shown="Default" {
                frame condition #0 (active) {
                }
                frame condition #1 {
                  n610 = control-ref of="This VI"() -> (w1381:refnum<vi>)
                  n611 = invoke class="VI" method="FP.Close"(reference=w1381) -> ()  [unwired: 2 in, 3 out]
                }
              }
            }
            frame True {
              n612 = call "WMI Reboot.vi"("Method"=enum16{"Reboot", "Shutdown"}."Shutdown") -> ()  [unwired: 10 in, 1 out]
            }
          }
        }
        frame True {
          n613 = call "WMI Reboot.vi"() -> ()  [unwired: 11 in, 1 out]
        }
      }
    }
  }
